vi "ControlProgram5.4.vi"() -> ()   [LabVIEW 2016]
uses:
  <vilib>/Utility/error.llb/DialogType.ctl
  <vilib>/Utility/miscctls.llb/LVPoint32TypeDef.ctl
  <vilib>/DAQmx/write.llb/DAQmx Write (Digital Bool 1Line 1Point).vi
  <vilib>/DAQmx/create/channels.llb/DAQmx Create Channel (DO-Digital Output).vi
  <vilib>/platform/TimedLoop/XDataNode/XDataNode.xnode
  <vilib>/Platform/TimedLoop/XDataNode/nitl_modes.ctl
  <vilib>/Platform/TimedLoop/XDataNode/XDNodeRunTimeDep.lvlib
  <vilib>/Platform/TimedLoop/XDataNode/wakeup.ctl
  <vilib>/Platform/TimedLoop/XDataNode/timing_clust.ctl
  <vilib>/DAQmx/create/channels.llb/DAQmx Create Channel (AI-Voltage-Basic).vi
  <vilib>/DAQmx/create/channels.llb/DAQmx Create Channel (AO-Voltage-Basic).vi
  <vilib>/DAQmx/write.llb/DAQmx Write (Analog 1D DBL NChan 1Samp).vi
  <resource>/objmgr/daqmx.rc
  <vilib>/Analysis/NI_AALBase.lvlib
  <vilib>/Analysis/baseanly.llb/Mean (DBL).vi
  <vilib>/Instr/_visa.llb/VISA Configure Serial Port (Instr).vi
  <vilib>/DAQmx/read.llb/DAQmx Read (Analog 2D DBL NChan NSamp).vi
  <vilib>/Utility/inputDevices.llb/closeMouse.vi
  <vilib>/Utility/inputDevices.llb/mouseAcquire.vi
  <vilib>/DAQmx/configure/timing.llb/DAQmx Timing (Sample Clock).vi
panel:
  out "Flush Sample Start Time":u32=46318105
  out "Sample flush time (s)":dbl=60.0
  in  "Inject Sample":bool
  out "Chart Freq (Hz)":dbl=500.0
  out "Cal values":T1={"AX alpha"=672.9952101249002, "BX alpha"=822.8320399167465, "AX kappa"=0.3432739170419873, "BX kappa"=0.22087046979741862, "AX offset"=-0.002065833400375715, "BX offset"=0.010483360643544744, "AY alpha"=702.0654168010462, "BY alpha"=773.6701766674906, "AY kappa"=0.33643150106915, "BY kappa"=0.2444549177225145, "AY offset"=-0.1177594339643395, "BY offset"=0.06470506082263472}
  in  "Inject Pump 1":bool
  in  "Inject Pump 2":bool
  in  "Tab Control 2":T2(tab)
  in  "Force FB script":bool
  in  "Got ADig bead":bool
  in  "Move Cap. 2 (ADig Top)":bool
  in  "Dump beads":bool
  in  "Got DNA bead":bool
  in  "Flow on\ncap 2?":bool=TRUE
  in  "Flow on\ncap 1?":bool=TRUE
  in  "Flow on\ndump?":bool=TRUE
  in  "Delta after tether":dbl=3.2
  in  "TA Cancel Save?":bool
  in  "Min fish\ndelta (V)":dbl=2.8 min=0.0 max=10.0 step=0.1
  in  "Max fish\ndelta (V)":dbl=3.8 min=0.0 max=10.0 step=0.1
  in  "Fish Speed (ms)":i32=3000
  in  "Wait (ms)":i32=1500
  in  "# attempts":dbl=15.0
  in  "Cutoff force (pN)":dbl=5.0
  in  "Raster after\n tether?":bool=TRUE
  out "Tether":bool
  out "Attempt #":i32
  in  "Flow on\nwhile fish?":bool=TRUE
  in  "Flow on\nafter raster?":bool=TRUE
  in  "Offset @ Delta (V)":dbl=4.0
  in  "Cal @ Delta (V)":dbl=5.0
  in  "Cal stage position":i32=3
  in  "Conv Y (nm/V)":dbl=505.7
  in  "Conv X (nm/V)":dbl=891.5
  out "Cal Final Sampling Rate":dbl=125000.0
  in  "Cal Averaging":i32=1
  in  "Wait before dip (s)":dbl=3.0
  in  "Start dipping after?":bool
  in  "Start trap delta (V)":dbl=3.85
  in  "Cancel dwell":bool
  in  "Pause dwell":bool
  in  "Return position":dbl=3.0
  in  "Dip duration":dbl=15.0
  in  "Dip position":dbl=4.0
  in  "Dip":bool
  out "Dip time":i32
  in  "Stop":bool=TRUE
  in  "?":T3(tab)
  in  "Save N sets":bool
  in  "N sets":i32=200
  in  "Cal sets to save":i32=500
  in  "Reset data stream":bool
  out "Buffer Overflow":bool
  out "Stage moving":bool
  in  "Comment":string
  in  "Raster scan":bool
  out "Saving":bool
  in  "Save cal":bool
  in  "Save Data":bool
  in  "Stop saving":bool
  out "Calibrating":bool
  out "Progress":dbl(slide) scale=0.0..100.0
  in  "Read Cal":bool
  in  "Fish":bool
  in  "Averaging Number":i32=1250
  out "Final Sampling Rate":dbl=100.0
  in  "Trap position":cluster{"X":dbl, "Y":dbl}={"X"=6.4, "Y"=1.35}
  in  "Trap delta":dbl=5.0 min=0.0 max=10.0 step=0.1
  in  "Fixed X":dbl=1.4
  in  "Fixed Y":dbl=1.35
  in  "Shutter 1 (B)":bool=TRUE
  in  "Shutter 2 (A)":bool=TRUE
  in  "Pulling direction":bool
  out "Raster scanning...":bool
  out "Current file name":path=path "D:/data/151111/151111_000.dat"
  in  "AX alpha":dbl=672.9952101249002 format="%#_3p"
  in  "BX alpha":dbl=822.8320399167465 format="%#_3g"
  in  "AX kappa":dbl=0.3432739170419873 format="%#_3g"
  in  "BX kappa":dbl=0.22087046979741862 format="%#_3g"
  in  "AX offset":dbl=-0.002065833400375715 format="%#_3g"
  in  "BX offset":dbl=0.010483360643544744 format="%#_3g"
  in  "AY alpha":dbl=702.0654168010462 format="%#_3g"
  in  "BY alpha":dbl=773.6701766674906 format="%#_3g"
  in  "AY kappa":dbl=0.33643150106915 format="%#_3g"
  in  "BY kappa":dbl=0.2444549177225145 format="%#_3g"
  in  "AY offset":dbl=-0.1177594339643395 format="%#_3g"
  in  "BY offset":dbl=0.06470506082263472 format="%#_3g"
  out "Buffer status":u8(slide) scale=0.0..100.0
  in  "dump spot":string="Dump beads spot"
  in  "up flow spot":string="Upper flow spot"
  in  "low flow spot":string="Lower flow spot"
  in  "up cap":string="Upper capillary (ADig beads)"
  in  "bottom cap":string="Lower capillary (DNA beads)"
  in  "Move to Position 5":bool
  in  "Set Position 5":bool
  in  "Saved stage positions":dbl[][](array[numeric])=[[1.0, 0.0, 0.0, 0.0], [2.0, -0.10561, -3.22524, -0.0041], [3.0, 0.5, -0.73974, 0.0], [4.0, 0.5, -2.1978, 0.0], [5.0, 0.5, -2.63158, -0.02256]]
  in  "Set Position 2":bool
  in  "Move to Position 2":bool
  in  "Set Position 1":bool
  in  "Move to Position 1":bool
  in  "Set Position 4":bool
  in  "Move to Position 4":bool
  in  "Set Position 3":bool
  in  "Move to Position 3":bool
  out "Stage error":errorcluster
  in  "Clear Volume":bool
  out "Sample Flush Meter":u8(slide) scale=0.0..100.0
  out "Flushing Sample":bool
  in  "Flush Sample":bool
  in  "Normal \nRate (ul/hr)  3":dbl=100.0
  in  "Normal \nVolume (ul) 3":dbl=400.0
  in  "Normal \nVolume (ul) 2":dbl
  in  "Normal \nRate (ul/hr)":dbl
  in  "Normal \nVolume (ul)":dbl
  in  "Flush\nRate (ul/min)":dbl
  in  "Flush\nVolume (ul)":dbl
  in  "Flush \nRate (ul/min)  2":dbl
  in  "Flush Pump 2":bool
  in  "Flush\nVolume (ul)  2":dbl
  in  "Flush Pump 1":bool
  in  "Normal \nRate (ul/hr)  2":dbl
  in  "Write Wait":i32=1000
  in  "Flush \nRate (ul/min)  3":dbl=100.0
  in  "Flush\nVolume (ul)  3":dbl=100.0
  out "error out":errorcluster
  in  "Use Mouse to Move Trap?":bool
  in  "Pause Mouse/Mirror Connection":bool
  out "Reference Voltage":cluster{dbl, dbl}={0.0, -0.0}
  out "Saved voltage":cluster{dbl, dbl}={5.766666666666665, 1.45}
  out "Real Coordinates":cluster{"Horizontal":i32, "Vertical":i32}={"Horizontal"=897, "Vertical"=-1271}
  out "CoordinatesMousePressed":T4
  out "Sum error":dbl(knob) scale=-1.0..1.0
  out "Trap sep":waveform(dbl)[](graph)=[{"t0"=timestamp(11.689999999999795 s since 1904-01-01), "dt"=0.002, "Y"=[4456.58918693872, 4456.558162103858, 4456.805211715709, 4456.946547075299, 4456.750056453253], "attributes"=variant("NI_ChannelName"=variant(string "T2 X"))}, {"t0"=timestamp(11.689999999999795 s since 1904-01-01), "dt"=0.002, "Y"=[3.6580154856012372, 3.6801758901442225, 3.6782205603924463, 3.7068987310363912, 3.7544784232311184], "attributes"=variant("NI_ChannelName"=variant(string "T2 Y"))}]
  in  "Set reading to\nsetpoint":bool
  in  "Offset Y (nm)":dbl format="%0.2f"
  in  "Offset X (nm)":dbl format="%0.2f"
  in  "Remove offsets":bool
  in  "Force Feedback":bool
  out "Feedback Output Voltage 2":cluster{dbl, dbl} {"?" format="%#_4g"; "?" format="%#_4g"}
  in  "Max value X":dbl=10.0 format="%.1f"
  in  "Min value X":dbl format="%0.1f"
  in  "Max value Y":dbl=10.0 format="%.1f"
  in  "Min value Y":dbl format="%.1g"
  in  "Offset":cluster{"Off Y":dbl, "Off X":dbl}={"Off Y"=1.5, "Off X"=0.17}
  in  "Setpoint voltage":cluster{"SP Y":dbl, "SP X":dbl}={"SP Y"=0.6, "SP X"=0.0}
  in  "Feedback const":T5={"Ki_B_Y"=0.5, "Ki_B_X"=0.0, "Kp Y"=1.0, "Kp X"=0.0}
  out "Mean Trap Pos X 2 (nm)":dbl=4456.729832857368 format="%0.2f"
  out "Mean Trp Pos Y 2 (nm)":dbl=3.6955578180810833 format="%0.2f"
  out "T2 X RMS (A)":dbl=1.4304414731965482 format="%0.2f"
  out "T2 Y RMS (A)":dbl=0.33307251334057864 format="%0.2f"
  in  "Scan range (nm)":dbl=500.0
  in  "Scan speed (nm/s)":dbl=100.0 min=0.0 max=100.0
  in  "Step size (nm)":dbl=1.0
  in  "Save scans":bool=TRUE
  in  "# scans":i32=1
  in  "Load param":bool
  in  "Scan Parameters":T6(array[cluster])=[{"Label"="Offset", "Max delta 2"=3.8, "Start delta 2"=2.4, "Speed (ms) 2"=10000, "# scans 2"=1}]
  in  "Trap delta\nafter":dbl=3.6
  in  "Stop raster":bool
  out "Scan range (V)":dbl=0.5608524957936063
  out "Scan steps (mirror)":u64=500
  out "Scan increment (V)":dbl=0.0011217049915872126
  out "Time per step (ms)":dbl=10.0
  out "Total raster time (s)":dbl=10.0
  out "N sets to be saved":dbl=1000.0
  out "Continue to display?":bool
  out "Video Error":errorcluster
  in  "# Samples/channel (in)":i32=40000 format="%.2f"
  out "Buffer size\n(Samples/channel)":u32=511
  out "DAQ rate\n(Samples/s)":dbl=125000.0 format="%#_6p"
  out "# Samples/channel":i32=1250
  out "# Samples/channel/s":dbl=100.0
  out "AvailSampPerChan":u32=6
  out "Data update period (s/set)":dbl=0.01 format="%#_6p"
  out "AvailSampPerChan 2":u32=81
  in  "PC samp per channel":i32=1000
  in  "Sampling Rate":dbl=125000.0 format="%0.0p"
  in  "DAQ Rate2":dbl=1000000.0 format="%#_6p"
  out "Data period (s)":dbl=8e-06 format="%#_6p"
  in  "Tether break\nforce (pN)":dbl=1.0
  in  "Path":path=path "D:/data"
  in  "Save file index":dbl
  out "Mirror task":refnum<k21>
  in  "HWP1":string="Half waveplate 1: differential trap power"
  in  "HWP0":string="Half waveplate 0: total trap power"
  in  "Move 1":bool
  in  "\"Degrees\" 1":dbl
  in  "Move 0":bool
  in  "\"Degrees\" 0":dbl
  out "Chamber":T7(plugin-control)
  out "Deflection":T4
  in  "Sampling Rate":dbl=125000.0 format="%0.2f"
  in  "Averaging Number":i32=12500
  in  "DAQ Rate":dbl=1000000.0
  out "Final Sampling Rate":dbl
  in  "Tab Control":T8(tab)
  in  "Downsamp\nfact":dbl=250.0
  out "Bead sep":waveform(dbl)[](graph)=[{"t0"=timestamp(11.689999999999795 s since 1904-01-01), "dt"=0.002, "Y"=[63.31490687968469, 63.634813997558965, 62.7925550739979, 64.07278834927408, 63.99586325693618], "attributes"=variant("NI_ChannelName"=variant(string "T2"))}, {"t0"=timestamp(11.689999999999795 s since 1904-01-01), "dt"=0.002, "Y"=[176.64692461381742, 177.9358681148926, 177.1161917603868, 176.2271334264959, 177.42702158777735], "attributes"=variant("NI_ChannelName"=variant(string "T1"))}]
  out "Force (pN)":waveform(dbl)[](graph)=[{"t0"=timestamp(11.689999999999795 s since 1904-01-01), "dt"=0.002, "Y"=[21.359049199870693, 21.47379015932484, 21.184451058658276, 21.619260543462246, 21.59231529352076], "attributes"=variant("NI_ChannelName"=variant(string "T2"))}, {"t0"=timestamp(11.689999999999795 s since 1904-01-01), "dt"=0.002, "Y"=[41.69409117180523, 41.983023709759294, 41.835566815034625, 41.592717375287485, 41.869370537040446], "attributes"=variant("NI_ChannelName"=variant(string "T1"))}]
  out "Mean force (pN)":dbl=31.62036358637639 format="%0.2f"
  out "Force noise (pN)":dbl=0.0949326369135985 format="%0.2f"
  out "Mean Bead Sep\n(nm)":dbl=120.31640670608219 format="%0.2f"
  out "Bead Sep Noise\n(A)":dbl=3.5979970492756337 format="%0.2f"
  out "PSD 2":cluster{dbl[], dbl[]}(graph)
  out "PSD 1":cluster{dbl[], dbl[]}(graph)
  out "PSD 1 Sum":dbl(slide) scale=0.0..10.0
  out "PSD 2 Sum":dbl(slide) scale=0.0..10.0
  in  "Start":bool
  out "All signals":waveform(dbl)[](graph)=[{"t0"=timestamp(11.689999999999795 s since 1904-01-01), "dt"=0.002, "Y"=[-1.299883075629171, -1.2973358725298367, -1.2936816089521828, -1.3024318472699856, -1.301891455018789], "attributes"=variant("NI_ChannelName"=variant(string "A y"))}, {"t0"=timestamp(11.689999999999795 s since 1904-01-01), "dt"=0.002, "Y"=[-0.23397256158648597, -0.24766722604162583, -0.2351063720288359, -0.2449917640631612, -0.24277750809631515], "attributes"=variant("NI_ChannelName"=variant(string "A x"))}, {"t0"=timestamp(11.689999999999795 s since 1904-01-01), "dt"=0.002, "Y"=[-0.7474367183534977, -0.752021809613988, -0.7569647451326695, -0.7437660589687638, -0.7496079628534502], "attributes"=variant("NI_ChannelName"=variant(string "B y"))}, {"t0"=timestamp(11.689999999999795 s since 1904-01-01), "dt"=0.002, "Y"=[-0.7679815477569002, -0.7778056271968022, -0.7612590927024251, -0.7662199857579963, -0.7730989233960032], "attributes"=variant("NI_ChannelName"=variant(string "B x"))}, {"t0"=timestamp(11.689999999999795 s since 1904-01-01), "dt"=0.002, "Y"=[6.442881382091263, 6.440977653300508, 6.439989054505619, 6.439557267869424, 6.436601783511025], "attributes"=variant("NI_ChannelName"=variant(string "A sum"))}, {"t0"=timestamp(11.689999999999795 s since 1904-01-01), "dt"=0.002, "Y"=[6.405386825078533, 6.40147238948137, 6.401793329117672, 6.401977644095232, 6.397063010213611], "attributes"=variant("NI_ChannelName"=variant(string "B sum"))}, {"t0"=timestamp(11.689999999999795 s since 1904-01-01), "dt"=0.002, "Y"=[6.3989783364427595, 6.3989435357306315, 6.399220652513415, 6.399379189091754, 6.399158784580205], "attributes"=variant("NI_ChannelName"=variant(string "Trap x"))}, {"t0"=timestamp(11.689999999999795 s since 1904-01-01), "dt"=0.002, "Y"=[1.3572335682926662, 1.3572773895395378, 1.3572735229590518, 1.357330232808061, 1.3574243196029883], "attributes"=variant("NI_ChannelName"=variant(string "Trap y"))}]
  # "Bead Calibration"
  # "X"
  # "Y"
  # "Pump #1 Controls"
  # "Pump #2 Controls"
  # "Sample Pump Controls"
  # "Retract the pumps manually. Change it back to INFUSE when you're done. Suck it up, don't whine."
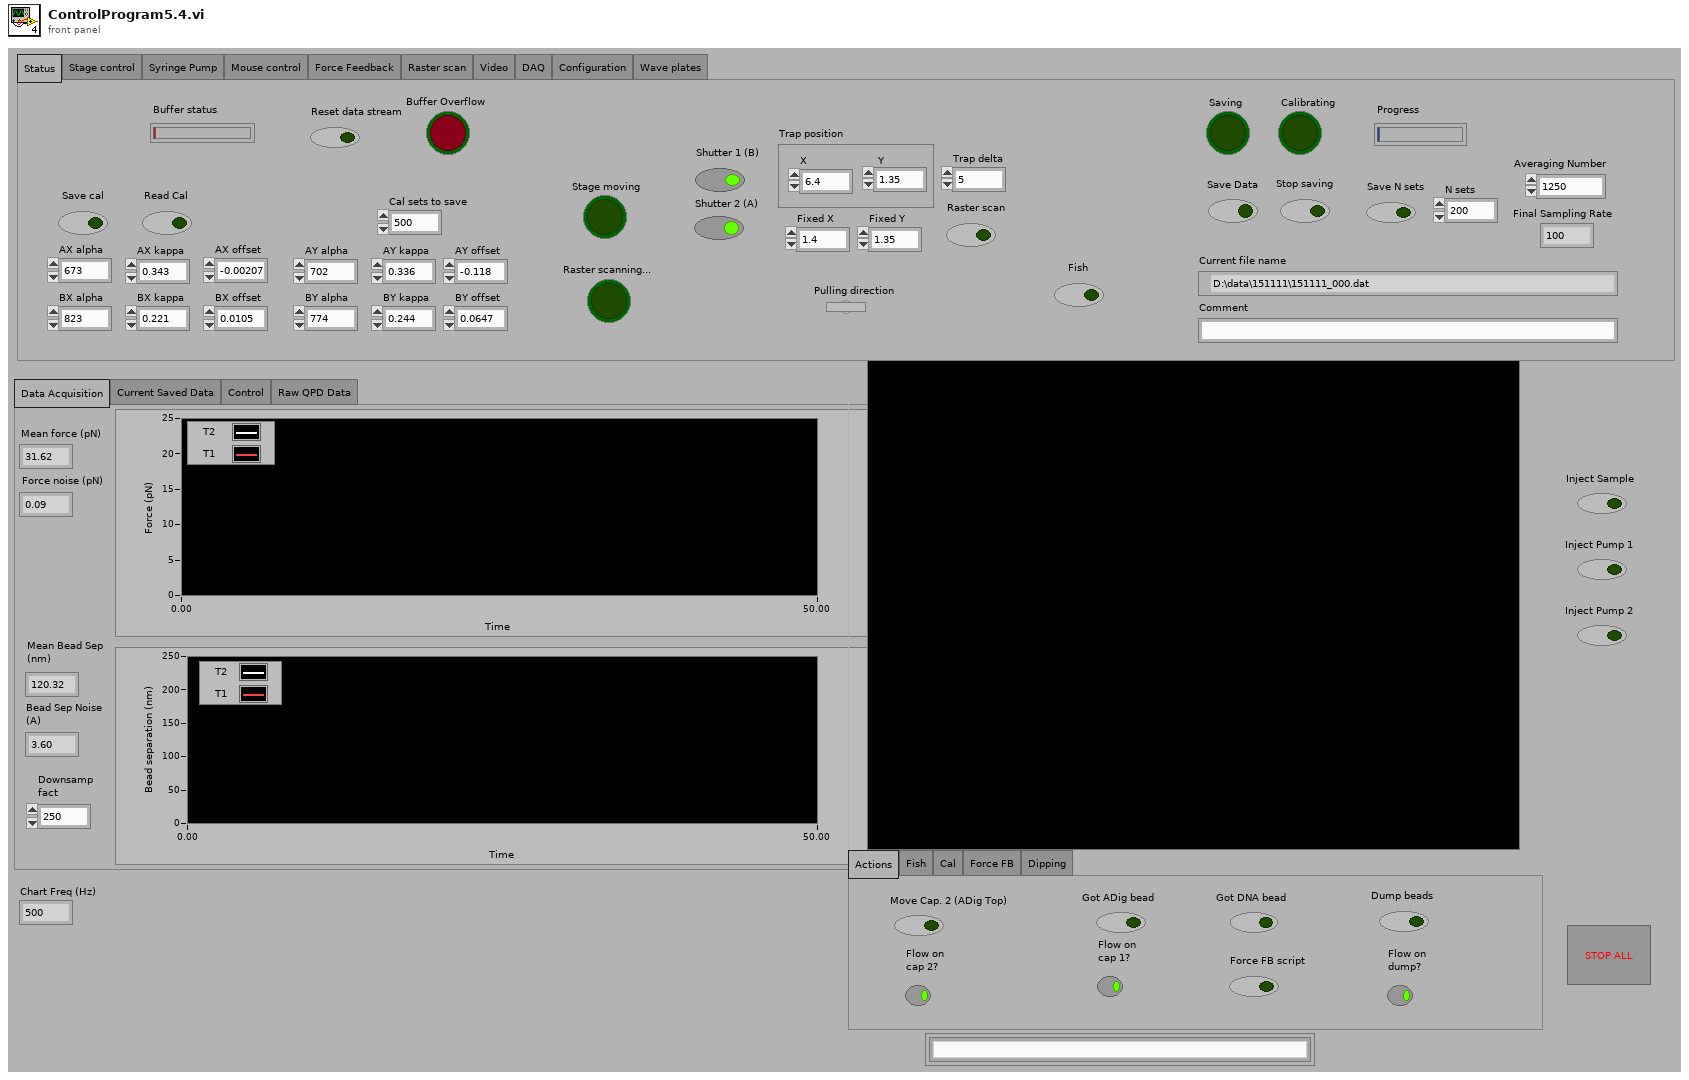
[diagram p1: front panel]
types:
  T1 = cluster{"AX alpha":dbl, "BX alpha":dbl, "AX kappa":dbl, "BX kappa":dbl, "AX offset":dbl, "BX offset":dbl, "AY alpha":dbl, "BY alpha":dbl, "AY kappa":dbl, "BY kappa":dbl, "AY offset":dbl, "BY offset":dbl}
  T2 = enum32{"Actions", "Fish", "Cal", "Force FB", "Dipping"}
  T3 = enum32{"Status", "Stage control", "Syringe Pump", "Mouse control", "Force Feedback", "Raster scan", "Video", "DAQ", "Configuration", "Wave plates"}
  T4 = typedef "LVPoint32TypeDef.ctl" = cluster{"Horizontal":i32, "Vertical":i32}
  T5 = cluster{"Ki_B_Y":dbl, "Ki_B_X":dbl, "Kp Y":dbl, "Kp X":dbl}
  T6 = cluster{"Label":string, "Max delta 2":dbl, "Start delta 2":dbl, "Speed (ms) 2":i32, "# scans 2":i32}[]
  T7 = typedef "IMAQ Image.ctl" = refnum<image>
  T8 = enum32{"Data Acquisition", "Current Saved Data", "Control", "Raw QPD Data"}
  T9 = enum16{"open", "replace", "create", "open or create", "replace or create", "replace or create with confirmation"}
  T10 = enum16{"big-endian, network order", "native, host order", "little-endian"}
  T11 = cluster{string, string, string, string, string, string, string, string}
  T12 = typedef "XDNodeRunTimeDep.lvlib/timing_clust.ctl" = cluster{"Expected End [f-1]":u64, "Actual End [f-1]":u64, "Finished Late? [f-1]":bool, "Expected End [i-1]":u64, "Actual End [i-1]":u64, "Finished Late? [i-1]":bool, "Expected Start [i]":u64, "Actual Start [i]":u64, "Expected Start [f]":u64, "Actual Start [f]":u64, "Source Name":string, "Structure Name":string, "Period":i64, "Deadline":i64, "Offset":i64, "Start":i64, "Priority":i32, "Timeout":i32, "Mode":T13, "Wakeup Reason":T14, "Error":errorcluster, "Source Type":string, "Secondary Source Type":string, "Global End Time":u64, "Global Start Time":u64, "Frame Duration":u64, "Iteration Duration":u64, "Assigned CPU":i32, "I/O Scan Engine Mode":u32}
  T13 = typedef "XDNodeRunTimeDep.lvlib/nitl_modes.ctl" = enum32{"No Change", "Process missed periods, maintain original phase", "Discard missed periods, maintain original phase", "Process missed periods, ignore original phase", "Discard missed periods, ignore original phase"}
  T14 = typedef "XDNodeRunTimeDep.lvlib/wakeup.ctl" = enum32{"Normal", "Aborted", "Asynchronous wakeup", "Timing source error", "Timed loop error", "Timeout"}
  T15 = typedef "DialogType.ctl" = u16
  T16 = cluster{"button 1":bool, "button 2":bool, "button 3":bool, "button 4":bool}
  T17 = cluster{"[0]":dbl, "[1]":dbl, "[2]":dbl, "[3]":dbl, "[4]":dbl, "[5]":dbl, "[6]":dbl, "[7]":dbl, "[8]":dbl, "[9]":dbl, "[10]":dbl, "[11]":dbl}
  T18 = cluster{"Label":string, "Max delta 2":dbl, "Start delta 2":dbl, "Speed (ms) 2":i32, "# scans 2":i32}
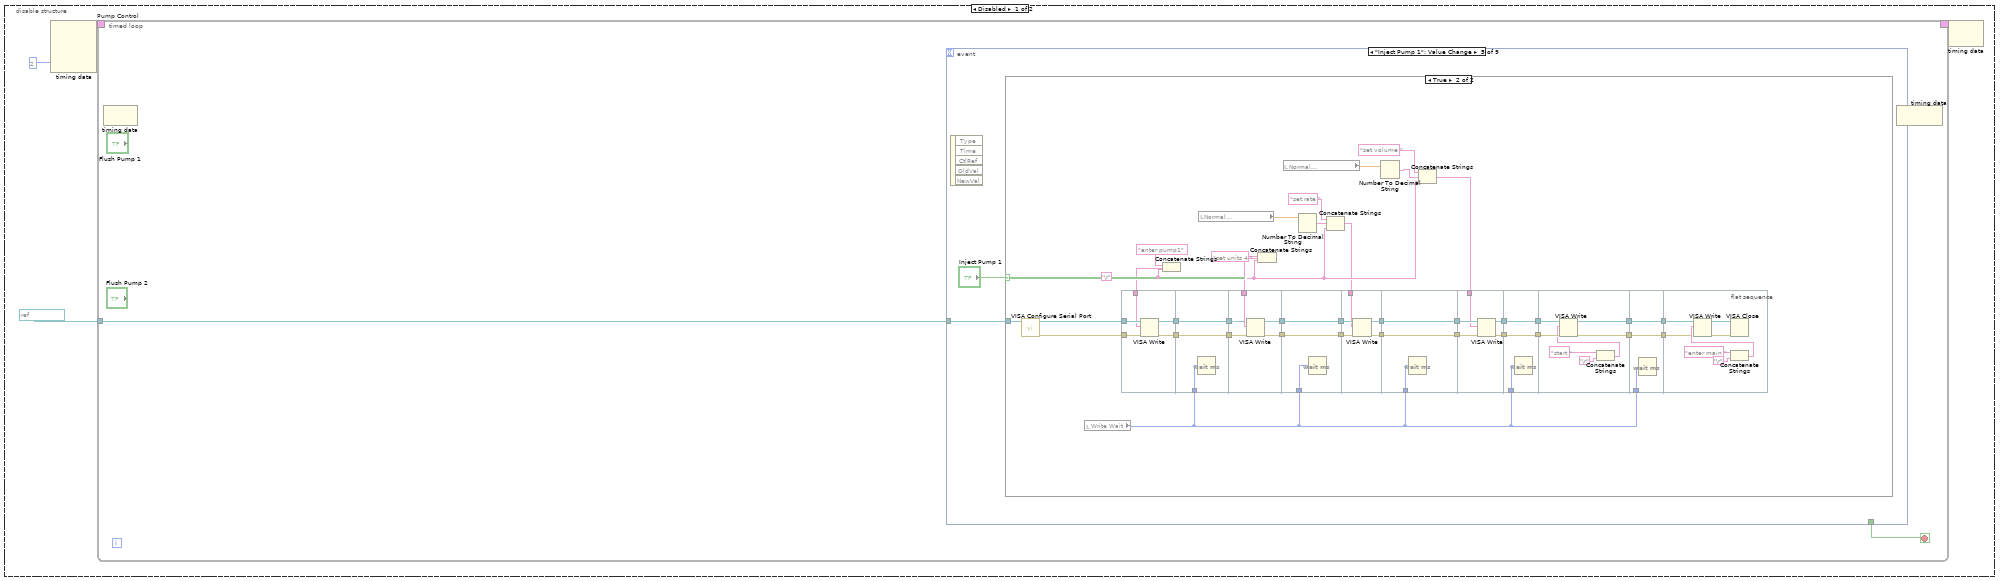
[diagram p2: hidden frame]
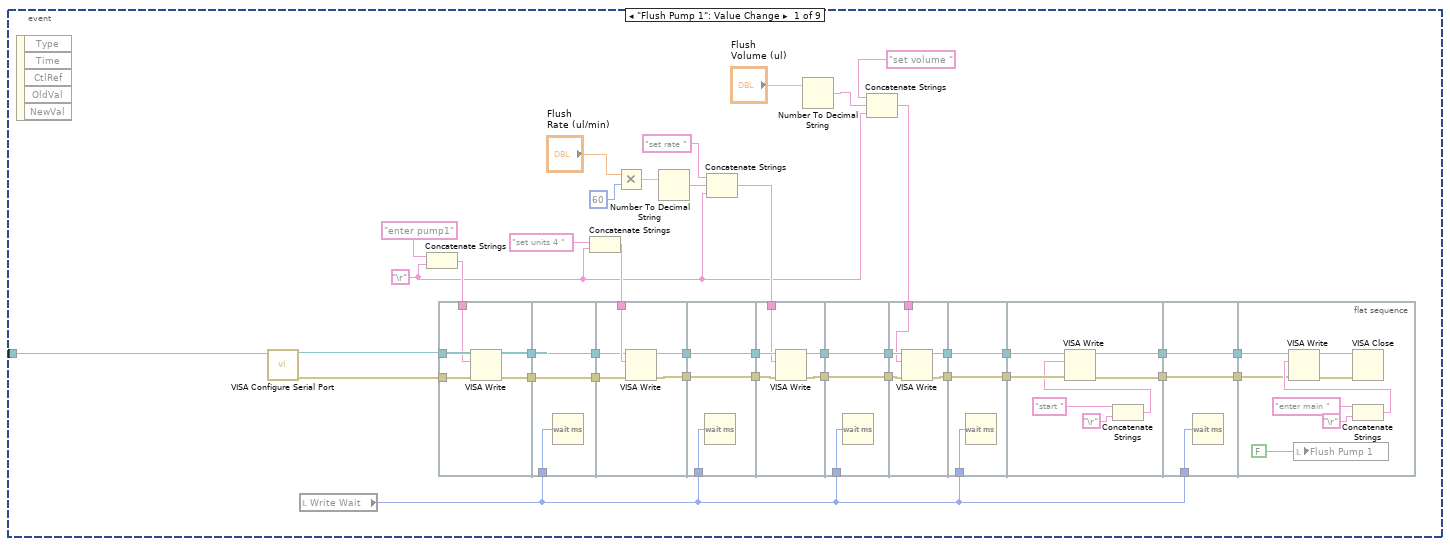
[diagram p3: hidden frame]
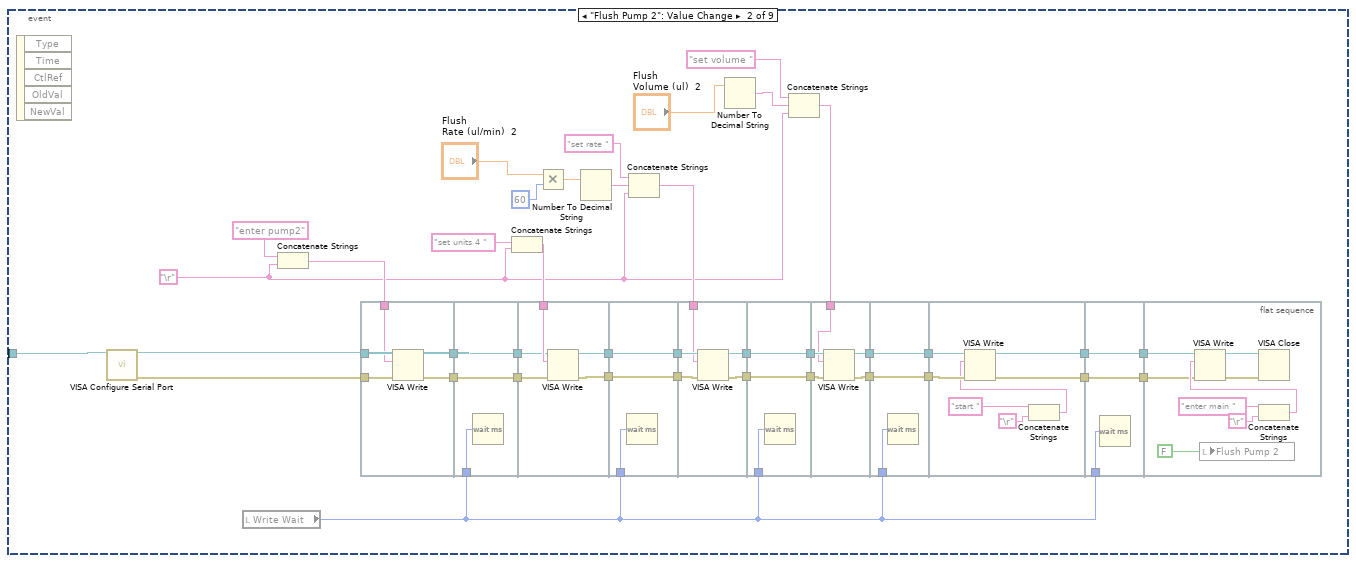
[diagram p4: hidden frame]
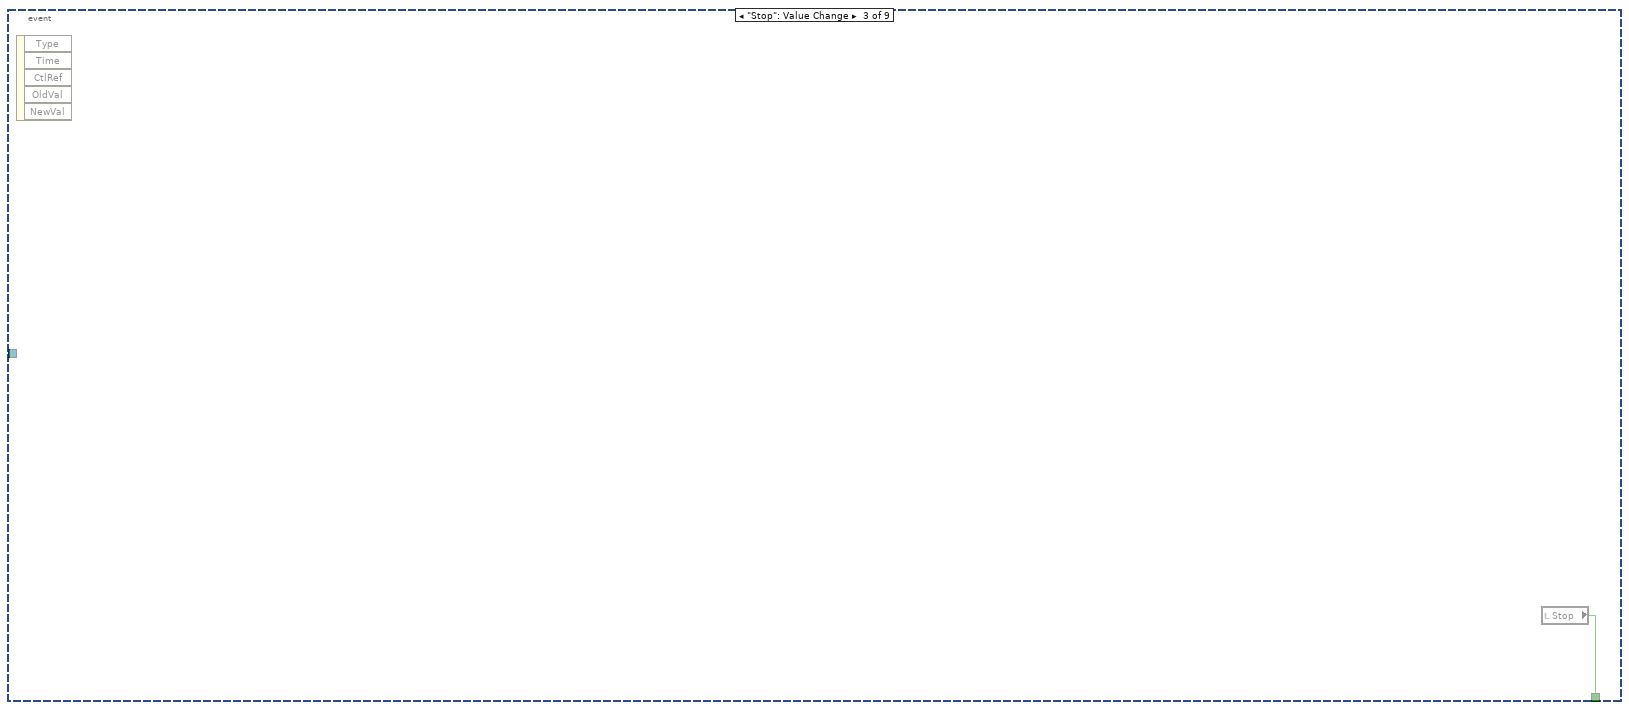
[diagram p5: hidden frame]
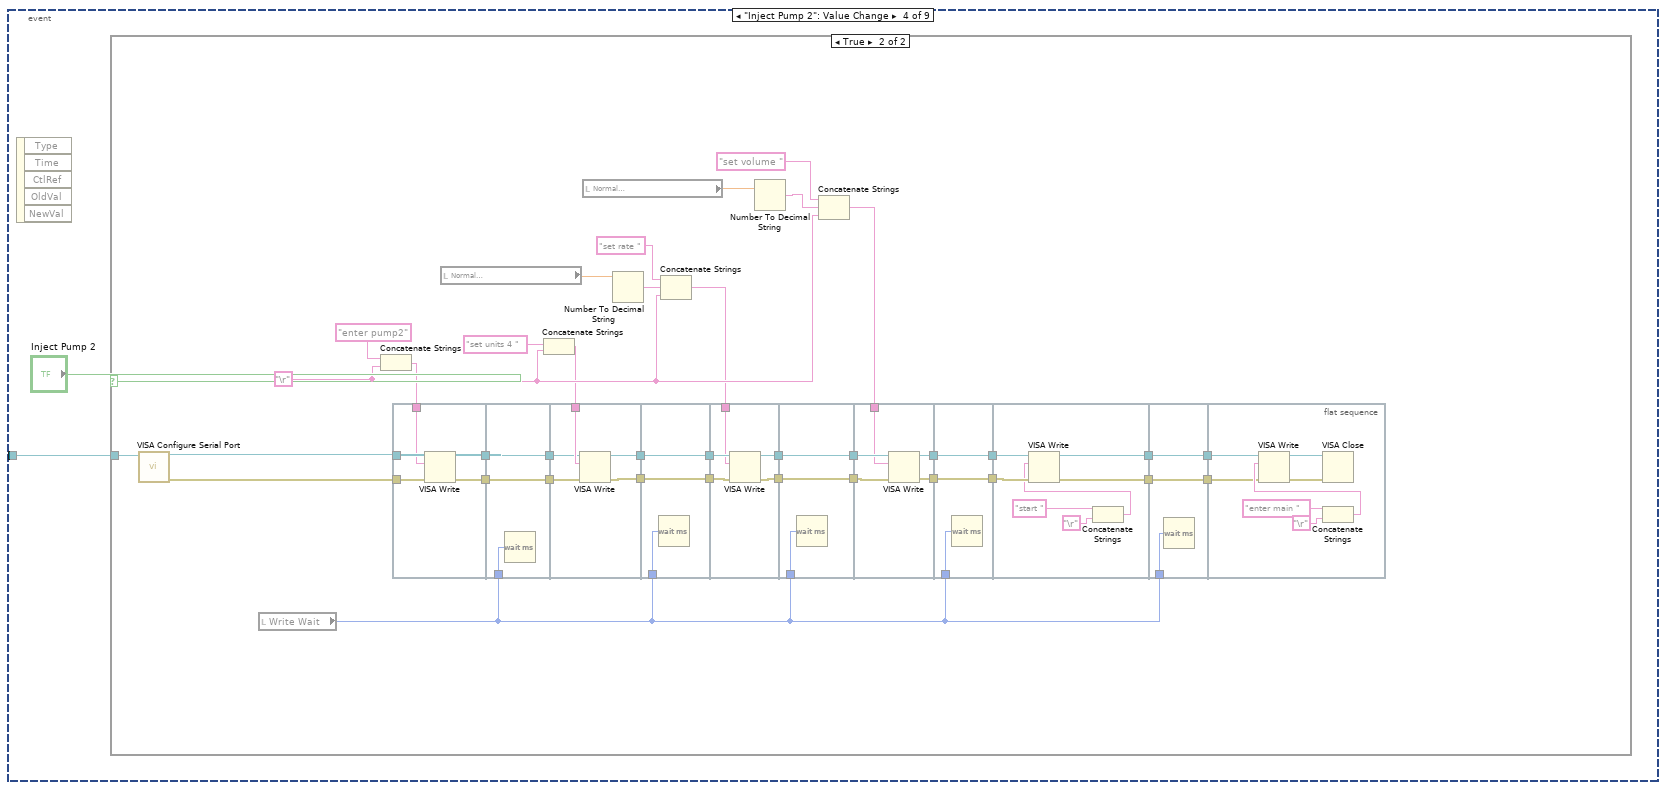
[diagram p6: hidden frame]
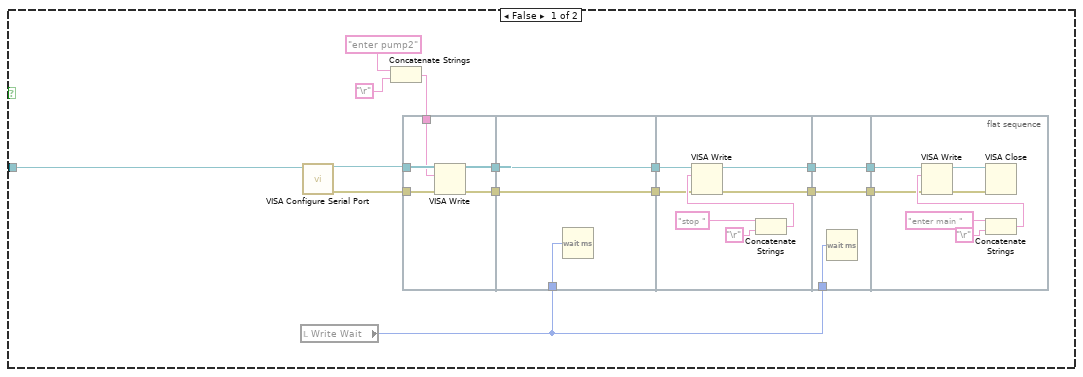
[diagram p7: hidden frame]
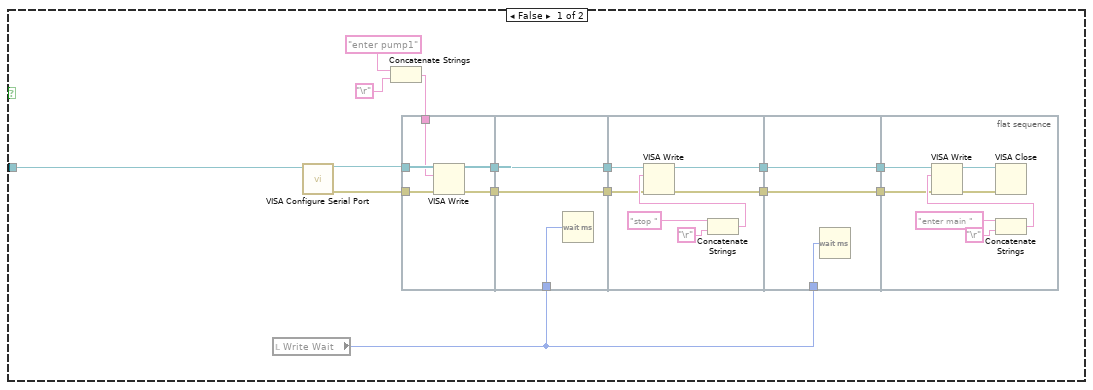
[diagram p8: hidden frame]
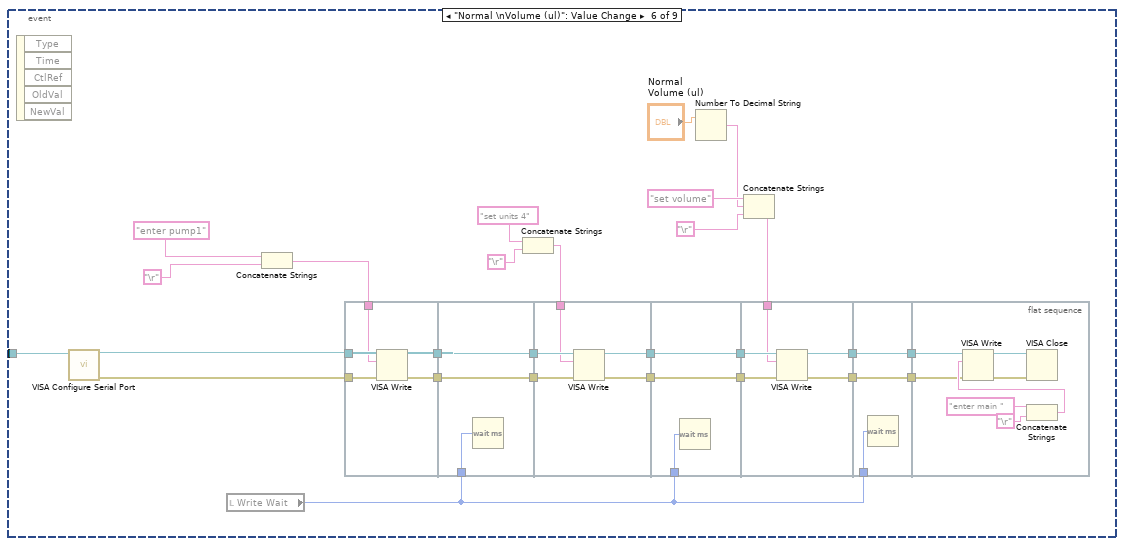
[diagram p9: hidden frame]
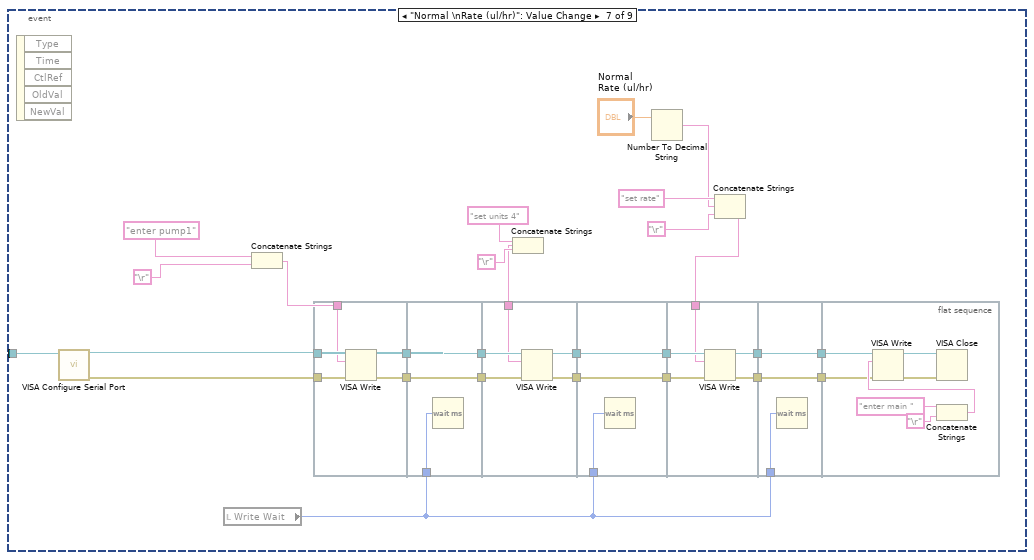
[diagram p10: hidden frame]
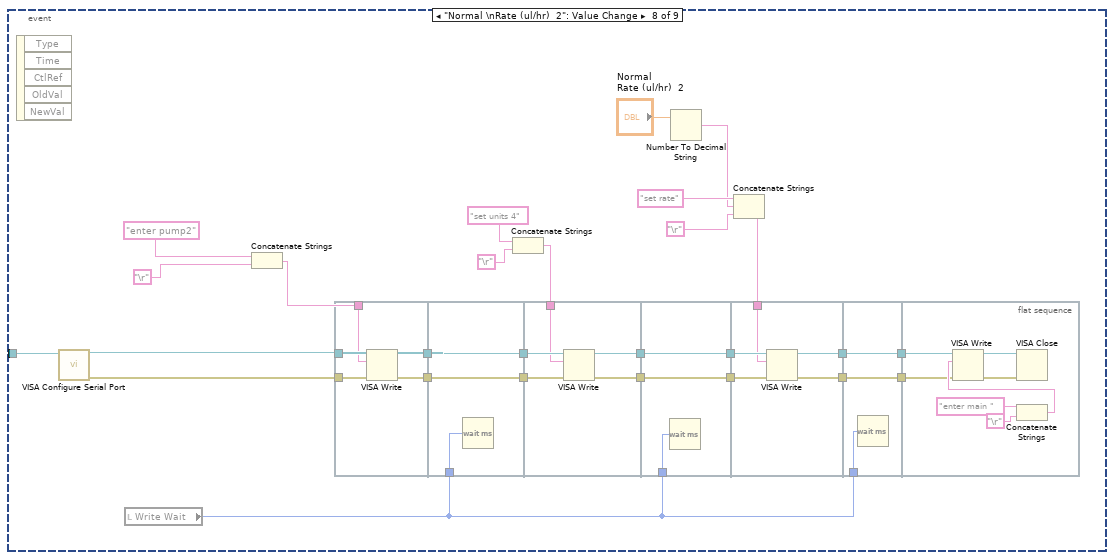
[diagram p11: hidden frame]
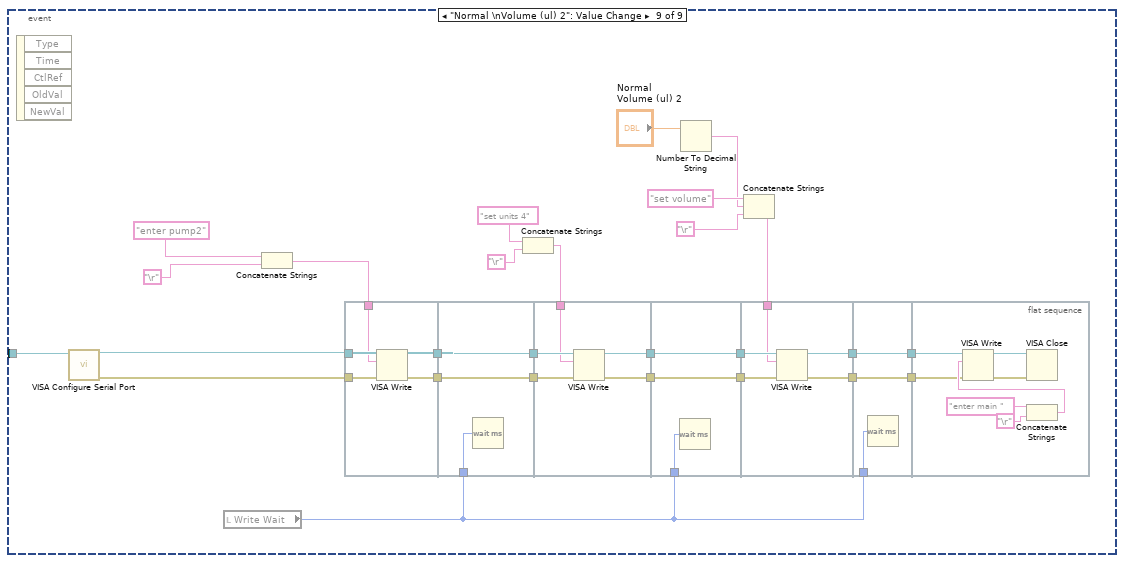
[diagram p12: hidden frame]
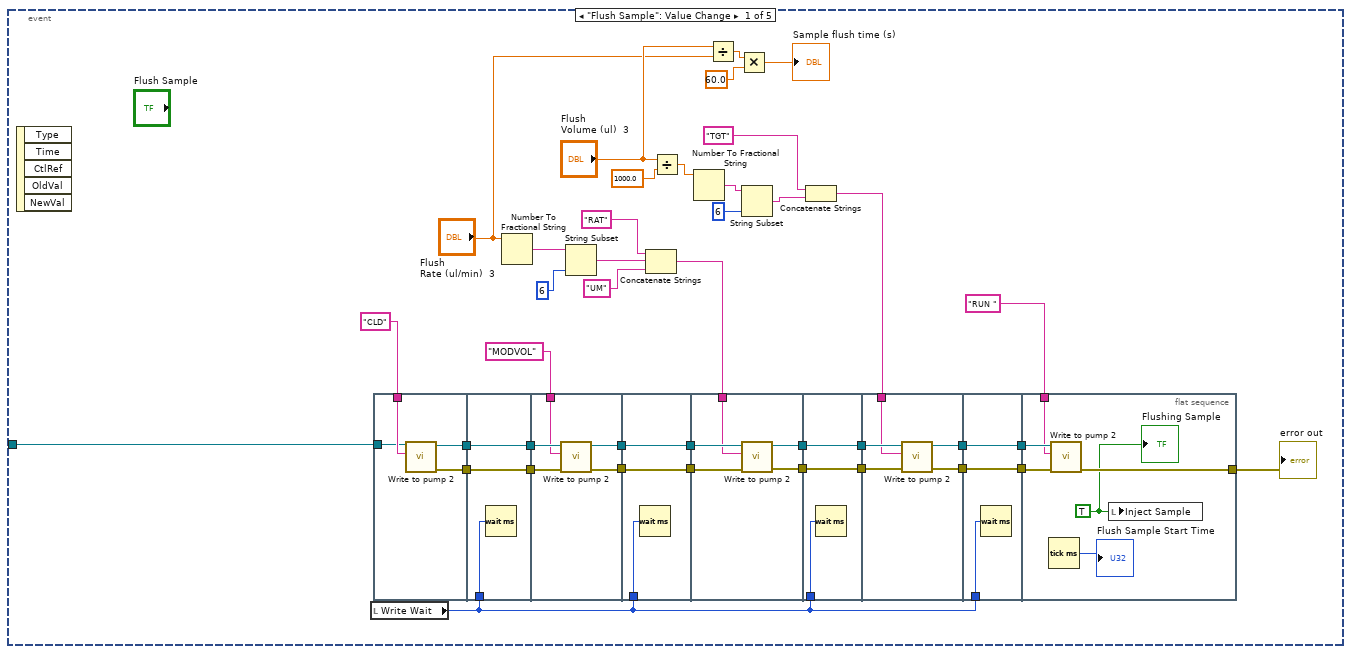
[diagram p13: hidden frame]
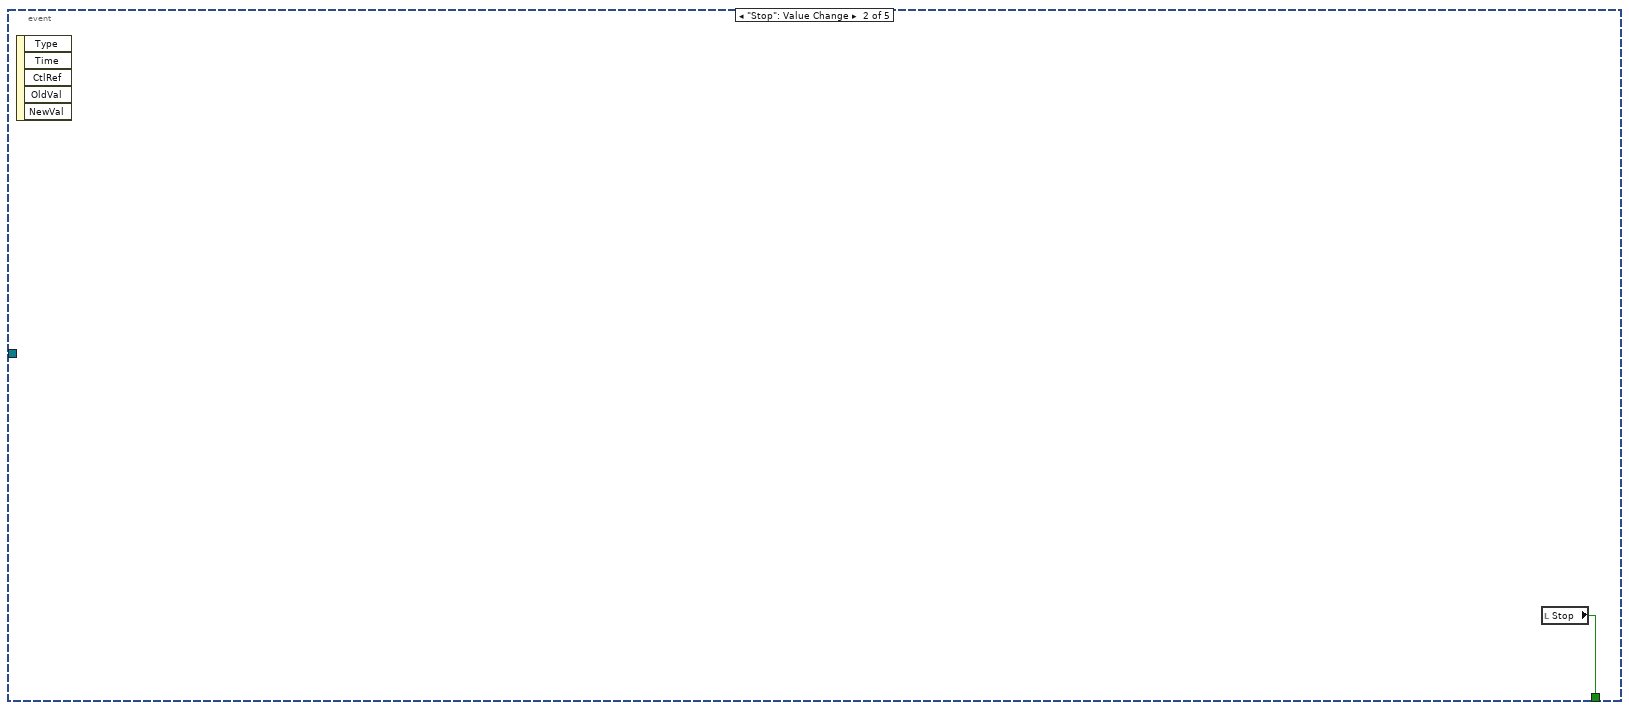
[diagram p14: hidden frame]
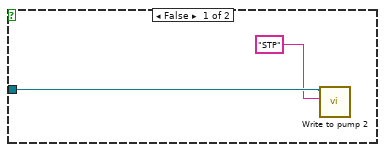
[diagram p15: hidden frame]
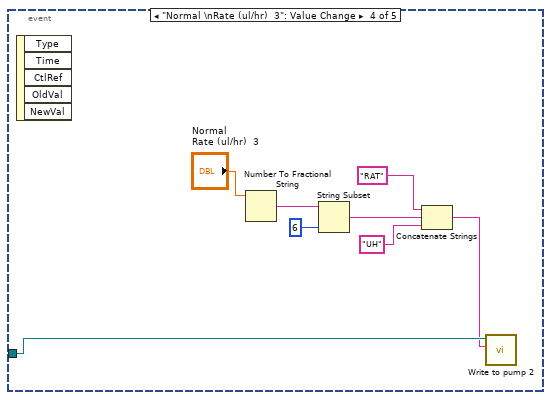
[diagram p16: hidden frame]
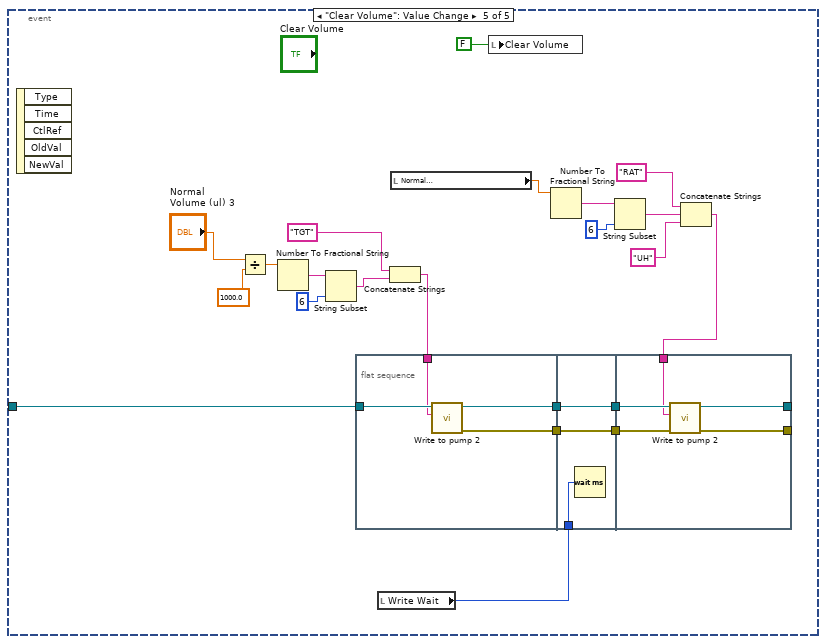
[diagram p17: hidden frame]
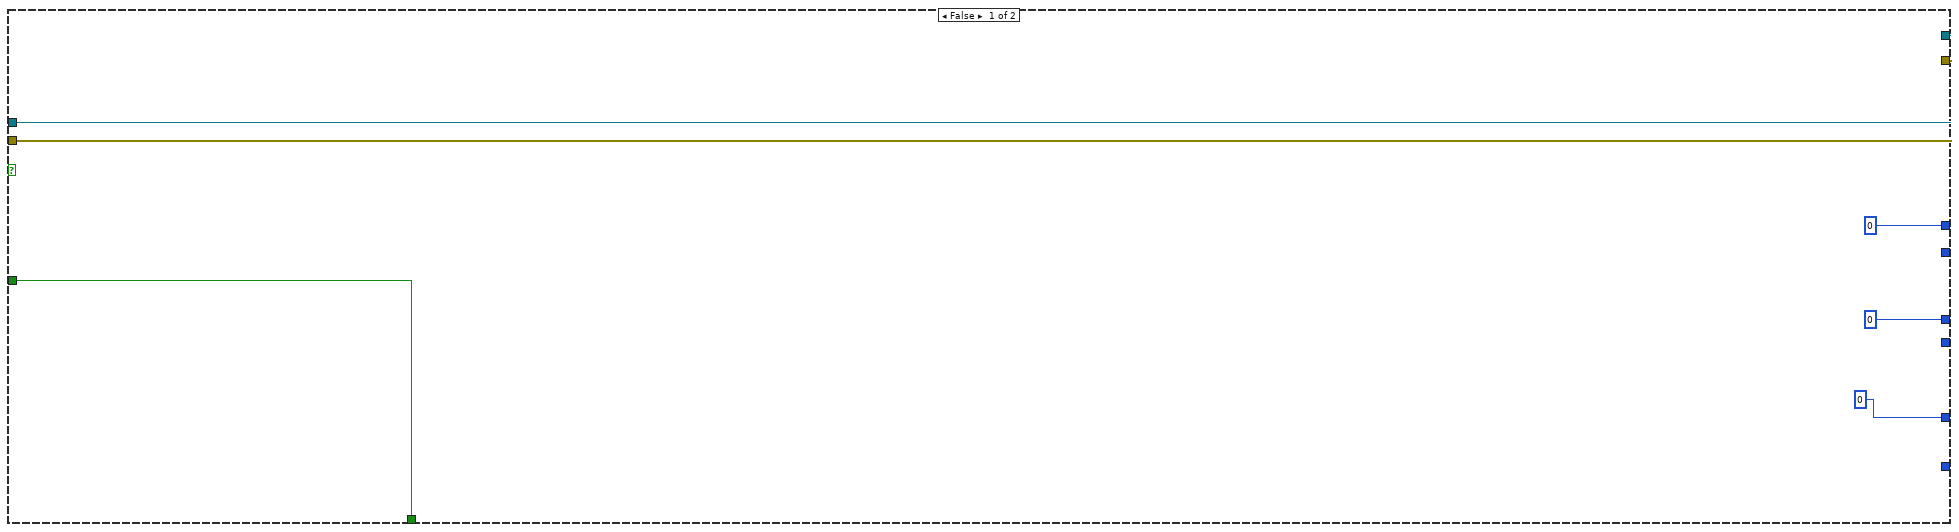
[diagram p18: hidden frame]
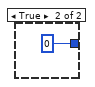
[diagram p19: hidden frame]
diagram:
  w42 = 10.0 ("Minimum Value")
  w43 = -10.0 ("Minimum Value")
  w45 = -2.0 ("Minimum Value")
  w46 = 2.0 ("Maximum Value")
  w71 = 10123 items=["Finite Samples"=10178, "Continuous Samples"=10123] ("sample mode")
  w92 = tag "Dev1/port2/line1"  # Shutter 2
  w95 = tag "Dev1/port1/line4"  # Shutter 1
  # "Create channels for movable mirror"
  # "Create channels for detectors"
  n1 = call-poly <vilib>:"DAQmx Create Virtual Channel.vi"("maximum value"=w46, "minimum value"=w45, "physical channels"=tag "Dev1/ai0" ("Physical Channel")) -> ("task out"=w47:refnum<k21>, "error out"=w70:errorcluster)  [unwired: 11 in]
  n2 = call-poly <vilib>:"DAQmx Create Virtual Channel.vi"("task in"=w47, "maximum value"=w46, "minimum value"=w45, "physical channels"=tag "Dev1/ai1", "error in"=w70) -> ("task out"=w68:refnum<k21>, "error out"=w67:errorcluster)  [unwired: 9 in]
  n3 = call-poly <vilib>:"DAQmx Create Virtual Channel.vi"("task in"=w68, "maximum value"=w46, "minimum value"=w45, "physical channels"=tag "Dev1/ai2", "error in"=w67) -> ("task out"=w59:refnum<k21>, "error out"=w58:errorcluster)  [unwired: 9 in]
  n4 = call-poly <vilib>:"DAQmx Create Virtual Channel.vi"("task in"=w59, "maximum value"=w46, "minimum value"=w45, "physical channels"=tag "Dev1/ai3" ("Physical Channel"), "error in"=w58) -> ("task out"=w44:refnum<k21>, "error out"=w64:errorcluster)  [unwired: 9 in]
  n5 = call-poly <vilib>:"DAQmx Create Virtual Channel.vi"("task in"=w44, "maximum value"=w42, "minimum value"=w43, "physical channels"=tag "Dev1/ai4", "error in"=w64) -> ("task out"=w62:refnum<k21>, "error out"=w61:errorcluster)  [unwired: 9 in]
  n6 = call-poly <vilib>:"DAQmx Create Virtual Channel.vi"("task in"=w62, "maximum value"=w42, "minimum value"=w43, "physical channels"=tag "Dev1/ai5", "error in"=w61) -> ("task out"=w57:refnum<k21>, "error out"=w56:errorcluster)  [unwired: 9 in]
  n7 = call-poly <vilib>:"DAQmx Create Virtual Channel.vi"("task in"=w57, "maximum value"=w42, "minimum value"=w43, "physical channels"=tag "Dev1/ai6", "error in"=w56) -> ("task out"=w51:refnum<k21>, "error out"=w49:errorcluster)  [unwired: 9 in]
  n8 = call-poly <vilib>:"DAQmx Create Virtual Channel.vi"("task in"=w51, "maximum value"=w42, "minimum value"=w43, "physical channels"=tag "Dev1/ai7", "error in"=w49) -> ("task out"=w50:refnum<k21>, "error out"=w48:errorcluster)  [unwired: 9 in]
  n9 = call-poly <vilib>:"DAQmx Timing.vi"("task/channels in"=w50, "sample mode"=w71, "samples per channel"="PC samp per channel", "rate"="Sampling Rate", "error in"=w48) -> ("task out"=w54:refnum<k21>, "error out"=w53:errorcluster)  [unwired: 9 in]
  n10 = call-poly <vilib>:"DAQmx Create Virtual Channel.vi"("maximum value"="Max value Y", "minimum value"="Min value Y", "physical channels"=tag "Dev1/ao1" ("Trap X Axis")) -> ("task out"=w39:refnum<k21>, "error out"=w41:errorcluster)  [unwired: 11 in]
  n11 = property class="DAQmx Timing"(reference=w54, error in=w53, "More:AI Convert:Rate"="DAQ Rate2") -> (reference out=w6:refnum<k21>, error out=w5:errorcluster, "SampClk.Rate"=→"DAQ rate\n(Samples/s)":dbl)
  n12 = call-poly <vilib>:"DAQmx Create Virtual Channel.vi"("task in"=w39, "maximum value"="Max value X", "minimum value"="Min value X", "physical channels"=tag "Dev1/ao0" ("Trap Y Axis"), "error in"=w41) -> ("task out"=w30:refnum<k21>, "error out"=w29:errorcluster)  [unwired: 9 in]
  "Mirror task" <- w30
  n13 = property class="DAQmx Buffer"(reference=w6, error in=w5) -> (reference out=w3:refnum<k21>, error out=w2:errorcluster, "Input.OnbrdBufSize"=→"Buffer size\n(Samples/channel)":u32)
  n14 = call <vilib>:"DAQmx Start Task.vi"("task/channels in"=w3, "error in"=w2) -> ("task out"=w31:refnum<k21>)  [unwired: 12 in, 1 out]
  n15 = while {
    tunnel: [w123] -> w77
    tunnel: [w323] -> w78
    tunnel: [w121] -> w76
    tunnel: [w435] -> w73
    tunnel: w31 -> [w136]
    tunnel: w30 -> [w431]
    tunnel: w29 -> [w436]
    stop <- w435 stop-if-true
    w167 = "NI_ChannelName" ("name")
    w243 = -1
    # "Scan # counter"
    # "DAQ loop iteration\ncounter (for timing)"
    # "Step counter"
    # "Force feedback"
    # "Raster scan"
    # "Rewire everything"
    # "Invert these because changed\nfrom PSD to QPD"
    # "Trap Y"
    # "Trap X"
    # "Convert to\npN"
    # "Convert to\nnm"
    # "Subtract\noffset"
    # "Normalize by\nsum"
    # "B sum"
    # "BX"
    # "BY"
    # "AX"
    # "AY"
    # "A sum"
    # "Close files when done saving"
    n16 = property class="DAQmx Read"(reference=w136) -> (reference out=w135:refnum<k21>, "AvailSampPerChan"=→"AvailSampPerChan 2":u32)  [unwired: 1 in, 1 out]
    n17 = local read "Averaging Number"() -> (w131:i32)
    n18 = local read "Averaging Number"() -> (w137:i32)
    "# Samples/channel" <- w137
    n19 = local read "Sampling Rate"() -> (w434:dbl)
    n20 = call-poly <vilib>:"DAQmx Read.vi"("task/channels in"=w135, "number of samples per channel"=w131, "timeout"=10.0) -> ("task out"=w322:refnum<k21>, "data"=w132:dbl[][], "error out"=w246:errorcluster)  [unwired: 10 in]
    n21 = Unbundle By Name(w246) -> ("status"=w371:bool)
    n22 = Divide(x=w434, y="Cal Averaging") -> (x/y=→"Cal Final Sampling Rate":dbl)
    n23 = Divide(x=w434, y=w137) -> (x/y=→"Final Sampling Rate" →"# Samples/channel/s":dbl)
    n24 = case shown="True" w371 {
      frame False {
      }
      frame True {
        n25 = call <vilib>:"Beep.vi"() -> ()  [unwired: 12 in]
        "Buffer Overflow" <- TRUE
      }
    }
    n26 = local read "Buffer size\n(Samples/channel)"() -> (w318:u32)
    n27 = property class="DAQmx Read"(reference=w322) -> (reference out=w321:refnum<k21>, "AvailSampPerChan"=w319:u32)  [unwired: 1 in, 1 out]
    "AvailSampPerChan" <- w319
    n28 = local read "Cal values"() -> (w363:T1)
    n29 = Index Array(array=w132, index (row)=4) -> (element=w235:dbl[])  [unwired: 1 in]
    n30 = Index Array(array=w132, index (row)=0) -> (element=w245:dbl[])  [unwired: 1 in]
    n31 = Index Array(array=w132, index (row)=2) -> (element=w240:dbl[])  [unwired: 1 in]
    n32 = Index Array(array=w132, index (row)=1) -> (element=w244:dbl[])  [unwired: 1 in]
    n33 = Index Array(array=w132, index (row)=3) -> (element=w238:dbl[])  [unwired: 1 in]
    n34 = Index Array(array=w132, index (row)=6) -> (element=w237:dbl[])  [unwired: 1 in]
    n35 = Index Array(array=w132, index (row)=7) -> (element=w236:dbl[])  [unwired: 1 in]
    n36 = Index Array(array=w132, index (row)=5) -> (element=w234:dbl[])  [unwired: 1 in]
    n37 = Divide(x=w319, y=w318) -> (x/y=→"Buffer status":dbl)
    n38 = Unbundle(w363) -> ("AX alpha"=w351:dbl, "BX alpha"=w347:dbl, "AX kappa"=w343:dbl, "BX kappa"=w339:dbl, "AX offset"=w357:dbl, "BX offset"=w355:dbl, "AY alpha"=w354:dbl, "BY alpha"=w349:dbl, "AY kappa"=w345:dbl, "BY kappa"=w341:dbl, "AY offset"=w361:dbl, "BY offset"=w359:dbl)
    n39 = Multiply(x=w244, y=w243) -> (x*y=w239:dbl[])
    n40 = Multiply(x=w245, y=w243) -> (x*y=w241:dbl[])
    n41 = local write "AX alpha"(w351) -> ()
    n42 = local write "BY offset"(w359) -> ()
    n43 = Build Array(w241, w240, w239, w238, w237, w236, w235, w234) -> (w164:dbl[][])
    n44 = local write "BX alpha"(w347) -> ()
    n45 = case shown="True" "Reset data stream" {
      selector: "Reset data stream" -> [_ w572]
      tunnel: w321 -> [w564 w570]
      tunnel: [w564 w568] -> w323
      tunnel: w246 -> [w563 w567]
      tunnel: [w563 w565] -> _
      frame False {
      }
      frame True {
        n46 = Not(x=w572) -> (.not. x?=w571:bool)
        n47 = call <vilib>:"DAQmx Stop Task.vi"("task/channels in"=w570, "error in"=w567) -> ("task out"=w569:refnum<k21>, "error out"=w566:errorcluster)  [unwired: 12 in]
        n48 = local write "Reset data stream"(w571) -> ()
        n49 = local write "Buffer Overflow"(w571) -> ()
        n50 = call <vilib>:"DAQmx Start Task.vi"("task/channels in"=w569, "error in"=w566) -> ("task out"=w568:refnum<k21>, "error out"=w565:errorcluster)  [unwired: 12 in]
      }
    }
    n51 = call-poly <vilib>:"Mean.vi"("X"=w234) -> ("mean"=w377:dbl)  [unwired: 1 out]
    n52 = local write "AY offset"(w361) -> ()
    n53 = call-poly <vilib>:"Mean.vi"("X"=w235) -> ("mean"=w378:dbl)  [unwired: 1 out]
    n54 = call-poly <vilib>:"Mean.vi"("X"=w240) -> ("mean"=w384:dbl)  [unwired: 1 out]
    n55 = call-poly <vilib>:"Mean.vi"("X"=w238) -> ("mean"=w382:dbl)  [unwired: 1 out]
    n56 = call-poly <vilib>:"Mean.vi"("X"=w237) -> ("mean"=w381:dbl)  [unwired: 1 out]
    n57 = call-poly <vilib>:"Mean.vi"("X"=w236) -> ("mean"=w380:dbl)  [unwired: 1 out]
    n58 = local read "Averaging Number"() -> (w130:i32)
    n59 = local write "BY kappa"(w341) -> ()
    n60 = local write "AX kappa"(w343) -> ()
    n61 = call-poly <vilib>:"Mean.vi"("X"=w239) -> ("mean"=w383:dbl)  [unwired: 1 out]
    n62 = local write "AY kappa"(w345) -> ()
    n63 = call-poly <vilib>:"Mean.vi"("X"=w241) -> ("mean"=w385:dbl)  [unwired: 1 out]
    n64 = local read "DAQ rate\n(Samples/s)"() -> (w142:dbl)
    n65 = Build Array(w378, w377) -> (w376:dbl[])
    n66 = local write "BX kappa"(w339) -> ()
    n67 = local write "BY alpha"(w349) -> ()
    n68 = local write "AX offset"(w357) -> ()
    n69 = local write "BX offset"(w355) -> ()
    n70 = local write "AY alpha"(w354) -> ()
    n71 = Build Array(w385, w384, w383, w382, w381, w380) -> (w374:dbl[])
    n72 = Divide(x=w130, y=w142) -> (x/y=w139:dbl)
    "Data update period (s/set)" <- w139
    n73 = Reciprocal(x=w142) -> (1/x=w143:dbl)
    "Data period (s)" <- w143
    n74 = Divide(x=w385, y=w381) -> (x/y=w415:dbl)
    n75 = Divide(x=w384, y=w381) -> (x/y=w416:dbl)
    n76 = Divide(x=w383, y=w380) -> (x/y=w423:dbl)
    n77 = Divide(x=w382, y=w380) -> (x/y=w424:dbl)
    n78 = Subtract(x=w415, y="AY offset") -> (x-y=w397:dbl)
    n79 = Subtract(x=w416, y="AX offset") -> (x-y=w398:dbl)
    n80 = Subtract(x=w423, y="BY offset") -> (x-y=w396:dbl)
    n81 = Subtract(x=w424, y="BX offset") -> (x-y=w399:dbl)
    n82 = Subtract(x=w423, y=w415) -> (x-y=w413:dbl)
    n83 = Subtract(x=w424, y=w416) -> (x-y=w414:dbl)
    n84 = feedback #1(0.0) -> (w317:dbl)
    n85 = Multiply(x="Downsamp\nfact", y=w143) -> (x*y=w144:dbl)
    n86 = Multiply(x=w397, y="AY alpha") -> (x*y=w331:dbl)
    n87 = Multiply(x=w398, y="AX alpha") -> (x*y=w329:dbl)
    n88 = Multiply(x=w399, y="BX alpha") -> (x*y=w330:dbl)
    n89 = Multiply(x=w396, y="BY alpha") -> (x*y=w332:dbl)
    n90 = Add(x=w139, y=w317) -> (x+y=w315:dbl)
    n91 = feedback-in #1(w315) -> ()
    n92 = Square(x=w331) -> (x^2=w407:dbl)
    n93 = Square(x=w329) -> (x^2=w408:dbl)
    n94 = Square(x=w332) -> (x^2=w409:dbl)
    n95 = Square(x=w330) -> (x^2=w410:dbl)
    n96 = Bundle(w413, w414) -> (w133:cluster{dbl, dbl})  [unwired: 1 in]
    n97 = case shown="True" "Set reading to\nsetpoint" {
      tunnel: w133 -> [_ w561]
      frame False {
      }
      frame True {
        n98 = local write "Set reading to\nsetpoint"(FALSE ("Set reading to\nsetpoint")) -> ()
        n99 = local read "Trap position"() -> (w560:cluster{"X":dbl, "Y":dbl})
        n100 = property on="Setpoint voltage" class="Clust (strict)"("Val(Sgnl)"=w561) -> ()  [unwired: 2 in, 2 out]
        n101 = Unbundle(w560) -> ("X"=w559:dbl, "Y"=w558:dbl)
        n102 = Bundle("Y"=w558, "X"=w559) -> (w557:cluster{"Y":dbl, "X":dbl})  [unwired: 1 in]
        n103 = property on="Offset" class="Clust (strict)"("Val(Sgnl)"=w557) -> ()  [unwired: 2 in, 2 out]
      }
    }
    n104 = Reciprocal(x=w144) -> (1/x=→"Chart Freq (Hz)":dbl)
    n105 = To Time Stamp(1:w315) -> (0:w314:timestamp)
    n106 = Add(x=w407, y=w408) -> (x+y=w411:dbl)
    n107 = Add(x=w409, y=w410) -> (x+y=w422:dbl)
    n108 = Multiply(x=w329, y="AX kappa") -> (x*y=w325:dbl)
    n109 = Bundle("A y", "A x", "B y", "B x", "A sum", "B sum", "Trap x", "Trap y") -> (w305:T11)  [unwired: 1 in]
    n110 = Multiply(x=w330, y="BX kappa") -> (x*y=w326:dbl)
    n111 = Square Root(x=w411) -> (sqrt(x)=w427:dbl)
    n112 = Square Root(x=w422) -> (sqrt(x)=w426:dbl)
    n113 = Multiply(x=w331, y="AY kappa") -> (x*y=w327:dbl)
    n114 = Multiply(x=w332, y="BY kappa") -> (x*y=w328:dbl)
    n115 = Subtract(x=w377, y="Fixed Y") -> (x-y=w412:dbl)
    n116 = Subtract(x=w378, y="Fixed X") -> (x-y=w417:dbl)
    n117 = Cluster To Array(cluster=w305) -> (array=w304:string[])
    n118 = for {
      tunnel: w164 -> [w549] mode=indexing
      tunnel: w144 -> [w548]
      tunnel: "Downsamp\nfact" -> [w554]
      tunnel: [w552] -> w220 mode=indexing
      tunnel: w314 -> [w556]
      tunnel: w304 -> [w551] mode=indexing
      tunnel: "NI_ChannelName" ("name") -> [w550]
      n119 = call "Downsample 1D array.vi"("Ave N"=w554, "Arrray In"=w549) -> ("Array Out"=w555:dbl[])  [unwired: 9 in]
      n120 = Bundle By Name("Y"=w555, "dt"=w548, "t0"=w556) -> (w553:waveform(dbl))  [unwired: 1 in]
      n121 = Set Waveform Attribute(5:w551, 6:w550, 7:w553) -> (3:w552:waveform(dbl))  [unwired: 1 in, 2 out]
    }
    "All signals" <- w220
    n122 = Square(x=w327) -> (x^2=w400:dbl)
    n123 = Square(x=w325) -> (x^2=w401:dbl)
    n124 = Square(x=w328) -> (x^2=w402:dbl)
    n125 = Square(x=w326) -> (x^2=w403:dbl)
    n126 = Add(x=w400, y=w401) -> (x+y=w404:dbl)
    n127 = Add(x=w402, y=w403) -> (x+y=w405:dbl)
    n128 = Multiply(x=w412, y="Conv Y (nm/V)") -> (x*y=w334:dbl)
    n129 = Multiply(x=w417, y="Conv X (nm/V)") -> (x*y=w335:dbl)
    n130 = feedback #2() -> (w372:cluster{"B_Y":dbl, "B_X":dbl})  [unwired: 1 in]
    n131 = case shown="True" "Force Feedback" {
      tunnel: [w840 w856] -> w124
      tunnel: [w839 w855] -> w122
      tunnel: w133 -> [_ w854]
      tunnel: [cluster{"B_Y":dbl, "B_X":dbl} {"B_Y"=0.0, "B_X"=0.0} ("Sum error past") w846] -> w373
      tunnel: w372 -> [_ w853]
      tunnel: w431 -> [w840 w849]
      tunnel: w436 -> [w839 w848]
      frame False {
        # "Force feedback"
      }
      frame True {
        n132 = call "ForceFeedback2.vi"("PSD/Mirror Voltages"=w854, "Sum error"=w853, "task/channels in"=w849, "error in"=w848, "Desired voltage"="Setpoint voltage", "Feedback const"="Feedback const", "offset"="Offset") -> ("task out"=w856:refnum<k21>, "Sum error past"=w846:cluster{"B_Y":dbl, "B_X":dbl}, "Output Voltage"=→"Feedback Output Voltage 2":cluster{dbl, dbl}, "error out"=w855:errorcluster)  [unwired: 8 in, 1 out]
        n133 = local read "Pulling direction"() -> (w845:bool)
        n134 = Unbundle(w846) -> ("B_Y"=w843:dbl, "B_X"=w842:dbl)
        n135 = Select(t=w843, s=w845, f=w842) -> (s? t:f=→"Sum error":dbl)
      }
    }
    n136 = feedback-in #2(w373) -> ()
    n137 = Square Root(x=w404) -> (sqrt(x)=w333:dbl)
    n138 = Square Root(x=w405) -> (sqrt(x)=w428:dbl)
    n139 = Add(x=w333, y=w428) -> (x+y=w406:dbl)
    n140 = Build Array(w415, w416, w423, w424, w381, w380, w333, w428, w427, w426, w335, w334) -> ()  [unwired: 1 out]
    n141 = Divide(x=w406, y=2.0) -> (x/y=w370:dbl)
    n142 = Index Array(array=w220, index=6) -> (element=w169:waveform(dbl))
    n143 = Index Array(array=w220, index=7) -> (element=w171:waveform(dbl))
    n144 = local read "Fixed X"() -> (w224:dbl)
    n145 = local read "Fixed Y"() -> (w226:dbl)
    n146 = Unbundle By Name(w169) -> ("Y"=w228:dbl[])
    n147 = Unbundle By Name(w171) -> ("Y"=w227:dbl[])
    n148 = Index Array(array=w220, index=0) -> (element=w177:waveform(dbl))
    n149 = Index Array(array=w220, index=1) -> (element=w301:waveform(dbl))
    n150 = Index Array(array=w220, index=4) -> (element=w295:waveform(dbl))
    n151 = Subtract(x=w228, y=w224) -> (x-y=w225:dbl[])
    n152 = Subtract(x=w227, y=w226) -> (x-y=w222:dbl[])
    n153 = Unbundle By Name(w177) -> ("Y"=w293:dbl[])
    n154 = Unbundle By Name(w301) -> ("Y"=w292:dbl[])
    n155 = Unbundle By Name(w295) -> ("Y"=w291:dbl[])
    n156 = Index Array(array=w220, index=5) -> (element=w294:waveform(dbl))
    n157 = local read "Conv X (nm/V)"() -> (w223:dbl)
    n158 = local read "Conv Y (nm/V)"() -> (w221:dbl)
    n159 = Index Array(array=w220, index=2) -> (element=w174:waveform(dbl))
    n160 = Index Array(array=w220, index=3) -> (element=w298:waveform(dbl))
    n161 = Set Waveform Attribute(5:"T2 X", 6:w167, 7:w169) -> (3:w168:waveform(dbl))  [unwired: 1 in, 2 out]
    n162 = Set Waveform Attribute(5:"T2 Y", 6:w167, 7:w171) -> (3:w170:waveform(dbl))  [unwired: 1 in, 2 out]
    n163 = Unbundle By Name(w294) -> ("Y"=w288:dbl[])
    n164 = Unbundle By Name(w174) -> ("Y"=w290:dbl[])
    n165 = Unbundle By Name(w298) -> ("Y"=w289:dbl[])
    n166 = local read "Saving"() -> (w336:bool)
    n167 = local read "Tether"() -> (w337:bool)
    n168 = Divide(x=w293, y=w291) -> (x/y=w192:dbl[])
    n169 = Divide(x=w292, y=w291) -> (x/y=w190:dbl[])
    n170 = local read "AY offset"() -> (w279:dbl)
    n171 = local read "AX offset"() -> (w277:dbl)
    n172 = Multiply(x=w225, y=w223) -> (x*y=w161:dbl[])
    n173 = Multiply(x=w222, y=w221) -> (x*y=w163:dbl[])
    n174 = Less?(x=w370, y="Tether break\nforce (pN)") -> (x < y?=w368:bool)
    n175 = Divide(x=w289, y=w288) -> (x/y=w191:dbl[])
    n176 = Subtract(x=w190, y=w277) -> (x-y=w280:dbl[])
    n177 = local read "BY offset"() -> (w284:dbl)
    n178 = local read "BX offset"() -> (w287:dbl)
    n179 = Subtract(x=w192, y=w279) -> (x-y=w281:dbl[])
    n180 = Divide(x=w290, y=w288) -> (x/y=w193:dbl[])
    n181 = local read "AY alpha"() -> (w278:dbl)
    n182 = local read "AX alpha"() -> (w276:dbl)
    n183 = Compound Arithmetic op=AND(w336, w337, w368) -> (w367:bool)
    n184 = call-poly <vilib>:"Mean.vi"("X"=w163) -> ("mean"=w203:dbl)  [unwired: 1 out]
    "Mean Trp Pos Y 2 (nm)" <- w203
    n185 = Subtract(x=w193, y=w192) -> (x-y=w189:dbl[])
    n186 = Subtract(x=w191, y=w190) -> (x-y=w188:dbl[])
    n187 = Subtract(x=w161, y="Offset X (nm)") -> (x-y=w160:dbl[])
    n188 = Subtract(x=w163, y="Offset Y (nm)") -> (x-y=w162:dbl[])
    n189 = Subtract(x=w193, y=w284) -> (x-y=w286:dbl[])
    n190 = Subtract(x=w191, y=w287) -> (x-y=w285:dbl[])
    n191 = Subtract(x=w203, y=w163) -> (x-y=w202:dbl[])
    n192 = call-poly <vilib>:"Mean.vi"("X"=w161) -> ("mean"=w207:dbl)  [unwired: 1 out]
    "Mean Trap Pos X 2 (nm)" <- w207
    n193 = Build Array(w189, w188) -> (w186:dbl[][])
    n194 = Index Array(array=w186, index (row)=0) -> (element=w184:dbl[])  [unwired: 1 in]
    n195 = Index Array(array=w186, index (row)=1) -> (element=w183:dbl[])  [unwired: 1 in]
    n196 = call-poly <vilib>:"Mean.vi"("X"=w184) -> ("mean"=w182:dbl)  [unwired: 1 out]
    n197 = call-poly <vilib>:"Mean.vi"("X"=w183) -> ("mean"=w181:dbl)  [unwired: 1 out]
    n198 = Bundle("mean"=w182, "mean"=w181) -> ()  [unwired: 1 in, 1 out]
    n199 = local read "BY alpha"() -> (w283:dbl)
    n200 = local read "BX alpha"() -> (w282:dbl)
    n201 = Multiply(x=w281, y=w278) -> (x*y=w269:dbl[])
    n202 = Multiply(x=w280, y=w276) -> (x*y=w268:dbl[])
    n203 = Square(x=w202) -> (x^2=w201:dbl[])
    n204 = Subtract(x=w207, y=w161) -> (x-y=w206:dbl[])
    n205 = Bundle By Name(cluster=w170, "Y"=w162) -> (w218:waveform(dbl))
    n206 = Bundle By Name(cluster=w168, "Y"=w160) -> (w219:waveform(dbl))
    n207 = case shown="True" w367 {
      selector: w367 -> [_ w575]
      frame False {
      }
      frame True {
        n208 = call <vilib>:"Beep.vi"() -> ()  [unwired: 12 in]
        n209 = Not(x=w575) -> (.not. x?=w573:bool)
        n210 = local write "Tether"(w573) -> ()
        n211 = local write "Force Feedback"(w573) -> ()
        n212 = property on="Stop saving" class="Bool (strict)"("Val(Sgnl)"="TA Cancel Save?") -> ()  [unwired: 2 in, 2 out]
      }
    }
    n213 = Square(x=w206) -> (x^2=w205:dbl[])
    n214 = call-poly <vilib>:"Mean.vi"("X"=w201) -> ("mean"=w200:dbl)  [unwired: 1 out]
    n215 = Square(x=w269) -> (x^2=w275:dbl[])
    n216 = Multiply(x=w286, y=w283) -> (x*y=w267:dbl[])
    n217 = Square(x=w268) -> (x^2=w274:dbl[])
    n218 = Multiply(x=w285, y=w282) -> (x*y=w266:dbl[])
    n219 = call-poly <vilib>:"Mean.vi"("X"=w205) -> ("mean"=w204:dbl)  [unwired: 1 out]
    n220 = Build Array(w219, w218) -> (w125:waveform(dbl)[])
    "Trap sep" <- w125
    n221 = Square Root(x=w200) -> (sqrt(x)=w199:dbl)
    n222 = Square(x=w267) -> (x^2=w273:dbl[])
    n223 = Square(x=w266) -> (x^2=w272:dbl[])
    n224 = Add(x=w275, y=w274) -> (x+y=w271:dbl[])
    n225 = Square Root(x=w204) -> (sqrt(x)=w197:dbl)
    n226 = Multiply(x=w199, y=10) -> (x*y=→"T2 Y RMS (A)":dbl)
    n227 = Square Root(x=w271) -> (sqrt(x)=w156:dbl[])
    n228 = Add(x=w273, y=w272) -> (x+y=w270:dbl[])
    n229 = Set Waveform Attribute(5:"T2", 6:"NI_ChannelName" ("name"), 7:w177) -> (3:w176:waveform(dbl))  [unwired: 1 in, 2 out]
    n230 = Set Waveform Attribute(5:"T1", 6:"NI_ChannelName" ("name"), 7:w174) -> (3:w173:waveform(dbl))  [unwired: 1 in, 2 out]
    n231 = Square Root(x=w270) -> (sqrt(x)=w155:dbl[])
    n232 = Multiply(x=w197, y=10) -> (x*y=→"T2 X RMS (A)":dbl)
    n233 = Bundle By Name(cluster=w176, "Y"=w156) -> (w180:waveform(dbl))
    n234 = Bundle By Name(cluster=w173, "Y"=w155) -> (w248:waveform(dbl))
    n235 = Add(x=w156, y=w155) -> (x+y=w154:dbl[])
    n236 = case shown="True" "Remove offsets" {
      selector: "Remove offsets" -> [_ w546]
      frame False {
      }
      frame True {
        n237 = local read "Mean Trp Pos Y 2 (nm)"() -> (w544:dbl)
        n238 = Not(x=w546) -> (.not. x?=w547:bool)
        n239 = local read "Mean Trap Pos X 2 (nm)"() -> (w545:dbl)
        n240 = local write "Remove offsets"(w547) -> ()
        n241 = local write "Offset Y (nm)"(w544) -> ()
        n242 = local write "Offset X (nm)"(w545) -> ()
      }
    }
    n243 = Build Array(w180, w248) -> (→"Bead sep":waveform(dbl)[])
    n244 = local read "AY kappa"() -> (w265:dbl)
    n245 = local read "AX kappa"() -> (w264:dbl)
    n246 = Divide(x=w154, y=2) -> (x/y=w152:dbl[])
    n247 = local read "Raster scanning..."() -> (w120:bool)
    n248 = local read "BX kappa"() -> (w262:dbl)
    n249 = local read "BY kappa"() -> (w263:dbl)
    n250 = call-poly <vilib>:"Mean.vi"("X"=w152) -> ("mean"=w151:dbl)  [unwired: 1 out]
    "Mean Bead Sep\n(nm)" <- w151
    n251 = local read "Calibrating"() -> (w429:bool)
    n252 = Multiply(x=w269, y=w265) -> (x*y=w258:dbl[])
    n253 = Multiply(x=w268, y=w264) -> (x*y=w259:dbl[])
    n254 = Square(x=w258) -> (x^2=w257:dbl[])
    n255 = Square(x=w259) -> (x^2=w256:dbl[])
    n256 = Subtract(x=w152, y=w151) -> (x-y=w150:dbl[])
    n257 = Multiply(x=w267, y=w263) -> (x*y=w260:dbl[])
    n258 = Multiply(x=w266, y=w262) -> (x*y=w261:dbl[])
    n259 = Add(x=w257, y=w256) -> (x+y=w253:dbl[])
    n260 = Square(x=w150) -> (x^2=w149:dbl[])
    n261 = Or(x=w120, y="Raster scan") -> (x .or. y?=w119:bool)
    n262 = Square Root(x=w253) -> (sqrt(x)=w217:dbl[])
    n263 = Square(x=w260) -> (x^2=w255:dbl[])
    n264 = Square(x=w261) -> (x^2=w254:dbl[])
    n265 = call-poly <vilib>:"Mean.vi"("X"=w149) -> ("mean"=w148:dbl)  [unwired: 1 out]
    n266 = Add(x=w255, y=w254) -> (x+y=w252:dbl[])
    n267 = Bundle By Name(cluster=w176, "Y"=w217) -> (w251:waveform(dbl))
    n268 = local read "Saving"() -> (w366:bool)
    n269 = Or(x=w429, y=w366) -> ()  [unwired: 1 out]
    n270 = Square Root(x=w148) -> (sqrt(x)=w147:dbl)
    n271 = Square Root(x=w252) -> (sqrt(x)=w216:dbl[])
    n272 = Multiply(x=10, y=w147) -> (x*y=→"Bead Sep Noise\n(A)":dbl)
    n273 = Bundle By Name(cluster=w173, "Y"=w216) -> (w250:waveform(dbl))
    n274 = Add(x=w217, y=w216) -> (x+y=w215:dbl[])
    n275 = Build Array(w251, w250) -> (→"Force (pN)":waveform(dbl)[])
    n276 = Divide(x=w215, y=2) -> (x/y=w212:dbl[])
    n277 = call-poly <vilib>:"Mean.vi"("X"=w212) -> ("mean"=w213:dbl)  [unwired: 1 out]
    "Mean force (pN)" <- w213
    n278 = Subtract(x=w213, y=w212) -> (x-y=w211:dbl[])
    n279 = Square(x=w211) -> (x^2=w210:dbl[])
    n280 = call-poly <vilib>:"Mean.vi"("X"=w210) -> ("mean"=w209:dbl)  [unwired: 1 out]
    n281 = Square Root(x=w209) -> (sqrt(x)=→"Force noise (pN)":dbl)
    n282 = flat-sequence {
      tunnel: w429 -> [w615]
      tunnel: w366 -> [_]
      tunnel: w429 -> [_]
      tunnel: w366 -> [_]
      tunnel: w164 -> [w602]
      tunnel: [w602] -> w387
      tunnel: w246 -> [w601]
      tunnel: [w601] -> w386
      tunnel: w374 -> [w600]
      tunnel: [w600] -> w379
      tunnel: w376 -> [w599]
      tunnel: [w599] -> w375
      tunnel: [w596] -> w365
      tunnel: [w593] -> w364
      tunnel: [w590] -> w233
      tunnel: [w589] -> w232
      tunnel: [w586] -> w231
      tunnel: w127 -> [w583]
      tunnel: ["Save Data"] -> w126
      tunnel: w387 -> [w762]
      tunnel: w386 -> [w761]
      tunnel: w379 -> [_]
      tunnel: w375 -> [_]
      tunnel: w365 -> [w760]
      tunnel: w364 -> [w759]
      tunnel: w233 -> [w758]
      tunnel: w232 -> [w757]
      tunnel: w231 -> [w756]
      tunnel: w126 -> [w754]
      tunnel: w125 -> [w753]
      frame #0 {
        w581 = 0.0
        # "1: old trap\n0: fleezers"
        # "Create files if saving data"
        n283 = local read "Save N sets"() -> (w585:bool)
        n284 = local read "Sampling Rate"() -> (w613:dbl)
        n285 = Or(x=w585, y="Save Data") -> (x .or. y?=w584:bool)
        n286 = Build Array(w584, "Save cal", w583) -> (w604:bool[])
        n287 = Compound Arithmetic op=OR("Save Data", "Save cal", w583) -> (w606:bool)
        n288 = Boolean Array To Number(Boolean array=w604) -> (number=w603:u32)
        n289 = local read "Trap position"() -> (w610:cluster{"X":dbl, "Y":dbl})
        n290 = local read "Fixed X"() -> (w580:dbl)
        n291 = local read "Fixed Y"() -> (w579:dbl)
        n292 = Unbundle(w610) -> ("X"=w578:dbl, "Y"=w577:dbl)
        n293 = Build Array(w578, w577, w580, w579, w581, w581) -> (w609:dbl[])
        n294 = feedback #3(refnum<k0> refnum) -> (w594:refnum<file>)
        n295 = feedback #4() -> (w591:dbl)  [unwired: 1 in]
        n296 = feedback #5(FALSE) -> (w587:bool)
        n297 = feedback #6(0) -> (w607:i32)
        n298 = feedback #7(refnum<k0> refnum) -> (w597:refnum<file>)
        n299 = case shown="True" w606 {
          tunnel: w615 -> [_ _]
          tunnel: 9 -> [_ w657]
          tunnel: w613 -> [_ w656]
          tunnel: 6 -> [_ w655]
          tunnel: 5 -> [_ w654]
          tunnel: w609 -> [_ w653]
          tunnel: [w620 1] -> w590
          tunnel: w607 -> [w621 _]
          tunnel: w603 -> [_ w628]
          tunnel: [w619 w626] -> w596
          tunnel: w597 -> [w619 _]
          tunnel: [w618 w625] -> w593
          tunnel: w594 -> [w618 _]
          tunnel: 1.0 -> [_ w624]
          tunnel: [w617 w623] -> w589
          tunnel: w591 -> [w617 _]
          tunnel: [w616 w622] -> w586
          tunnel: w587 -> [w616 _]
          frame False {
            n300 = Increment(x=w621) -> (x+1=w620:i32)
          }
          frame True {
            w629 = FALSE ("Save Data")
            w635 = FALSE
            w636 = T10."big-endian, network order" ("byte order (0:big-endian, network order)")
            n301 = local write "Save cal"(w629) -> ()
            n302 = local write "Save Data"(w629) -> ()
            n303 = case shown="4" w628 {
              tunnel: w657 -> [w704 w722 w752]
              tunnel: w656 -> [w682 w721 w727]
              tunnel: w655 -> [w703 w719 w748]
              tunnel: w654 -> [w702 w718 w747]
              tunnel: w653 -> [w700 w715 w744]
              tunnel: [w699 w714 w733] -> w650
              tunnel: [w701 w711 w732] -> w622
              tunnel: ["Averaging Number" 200 w730] -> _
              tunnel: w624 -> [w687 w706 w729]
              tunnel: [w683 "Cal sets to save" w723] -> w623
              frame 1, Default {
                w701 = TRUE
                w688 = 0.0
                # "Time trace"
                n304 = local read "Averaging Number"() -> (w698:i32)
                n305 = Boolean To (0,1)(Boolean=w701) -> (0, 1=w693:i16)
                n306 = Increment(x=w693) -> (x+1=w692:i16)
                n307 = Divide(x=w682, y=w698) -> (x/y=w697:dbl)
                n308 = To Double Precision Float(number=w692) -> (double precision float=w691:dbl)
                n309 = Reciprocal(x=w697) -> (1/x=w696:dbl)
                n310 = Reciprocal(x=w682) -> (1/x=w681:dbl)
                n311 = Build Array(w704, w681, w696, w703, w702, 0 ("f")) -> (w695:dbl[])
                n312 = Build Array(w691, w687, w688, w688, w688) -> (w694:dbl[])
                n313 = Build Array (concatenate)(w695, w700, w694) -> (w699:dbl[])
                n314 = Select(t="N sets", s="Save N sets", f=2147483647) -> (s? t:f=w683:i32)
              }
              frame 2 {
                w711 = FALSE
                w709 = 0.0
                # "Calibration file"
                n315 = Reciprocal(x=w721) -> (1/x=w720:dbl)
                n316 = Boolean To (0,1)(Boolean=w711) -> (0, 1=w713:i16)
                n317 = To Double Precision Float(number=w713) -> (double precision float=w712:dbl)
                n318 = Build Array(w722, w720, w720, w719, w718, 1) -> (w716:dbl[])
                n319 = Build Array(w712, w706, w709, w709, w709) -> (w710:dbl[])
                n320 = Build Array (concatenate)(w716, w715, w710) -> (w714:dbl[])
                "Calibrating" <- TRUE ("Calibrating")
              }
              frame 4 {
                w740 = 0.0
                w732 = TRUE
                # "Not using ncycles"
                # "FX curve"
                n321 = local read "Averaging Number"() -> (w751:i32)
                n322 = Boolean To (0,1)(Boolean=w732) -> (0, 1=w743:i16)
                n323 = Increment(x=w743) -> (x+1=w742:i16)
                n324 = local write "Raster scan"(FALSE ("Raster scan")) -> ()
                n325 = To Double Precision Float(number=w742) -> (double precision float=w741:dbl)
                n326 = Divide(x=w727, y=w751) -> (x/y=w750:dbl)
                n327 = Reciprocal(x=w750) -> (1/x=w749:dbl)
                n328 = Build Array(w741, w729, w740, w740, w740) -> (w739:dbl[])
                n329 = Reciprocal(x=w727) -> (1/x=w726:dbl)
                n330 = Build Array(w752, w726, w749, w748, w747, 2) -> (w745:dbl[])
                n331 = local read "Pulling direction"() -> (w737:bool)
                n332 = local read "Scan range (V)"() -> (w724:dbl)
                n333 = local read "N sets to be saved"() -> (w723:dbl)
                n334 = local read "Scan steps (mirror)"() -> (w725:u64)
                n335 = local read "# scans"() -> (w735:i32)
                n336 = Not(x=w737) -> (.not. x?=w736:bool)
                n337 = local read "Averaging Number"() -> (w730:i32)
                n338 = Boolean To (0,1)(Boolean=w736) -> (0, 1=w738:i16)
                n339 = Build Array(w738, w724, w725, 0, w735) -> (w734:dbl[])
                n340 = Build Array (concatenate)(w745, w744, w739, w734) -> (w733:dbl[])
              }
            }
            n341 = call "CreateSaveFile.vi"("Index In"="Save file index", "Ext"=".dat", "Insert"="", "Directory"="Path") -> ("Path Out"=w634:path)  [unwired: 6 in, 1 out]
            "Current file name" <- w634
            n342 = Open/Create/Replace File(file path (use dialog)=w634, operation (0:open)=T9."create", access (0:read/write)=enum16{"read/write", "read-only", "write-only"}."write-only") -> (refnum out=w643:refnum<file>, error out=w644:errorcluster)  [unwired: 3 in, 1 out]
            n343 = Array Size(array=w650) -> (size(s)=w652:i32)
            n344 = case shown="True" w622 {
              tunnel: w634 -> [_ w680]
              tunnel: [refnum<k0> refnum w659] -> w625
              frame False {
              }
              frame True {
                w666 = 0.0
                n345 = Path To String(path=w680) -> (string=w676:string)
                n346 = Build Array(w666, w666, w666, w666, w666, w666, w666, w666) -> (w663:dbl[])
                n347 = String Length(string=w676) -> (length=w679:i32)
                n348 = Array Size(array=w663) -> (size(s)=w665:i32)
                n349 = Subtract(x=w679, y=4) -> (x-y=w677:i32)
                n350 = To Double Precision Float(number=w665) -> (double precision float=w664:dbl)
                n351 = String Subset(string=w676, length (rest)=w677) -> (substring=w675:string)  [unwired: 1 in]
                n352 = Build Array (concatenate)(w664, w663) -> (w662:dbl[])
                n353 = Concatenate Strings(w675, "_pos.dat" ("string")) -> (w673:string)
                n354 = String To Path(string=w673) -> (path=w672:path)
                n355 = Open/Create/Replace File(file path (use dialog)=w672, operation (0:open)=T9."create", access (0:read/write)=enum16{"read/write", "read-only", "write-only"}."write-only") -> (refnum out=w668:refnum<file>, error out=w669:errorcluster)  [unwired: 3 in, 1 out]
                n356 = Deny Access(4:w669, 7:w668) -> (3:w667:refnum<file>)  [unwired: 1 in, 1 out]
                n357 = Write to Binary File(file (use dialog)=w667, data=w662, 5:FALSE ("prepend array or string size? (T)"), 9:T10."big-endian, network order" ("byte order (0:big-endian, network order)")) -> (refnum out=w659:refnum<file>)  [unwired: 2 in, 2 out]
              }
            }
            n358 = Deny Access(4:w644, 7:w643) -> (0:w633:errorcluster, 3:w642:refnum<file>)  [unwired: 1 in]
            n359 = String Length(string="Comment") -> (length=w649:i32)
            n360 = To Double Precision Float(number=w652) -> (double precision float=w651:dbl)
            n361 = To Double Precision Float(number=w649) -> (double precision float=w648:dbl)
            n362 = Build Array (concatenate)(w651, w650, w648) -> (w639:dbl[])
            n363 = Write to Binary File(file (use dialog)=w642, data=w639, error in=w633, 5:w635, 9:w636) -> (refnum out=w638:refnum<file>, error out=w632:errorcluster)  [unwired: 1 in, 1 out]
            n364 = Write to Binary File(file (use dialog)=w638, data="Comment", error in=w632, 5:w635, 9:w636) -> (refnum out=w626:refnum<file>)  [unwired: 1 in, 2 out]
            "Saving" <- TRUE
          }
        }
        n365 = feedback-in #3(w593) -> ()
        n366 = feedback-in #4(w589) -> ()
        n367 = feedback-in #5(w586) -> ()
        n368 = feedback-in #6(w590) -> ()
        n369 = feedback-in #7(w596) -> ()
      }
      frame #1 {
        n370 = local read "Saving"() -> (w755:bool)
        n371 = case shown="True" w755 {
          tunnel: w762 -> [_ w781]
          tunnel: w761 -> [_ w780]
          tunnel: w760 -> [_ w779]
          tunnel: w759 -> [_ w778]
          tunnel: w758 -> [_ w768]
          tunnel: w757 -> [_ w769]
          tunnel: w756 -> [_ w772]
          tunnel: w754 -> [_ w764]
          tunnel: w753 -> [_ w763]
          frame False {
            (unwired) FALSE ("Calibrating")
          }
          frame True {
            n372 = local read "Stop"() -> (w776:bool)
            n373 = Less Or Equal?(x=w768, y=w769) -> (x <= y?=w777:bool)
            n374 = Divide(x=w768, y=w769) -> (x/y=w767:dbl)
            n375 = Or(x=w776, y="Stop saving") -> (x .or. y?=w775:bool)
            n376 = Not(x=w775) -> (.not. x?=w774:bool)
            n377 = Multiply(x=100.0, y=w767) -> (x*y=w766:dbl)
            n378 = And(x=w777, y=w774) -> (x .and. y?=w773:bool)
            n379 = case shown="True" w773 {
              tunnel: w779 -> [w786 w795]
              tunnel: w780 -> [_ w794]
              tunnel: w781 -> [_ w793]
              tunnel: w778 -> [w785 w792]
              tunnel: w772 -> [w783 _]
              tunnel: [0.0 ("Progress") w791] -> w771
              tunnel: w766 -> [_ w791]
              tunnel: w764 -> [_ w788]
              tunnel: w763 -> [_ w789]
              frame False {
                w784 = FALSE
                n380 = Close File(refnum=w786) -> ()  [unwired: 1 in, 2 out]
                n381 = case shown="True" w783 {
                  tunnel: w785 -> [_ w787]
                  frame False {
                  }
                  frame True {
                    n382 = Close File(refnum=w787) -> ()  [unwired: 1 in, 2 out]
                  }
                }
                n383 = call <vilib>:"Beep.vi"() -> ()  [unwired: 12 in]
                n384 = local write "Saving"(w784) -> ()
                n385 = local write "Stop saving"(w784) -> ()
                n386 = local write "Calibrating"(w784) -> ()
              }
              frame True {
                n387 = local read "Calibrating"() -> (w790:bool)
                n388 = case shown="False" w790 {
                  tunnel: w795 -> [w822 w838]
                  tunnel: w794 -> [_ w837]
                  tunnel: w793 -> [w809 w831]
                  tunnel: w792 -> [w808 _]
                  tunnel: w789 -> [w800 _]
                  tunnel: w788 -> [_ _]
                  frame False {
                    n389 = local read "Averaging Number"() -> (w816:i32)
                    n390 = Array Subset(array=w809, index (row)=0 ("index"), length (row)=6 ("length")) -> (w805:dbl[][])  [unwired: 2 in]
                    n391 = Array Subset(array=w809, index (row)=6 ("index"), length (row)=2 ("length")) -> (w804:dbl[][])  [unwired: 2 in]
                    n392 = Array Size(array=w804) -> (size(s)=w815:i32[])
                    n393 = Array Size(array=w805) -> (size(s)=w812:i32[])
                    n394 = Index Array(array=w800, index=0) -> (element=w797:waveform(dbl))
                    n395 = Index Array(array=w800, index=1) -> (element=w796:waveform(dbl))
                    n396 = for {
                      tunnel: w805 -> [w826] mode=indexing
                      tunnel: w816 -> [w828]
                      tunnel: [w827] -> w803 mode=indexing
                      n397 = call "Downsample 1D array.vi"("Ave N"=w828, "Arrray In"=w826) -> ("Array Out"=w827:dbl[])  [unwired: 9 in]
                    }
                    n398 = Unbundle By Name(w797) -> ()  [unwired: 1 out]
                    n399 = Unbundle By Name(w796) -> ()  [unwired: 1 out]
                    n400 = Multiply Array Elements(1:w812) -> (0:w811:i32)
                    n401 = for {
                      tunnel: w804 -> [w825] mode=indexing
                      tunnel: w816 -> [w824]
                      tunnel: [w823] -> w807 mode=indexing
                      n402 = call "Downsample 1D array.vi"("Ave N"=w824, "Arrray In"=w825) -> ("Array Out"=w823:dbl[])  [unwired: 9 in]
                    }
                    n403 = Multiply Array Elements(1:w815) -> (0:w814:i32)
                    n404 = Divide(x=w811, y=w816) -> (x/y=w817:dbl)
                    n405 = Divide(x=w814, y=w816) -> (x/y=w813:dbl)
                    n406 = Transpose 2D Array(2D array=w803) -> (transposed array=w802:dbl[][])
                    n407 = Transpose 2D Array(2D array=w807) -> (transposed array=w801:dbl[][])
                    n408 = Reshape Array(w802, w817) -> (w806:dbl[])
                    n409 = Reshape Array(w801, w813) -> (w810:dbl[])
                    n410 = call <vilib>:"Write File+ [SGL].vi"("1D array"=w810, "refnum"=w808) -> ()  [unwired: 7 in, 3 out]
                    n411 = call <vilib>:"Write File+ [SGL].vi"("1D array"=w806, "refnum"=w822) -> ()  [unwired: 7 in, 3 out]
                  }
                  frame True {
                    n412 = Array Subset(array=w831, index (row)=0 ("index"), length (row)=6 ("length")) -> (w829:dbl[][])  [unwired: 2 in]
                    n413 = Transpose 2D Array(2D array=w829) -> (transposed array=w835:dbl[][])
                    n414 = Array Size(array=w829) -> (size(s)=w830:i32[])
                    n415 = Multiply Array Elements(1:w830) -> (0:w836:i32)
                    n416 = Reshape Array(w835, w836) -> (w834:dbl[])
                    n417 = call <vilib>:"Write File+ [SGL].vi"("1D array"=w834, "error in (no error)"=w837, "refnum"=w838) -> ()  [unwired: 6 in, 3 out]
                  }
                }
              }
            }
            "Progress" <- w771
          }
        }
      }
    }
    n418 = local read "Flushing Sample"() -> (w129:bool)
    n419 = case shown="True" w129 {
      frame False {
      }
      frame True {
        n420 = local read "Flush Sample Start Time"() -> (w540:u32)
        n421 = local read "Sample flush time (s)"() -> (w533:dbl)
        n422 = Tick Count (ms)() -> (millisecond timer value=w541:u32)
        n423 = Subtract(x=w541, y=w540) -> (x-y=w531:u32)
        n424 = Multiply(x=u32 1000, y=w533) -> (x*y=w532:dbl)
        n425 = Divide(x=w531, y=w532) -> (x/y=w536:dbl)
        n426 = Greater?(x=w531, y=w532) -> (0:w539:bool)
        n427 = Not(x=w539) -> (.not. x?=w538:bool)
        n428 = Boolean To (0,1)(Boolean=w538) -> (0, 1=w537:i16)
        n429 = Compound Arithmetic op=MULTIPLY(w537, w536, 100.0 ("value")) -> (→"Sample Flush Meter":dbl)
        n430 = case shown="True" w539 {
          frame False {
          }
          frame True {
            w543 = FALSE ("Inject Sample")
            n431 = property on="Clear Volume" class="Bool (strict)"("Val(Sgnl)"=TRUE ("Value (Signaling)")) -> ()  [unwired: 2 in, 2 out]
            n432 = local write "Inject Sample"(w543) -> ()
            n433 = local write "Flushing Sample"(w543) -> ()
          }
        }
      }
    }
    n434 = feedback #8(0) -> (w112:i32)
    n435 = feedback #9(0) -> (w109:i32)
    n436 = feedback #10(0) -> (w114:i32)
    n437 = case shown="True" w119 {
      tunnel: w124 -> [w443 w491]
      tunnel: [w443 w475] -> w123
      tunnel: w122 -> [w442 w490]
      tunnel: [w442 w474] -> w121
      tunnel: "Raster scan" -> [w441 w464]
      tunnel: [w441 w463] -> w117
      tunnel: [0 w462] -> w115
      tunnel: w114 -> [_ w455]
      tunnel: w112 -> [_ w461]
      tunnel: [0 w446] -> w111
      tunnel: w109 -> [_ w452]
      tunnel: [0 w451] -> w108
      frame False {
      }
      frame True {
        # "Reset step counter"
        # "Current position"
        # "Initial values"
        n438 = local read "Trap position"() -> (w468:cluster{"X":dbl, "Y":dbl})
        n439 = local read "Data update period (s/set)"() -> (w460:dbl)
        n440 = local read "Time per step (ms)"() -> (w457:dbl)
        n441 = local read "Fixed X"() -> (w484:dbl)
        n442 = local read "Fixed Y"() -> (w485:dbl)
        n443 = Unbundle(w468) -> ("X"=w466:dbl, "Y"=w465:dbl)
        n444 = local read "Scan steps (mirror)"() -> (w473:u64)
        n445 = Multiply(x=w460, y=1000.0) -> (x*y=w458:dbl)
        n446 = local read "Stop raster"() -> (w480:bool)
        n447 = local read "Stop saving"() -> (w481:bool)
        n448 = Select(t=w484, s="Pulling direction", f=w485) -> (s? t:f=w492:dbl)
        n449 = Select(t=w465, s="Pulling direction", f=w466) -> (s? t:f=w467:dbl)
        n450 = Divide(x=w457, y=w458) -> (x/y=w456:dbl)
        n451 = Quotient & Remainder(x=w455, y=w456) -> (x-y*floor(x/y)=w454:dbl)  [unwired: 1 out]
        n452 = Not(x=w480) -> (.not. x?=w479:bool)
        n453 = Not(x=w481) -> (.not. x?=w478:bool)
        n454 = Multiply(x=u64 2, y=w473) -> (x*y=w469:u64)
        n455 = Equal To 0?(x=w454) -> (x = 0?=w453:bool)
        n456 = Less?(x=w461, y=w469) -> (x < y?=w470:bool)
        n457 = Compound Arithmetic op=AND(w470, w479, w478, w453) -> (w471:bool)
        n458 = Not(x=w470) -> (.not. x?=w449:bool)
        n459 = feedback #11() -> (w476:dbl)  [unwired: 1 in]
        n460 = case shown="True" w471 {
          tunnel: w492 -> [_ w526]
          tunnel: w467 -> [_ w508]
          tunnel: w491 -> [w503 w525]
          tunnel: w490 -> [w502 w524]
          tunnel: [w503 w523] -> w475
          tunnel: [w502 w522] -> w474
          tunnel: [w499 w511] -> w477
          tunnel: w461 -> [w500 w506]
          tunnel: w476 -> [w499 w505]
          tunnel: w464 -> [w501 w510]
          tunnel: [w501 w510] -> w463
          tunnel: [w500 w509] -> w447
          frame False {
          }
          frame True {
            # "Go forward or backward?"
            n461 = local read "Scan increment (V)"() -> (w504:dbl)
            n462 = local read "Scan steps (mirror)"() -> (w515:u64)
            n463 = Multiply(x=w504, y=w506) -> (x*y=w507:dbl)
            n464 = Less?(x=w506, y=w515) -> (x < y?=w514:bool)
            n465 = Add(x=w508, y=w507) -> (x+y=w517:dbl)
            n466 = Subtract(x=w505, y=w504) -> (x-y=w516:dbl)
            n467 = Select(t=w517, s=w514, f=w516) -> (s? t:f=w511:dbl)
            n468 = local read "Pulling direction"() -> (w513:bool)
            n469 = Build Array(w511, w526) -> (w520:dbl[])
            n470 = Build Array(w526, w511) -> (w519:dbl[])
            n471 = Select(t=w520, s=w513, f=w519) -> (s? t:f=w518:dbl[])
            n472 = call-poly <vilib>:"DAQmx Write.vi"("task/channels in"=w525, "auto start"=TRUE, "data"=w518, "error in"=w524) -> ("task out"=w523:refnum<k21>, "error out"=w522:errorcluster)  [unwired: 9 in, 1 out]
            n473 = Increment(x=w506) -> (x+1=w509:i32)
            "Raster scanning..." <- TRUE ("Raster scanning...")
          }
        }
        n474 = feedback-in #11(w477) -> ()
        n475 = case shown="True" w449 {
          tunnel: w452 -> [w496 w498]
          tunnel: [w496 w497] -> w451
          frame False {
          }
          frame True {
            n476 = Increment(x=w498) -> (x+1=w497:i32)
          }
        }
        n477 = local read "# scans"() -> (w450:i32)
        n478 = local read "Stop saving"() -> (w483:bool)
        n479 = Greater Or Equal?(x=w451, y=w450) -> (x >= y?=w444:bool)
        n480 = Not(x=w444) -> (.not. x?=w445:bool)
        n481 = And(x=w449, y=w445) -> (x .and. y?=w448:bool)
        n482 = Compound Arithmetic op=OR(w444, "Stop raster", w483) -> (w486:bool)
        n483 = case shown="True" w486 {
          frame False {
          }
          frame True {
            n484 = flat-sequence {
              frame #0 {
                n485 = Wait (ms)(milliseconds to wait=u32 300) -> ()  [unwired: 1 out]
              }
              frame #1 {
                n486 = property on="Trap delta" class="DigNum (strict)"("Val(Sgnl)"="Trap delta\nafter") -> ()  [unwired: 2 in, 2 out]
              }
            }
          }
        }
        n487 = And(x="Flow on\nafter raster?", y=w486) -> (x .and. y?=w487:bool)
        n488 = case shown="True" w487 {
          frame False {
          }
          frame True {
            n489 = property on="Inject Sample" class="Bool (strict)"("Val(Sgnl)"=TRUE ("Value (Signaling)")) -> ()  [unwired: 2 in, 2 out]
          }
        }
        n490 = case shown="False" w448 {
          tunnel: w447 -> [w494 _]
          tunnel: [w494 0] -> w446
          frame False {
          }
          frame True {
          }
        }
        n491 = Not(x=w486) -> (.not. x?=w489:bool)
        n492 = local write "Raster scanning..."(w489) -> ()
        n493 = Increment(x=w455) -> (x+1=w462:i32)
      }
    }
    n494 = And(x="Save scans", y=w117) -> (x .and. y?=w127:bool)
    n495 = feedback-in #8(w111) -> ()
    n496 = feedback-in #9(w108) -> ()
    n497 = feedback-in #10(w115) -> ()
    n498 = local read "Stop"() -> (w435:bool)
  }
  n499 = local write "Progress"(u8 0 ("Progress")) -> ()
  n500 = local write "Calibrating"(FALSE ("Calibrating")) -> ()
  n501 = call "InitializeChamberImage.vi"() -> ("error out"=w101:errorcluster, "IMAQ Session Out"=w102:refnum<k11>, "Display Out"=w103:T7, "Acquired Image"=w9:T7)  [unwired: 8 in]
  n502 = node-c288(i64 10 ("Period"), 2 ("Processor")) -> (w15:T12)  [unwired: 2 in]
  n503 = timed-loop {
    tunnel: w103 -> [w866]
    tunnel: w102 -> [w865]
    tunnel: w101 -> [w864]
    tunnel: [w862] -> w100
    tunnel: [w861] -> w99
    timing: w15 -> [_]
    timing-out: [_] -> w14
    i -> [w863]
    stop <- w857 continue-if-true
    n504 = node-c288() -> ()  [unwired: 1 in, 1 out]
    n505 = call <vilib>:"IMAQ Copy Acquired Buffer.vi"("IMAQ Session In"=w865, "Image In"=w866, "Buffer Number"=w863, "error in (no error)"=w864) -> ("IMAQ Session Out"=w862:refnum<k11>, "Image Out"=→"Chamber":T7, "error out"=w861:errorcluster)  [unwired: 7 in, 2 out]
    "Video Error" <- w861
    n506 = local read "Stop"() -> (w859:bool)
    n507 = Unbundle By Name(w861) -> ("status"=w860:bool)
    n508 = Not Or(1:w859, 2:w860) -> (0:w857:bool)
    "Continue to display?" <- w857
    n509 = node-c288() -> ()  [unwired: 1 in, 1 out]
  }
  n510 = node-c288(w14) -> ()  [unwired: 1 out]
  n511 = call <vilib>:"IMAQ Close.vi"("error in (no error)"=w99, "IMAQ Session In"=w100) -> ("error out"=w107:errorcluster)  [unwired: 9 in]
  n512 = call "IMAQ Dispose"("error in (no error)"=w107) -> ("error out"=w106:errorcluster)  [unwired: 5 in]
  n513 = call-poly "VISA Configure Serial Port"("VISA resource name"=refnum<visa-resource-name> "COM3") -> ("VISA resource name out"=w21:refnum<visa-resource-name>, "error out"=w20:errorcluster)  [unwired: 13 in]
  n514 = call "IMAQ Dispose"("Image"=w9, "error in (no error)"=w106) -> ("error out"=w105:errorcluster)  [unwired: 4 in]
  n515 = node-c288(i64 100 ("Period"), 2 ("Processor")) -> (w23:T12)  [unwired: 2 in]
  n516 = call <vilib>:"Simple Error Handler.vi"("error in (no error)"=w105) -> ()  [unwired: 4 in, 5 out]
  n517 = timed-loop {
    timing: w23 -> [_]
    timing-out: [_] -> w22
    tunnel: w21 -> [w869]
    tunnel: w20 -> [w871]
    tunnel: [w869] -> w19
    stop <- w870 stop-if-true
    n518 = node-c288() -> ()  [unwired: 1 in, 1 out]
    n519 = event shown="[0] \"Got DNA bead\": Value Change" {
      selector: _ -> [_ _ _ _ _ _ _ _ _ _ _]
      dyn-events: _ -> [_ _ _ _ _ _ _ _ _ _ _]
      timeout: _ -> [_ _ _ _ _ _ _ _ _ _ _]
      tunnel: w869 -> [w878 w917 w937 w954 w971 w990 w1010 _ _ _ _]
      tunnel: w871 -> [w877 w916 w936 w953 w970 w989 w1009 _ _ _ _]
      tunnel: [_ _ _ _ _ _ _ _ _ _ w1063] -> w870
      event "Got DNA bead": Value Change {
        n520 = event-data() -> ()  [unwired: 1 in, 5 out]
        n521 = flat-sequence {
          tunnel: w878 -> [w882]
          tunnel: w877 -> [w880]
          tunnel: [w897] -> w876
          tunnel: w876 -> [w900]
          tunnel: [w900] -> w875
          tunnel: w875 -> [w902]
          tunnel: [w902] -> w874
          tunnel: w874 -> [w906]
          tunnel: [w906] -> w873
          tunnel: w873 -> [w908]
          tunnel: [w908] -> w872
          tunnel: w872 -> [w910]
          frame #0 {
            n522 = local read "Saved stage positions"() -> (w883:dbl[][])
            n523 = disable-structure shown="Disabled" {
              frame Disabled {
                n524 = property on="Inject Pump 2" class="Bool (strict)"("Val(Sgnl)"=FALSE ("Inject Pump 2")) -> ()  [unwired: 2 in, 2 out]
              }
              frame Enabled {
              }
            }
            n525 = property on="Inject Sample" class="Bool (strict)"("Val(Sgnl)"=TRUE ("Value (Signaling)")) -> ()  [unwired: 2 in, 2 out]
            n526 = local write "Stage moving"(TRUE ("Stage moving")) -> ()
            n527 = property on="Trap delta" class="DigNum (strict)"("Val(Sgnl)"="Cal @ Delta (V)") -> ()  [unwired: 2 in, 2 out]
            n528 = call "move to saved stage position.vi"("error in"=w880, "Stage VISA resource name in"=w882, "Position"="Cal stage position", "Saved Stage Positions"=w883) -> ()  [unwired: 2 out]
          }
          frame #1 {
            n529 = local write "Stage moving"(FALSE ("Stage moving")) -> ()
            n530 = property on="Inject Sample" class="Bool (strict)"("Val(Sgnl)"=FALSE ("Value (Signaling)")) -> ()  [unwired: 2 in, 2 out]
            n531 = call <vilib>:"Beep.vi"() -> ()  [unwired: 12 in]
          }
          frame #2 {
            n532 = Wait (ms)(milliseconds to wait=u32 1000) -> ()  [unwired: 1 out]
          }
          frame #3 {
            n533 = property on="Save cal" class="Bool (strict)"("Val(Sgnl)"=TRUE ("Value (Signaling)")) -> ()  [unwired: 2 in, 2 out]
          }
          frame #4 {
            n534 = Wait (ms)(milliseconds to wait=u32 2000) -> ()  [unwired: 1 out]
          }
          frame #5 {
            n535 = while {
              stop <- w893 stop-if-true
              n536 = local read "Saving"() -> (w894:bool)
              n537 = Not(x=w894) -> (.not. x?=w893:bool)
              n538 = Wait (ms)(milliseconds to wait=u32 100) -> ()  [unwired: 1 out]
            }
          }
          frame #6 {
            n539 = Wait (ms)(milliseconds to wait=u32 2000) -> ()  [unwired: 1 out]
            n540 = property on="Trap delta" class="DigNum (strict)"("Val(Sgnl)"="Offset @ Delta (V)") -> ()  [unwired: 2 in, 2 out]
          }
          frame #7 {
            # "Only continue if there is no buffer\noverflow error"
            n541 = local read "Buffer Overflow"() -> (w898:bool)
            n542 = Not(x=w898) -> (.not. x?=w897:bool)
            n543 = case shown="True" w897 {
              frame False {
              }
              frame True {
                n544 = property on="Raster scan" class="Bool (strict)"("Val(Sgnl)"=TRUE ("Value (Signaling)")) -> ()  [unwired: 2 in, 2 out]
              }
            }
          }
          frame #8 {
            n545 = case shown="True" w900 {
              frame False {
              }
              frame True {
                n546 = Wait (ms)(milliseconds to wait=u32 2000) -> ()  [unwired: 1 out]
              }
            }
          }
          frame #9 {
            n547 = case shown="True" w902 {
              frame False {
              }
              frame True {
                n548 = while {
                  stop <- w904 stop-if-true
                  n549 = local read "Saving"() -> (w905:bool)
                  n550 = Not(x=w905) -> (.not. x?=w904:bool)
                  n551 = Wait (ms)(milliseconds to wait=u32 100) -> ()  [unwired: 1 out]
                }
              }
            }
          }
          frame #10 {
            n552 = case shown="True" w906 {
              frame False {
              }
              frame True {
                n553 = property on="Read Cal" class="Bool (strict)"("Val(Sgnl)"=TRUE ("Value (Signaling)")) -> ()  [unwired: 2 in, 2 out]
              }
            }
          }
          frame #11 {
            n554 = case shown="True" w908 {
              frame False {
              }
              frame True {
                n555 = Wait (ms)(milliseconds to wait=u32 1000) -> ()  [unwired: 1 out]
              }
            }
          }
          frame #12 {
            n556 = case shown="True" w910 {
              frame False {
              }
              frame True {
                n557 = property on="Fish" class="Bool (strict)"("Val(Sgnl)"=TRUE ("Value (Signaling)")) -> ()  [unwired: 2 in, 2 out]
                n558 = case shown="True" "Flow on\nwhile fish?" {
                  frame False {
                  }
                  frame True {
                    n559 = property on="Inject Sample" class="Bool (strict)"("Val(Sgnl)"=TRUE ("Value (Signaling)")) -> ()  [unwired: 2 in, 2 out]
                  }
                }
              }
            }
          }
        }
      }
      event "Dump beads": Value Change {
        n560 = event-data() -> ()  [unwired: 1 in, 5 out]
        n561 = flat-sequence {
          tunnel: w916 -> [w920]
          tunnel: w917 -> [w921]
          tunnel: [w921] -> w915
          tunnel: [w920] -> w914
          tunnel: w915 -> [w924]
          tunnel: w914 -> [w923]
          frame #0 {
            w918 = FALSE ("Fish")
            n562 = local read "Saving"() -> (w919:bool)
            n563 = local write "Pause dwell"(w918) -> ()
            n564 = local write "Force Feedback"(w918) -> ()
            n565 = local write "Dump beads"(w918) -> ()
            n566 = property on="Stop saving" class="Bool (strict)"("Val(Sgnl)"=w919) -> ()  [unwired: 2 in, 2 out]
            n567 = local write "Fish"(w918) -> ()
          }
          frame #1 {
            n568 = local read "Saved stage positions"() -> (w926:dbl[][])
            n569 = case shown="True" "Flow on\ndump?" {
              frame False {
              }
              frame True {
                n570 = property on="Inject Sample" class="Bool (strict)"("Val(Sgnl)"=TRUE ("Value (Signaling)")) -> ()  [unwired: 2 in, 2 out]
              }
            }
            n571 = local write "Stage moving"(TRUE ("Stage moving")) -> ()
            n572 = call "move to saved stage position.vi"("error in"=w923, "Stage VISA resource name in"=w924, "Position"=5, "Saved Stage Positions"=w926) -> ()  [unwired: 2 out]
          }
          frame #2 {
            n573 = local read "Shutter 1 (B)"() -> (w931:bool)
            n574 = local read "Shutter 2 (A)"() -> (w930:bool)
            n575 = call <vilib>:"Beep.vi"() -> ()  [unwired: 12 in]
            n576 = case shown="True" w931 {
              frame False {
              }
              frame True {
                n577 = property on="Shutter 1 (B)" class="Bool (strict)"("Val(Sgnl)"=FALSE ("Value (Signaling)")) -> ()  [unwired: 2 in, 2 out]
              }
            }
            n578 = case shown="True" w930 {
              frame False {
              }
              frame True {
                n579 = property on="Shutter 2 (A)" class="Bool (strict)"("Val(Sgnl)"=FALSE) -> ()  [unwired: 2 in, 2 out]
              }
            }
            n580 = local write "Stage moving"(FALSE ("Stage moving")) -> ()
            n581 = local write "Tether"(FALSE ("Tether")) -> ()
          }
          frame #3 {
            n582 = property on="Move Cap. 2 (ADig Top)" class="Bool (strict)"("Val(Sgnl)"=TRUE ("Value (Signaling)")) -> ()  [unwired: 2 in, 2 out]
          }
        }
      }
      event "Move Cap. 2 (ADig Top)": Value Change {
        n583 = event-data() -> ()  [unwired: 1 in, 5 out]
        n584 = flat-sequence {
          tunnel: w937 -> [w941]
          tunnel: w936 -> [w940]
          frame #0 {
            n585 = local read "Saved stage positions"() -> (w939:dbl[][])
            n586 = case shown="True" "Flow on\ncap 2?" {
              frame False {
              }
              frame True {
                n587 = property on="Inject Sample" class="Bool (strict)"("Val(Sgnl)"=TRUE ("Value (Signaling)")) -> ()  [unwired: 2 in, 2 out]
              }
            }
            n588 = local write "Move Cap. 2 (ADig Top)"(FALSE ("Move Cap. 2 (ADig Top)")) -> ()
            n589 = local write "Stage moving"(TRUE ("Stage moving")) -> ()
            n590 = call "move to saved stage position.vi"("error in"=w940, "Stage VISA resource name in"=w941, "Position"=2, "Saved Stage Positions"=w939) -> ()  [unwired: 2 out]
          }
          frame #1 {
            # "Make sure you don't reverse\nwhich is ON and OFF"
            n591 = local read "Cal @ Delta (V)"() -> (w948:dbl)
            n592 = local write "Stage moving"(FALSE ("Stage moving")) -> ()
            n593 = call <vilib>:"Beep.vi"() -> ()  [unwired: 12 in]
            n594 = property on="Trap delta" class="DigNum (strict)"("Val(Sgnl)"=w948) -> ()  [unwired: 2 in, 2 out]
            n595 = disable-structure shown="Disabled" {
              frame Disabled {
                n596 = property on="Inject Pump 1" class="Bool (strict)"("Val(Sgnl)"=TRUE ("Inject Pump 2")) -> ()  [unwired: 2 in, 2 out]
              }
              frame Enabled {
              }
            }
            n597 = local read "Shutter 2 (A)"() -> (w947:bool)
            n598 = case shown="False" w947 {
              frame False {
                n599 = property on="Shutter 2 (A)" class="Bool (strict)"("Val(Sgnl)"=TRUE ("Value (Signaling)")) -> ()  [unwired: 2 in, 2 out]
              }
              frame True {
              }
            }
            n600 = property on="Inject Sample" class="Bool (strict)"("Val(Sgnl)"=FALSE ("Value (Signaling)")) -> ()  [unwired: 2 in, 2 out]
          }
        }
      }
      event "Got ADig bead": Value Change {
        n601 = event-data() -> ()  [unwired: 1 in, 5 out]
        n602 = flat-sequence {
          tunnel: w954 -> [w958]
          tunnel: w953 -> [w957]
          frame #0 {
            n603 = local read "Saved stage positions"() -> (w960:dbl[][])
            n604 = property on="Inject Pump 1" class="Bool (strict)"("Val(Sgnl)"=FALSE ("Inject Pump 2")) -> ()  [unwired: 2 in, 2 out]
            n605 = case shown="True" "Flow on\ncap 1?" {
              frame False {
              }
              frame True {
                n606 = property on="Inject Sample" class="Bool (strict)"("Val(Sgnl)"=TRUE ("Value (Signaling)")) -> ()  [unwired: 2 in, 2 out]
              }
            }
            n607 = local write "Stage moving"(TRUE ("Stage moving")) -> ()
            n608 = call "move to saved stage position.vi"("error in"=w957, "Stage VISA resource name in"=w958, "Position"=1, "Saved Stage Positions"=w960) -> ()  [unwired: 2 out]
          }
          frame #1 {
            n609 = local read "Shutter 1 (B)"() -> (w964:bool)
            n610 = disable-structure shown="Disabled" {
              frame Disabled {
                n611 = property on="Inject Pump 2" class="Bool (strict)"("Val(Sgnl)"=TRUE ("Inject Pump 2")) -> ()  [unwired: 2 in, 2 out]
              }
              frame Enabled {
              }
            }
            n612 = local write "Stage moving"(FALSE ("Stage moving")) -> ()
            n613 = case shown="False" w964 {
              frame False {
                n614 = property on="Shutter 1 (B)" class="Bool (strict)"("Val(Sgnl)"=TRUE ("Value (Signaling)")) -> ()  [unwired: 2 in, 2 out]
              }
              frame True {
              }
            }
            n615 = property on="Inject Sample" class="Bool (strict)"("Val(Sgnl)"=FALSE ("Value (Signaling)")) -> ()  [unwired: 2 in, 2 out]
            n616 = call <vilib>:"Beep.vi"() -> ()  [unwired: 12 in]
          }
        }
        n617 = local write "Got ADig bead"(FALSE ("Got ADig bead")) -> ()
      }
      event "Set Position 1", "Set Position 2", "Set Position 3", "Set Position 4", "Set Position 5": Value Change {
        n618 = event-data() -> ()  [unwired: 1 in, 5 out]
        n619 = Build Array("Set Position 1", "Set Position 2", "Set Position 3", "Set Position 4", "Set Position 5") -> (w983:bool[])
        n620 = Boolean Array To Number(Boolean array=w983) -> (number=w982:u32)
        n621 = call "Read Stage Position.vi"("error in"=w970, "VISA resource name in"=w971) -> ("Current Position"=w968:cluster{dbl, dbl, dbl}, "error out"=→"Stage error":errorcluster)  [unwired: 1 in, 1 out]
        n622 = Logarithm Base 2(1:w982) -> (0:w976:dbl)
        n623 = Cluster To Array(cluster=w968) -> (array=w978:dbl[])
        n624 = Increment(x=w976) -> (x+1=w979:dbl)
        n625 = Build Array (concatenate)(w979, w978) -> (w977:dbl[])
        n626 = Replace Array Subset(array="Saved stage positions", new element=w977, index (row)=w976) -> (w980:dbl[][])  [unwired: 1 in]
        n627 = local write "Saved stage positions"(w980) -> ()
      }
      event "Move to Position 2", "Move to Position 4", "Move to Position 3", "Move to Position 5", "Move to Position 1": Value Change {
        n628 = event-data() -> ()  [unwired: 1 in, 5 out]
        n629 = Build Array("Move to Position 1", "Move to Position 2", "Move to Position 3", "Move to Position 4", "Move to Position 5") -> (w993:bool[])
        n630 = Boolean Array To Number(Boolean array=w993) -> (number=w992:u32)
        n631 = Logarithm Base 2(1:w992) -> (0:w991:dbl)
        n632 = flat-sequence {
          tunnel: w991 -> [w998]
          tunnel: w990 -> [w997]
          tunnel: w989 -> [w996]
          frame #0 {
            n633 = local read "Saved stage positions"() -> (w999:dbl[][])
            n634 = Increment(x=w998) -> (x+1=w995:dbl)
            n635 = call "move to saved stage position.vi"("error in"=w996, "Stage VISA resource name in"=w997, "Position"=w995, "Saved Stage Positions"=w999) -> ()  [unwired: 2 out]
            "Stage moving" <- TRUE ("Stage moving")
          }
          frame #1 {
            n636 = call <vilib>:"Beep.vi"() -> ()  [unwired: 12 in]
            n637 = local write "Stage moving"(FALSE ("Stage moving")) -> ()
          }
        }
      }
      event "Dip": Value Change {
        n638 = event-data() -> ()  [unwired: 1 in, 5 out]
        n639 = local write "Dip"(FALSE ("Dip")) -> ()
        n640 = flat-sequence {
          tunnel: w1010 -> [w1012]
          tunnel: w1009 -> [w1011]
          tunnel: [w1013] -> w1007
          tunnel: [w1012] -> w1005
          tunnel: [w1011] -> w1003
          tunnel: [w1021] -> w1008
          tunnel: w1007 -> [w1021]
          tunnel: [w1020] -> w1006
          tunnel: w1005 -> [w1020]
          tunnel: [w1019] -> w1004
          tunnel: w1003 -> [w1019]
          tunnel: w1008 -> [w1040]
          tunnel: w1006 -> [w1039]
          tunnel: w1004 -> [w1038]
          frame #0 {
            n641 = local read "Saved stage positions"() -> (w1013:dbl[][])
            n642 = local write "Stage moving"(TRUE) -> ()
            n643 = call "move to saved stage position.vi"("error in"=w1011, "Stage VISA resource name in"=w1012, "Position"="Dip position", "Saved Stage Positions"=w1013) -> ()  [unwired: 2 out]
          }
          frame #1 {
            n644 = node-c288() -> (w1018:T12)  [unwired: 4 in]
            n645 = timed-loop {
              timing: w1018 -> [_]
              timing-out: [_] -> w1017
              i -> [w1031]
              stop <- w1022 stop-if-true
              n646 = node-c288() -> ()  [unwired: 1 in, 1 out]
              n647 = Greater Or Equal?(x=w1031, y="Dip duration") -> (x >= y?=w1027:bool)
              n648 = local read "Dump beads"() -> (w1024:bool)
              n649 = Or(x=w1027, y="Cancel dwell") -> (x .or. y?=w1025:bool)
              n650 = Not(x="Pause dwell") -> (.not. x?=w1028:bool)
              n651 = node-c288() -> ()  [unwired: 1 in, 1 out]
              n652 = And(x=w1028, y=w1025) -> (x .and. y?=w1023:bool)
              n653 = Or(x=w1023, y=w1024) -> (x .or. y?=w1022:bool)
              "Dip time" <- w1031
            }
            n654 = local write "Stage moving"(FALSE ("Stage moving")) -> ()
            n655 = node-c288(w1017) -> ()  [unwired: 1 out]
          }
          frame #2 {
            n656 = local write "Cancel dwell"(FALSE ("Cancel dwell")) -> ()
            n657 = call "move to saved stage position.vi"("error in"=w1038, "Stage VISA resource name in"=w1039, "Position"="Return position", "Saved Stage Positions"=w1040) -> ()  [unwired: 2 out]
          }
          frame #3 {
            n658 = local write "Stage moving"(FALSE ("Stage moving")) -> ()
          }
        }
      }
      event "Force FB script": Value Change {
        n659 = event-data() -> ()  [unwired: 1 in, 5 out]
        n660 = flat-sequence {
          frame #0 {
            n661 = disable-structure shown="Disabled" {
              frame Disabled {
                n662 = local read "# Samples/channel"() -> (w1044:i32)
                n663 = local write "# Samples/channel (in)"(w1044) -> ()
              }
              frame Enabled {
              }
            }
            n664 = local write "Force FB script"(FALSE ("Force FB script")) -> ()
            n665 = property on="Trap delta" class="DigNum (strict)"("Val(Sgnl)"="Start trap delta (V)") -> ()  [unwired: 2 in, 2 out]
          }
          frame #1 {
            n666 = Wait (ms)(milliseconds to wait=u32 500) -> ()  [unwired: 1 out]
          }
          frame #2 {
            n667 = property on="Set reading to\nsetpoint" class="Bool (strict)"("Val(Sgnl)"=TRUE ("Value (Signaling)")) -> ()  [unwired: 2 in, 2 out]
          }
          frame #3 {
            n668 = Wait (ms)(milliseconds to wait=u32 300) -> ()  [unwired: 1 out]
          }
          frame #4 {
            n669 = local write "Force Feedback"(TRUE ("Force Feedback")) -> ()
            n670 = property on="Tabs" class="TabCtl (strict)"("Val(Sgnl)"=T3."Force Feedback" ("Value (Signaling)")) -> ()  [unwired: 2 in, 2 out]
          }
          frame #5 {
            n671 = property on="Save Data" class="Bool (strict)"("Val(Sgnl)"=TRUE ("Value (Signaling)")) -> ()  [unwired: 2 in, 2 out]
          }
          frame #6 {
            n672 = Multiply(x="Wait before dip (s)", y=1000) -> (x*y=w1051:dbl)
            n673 = Wait (ms)(milliseconds to wait=w1051) -> ()  [unwired: 1 out]
          }
          frame #7 {
            n674 = case shown="True" "Start dipping after?" {
              selector: "Start dipping after?" -> [_ w1056]
              frame False {
              }
              frame True {
                n675 = property on="Dip" class="Bool (strict)"("Val(Sgnl)"=w1056) -> ()  [unwired: 2 in, 2 out]
              }
            }
            n676 = property on="Remove offsets" class="Bool (strict)"("Val(Sgnl)"=TRUE ("Value (Signaling)")) -> ()  [unwired: 2 in, 2 out]
          }
        }
      }
      event "Move 0": Value Change {
        n677 = event-data() -> ()  [unwired: 1 in, 5 out]
        n678 = local write "Move 0"(FALSE) -> ()
        n679 = call "HalfWavePlate.vi"("Degrees"="\"Degrees\" 0", "Motor"=0) -> ()  [unwired: 1 in]
      }
      event "Move 1": Value Change {
        n680 = event-data() -> ()  [unwired: 1 in, 5 out]
        n681 = local write "Move 1"(FALSE) -> ()
        n682 = call "HalfWavePlate.vi"("Degrees"="\"Degrees\" 1", "Motor"=1) -> ()  [unwired: 1 in]
      }
      event "Stop": Value Change {
        n683 = event-data() -> ()  [unwired: 1 in, 5 out]
        n684 = local read "Stop"() -> (w1063:bool)
      }
    }
    n685 = node-c288() -> ()  [unwired: 1 in, 1 out]
  }
  n686 = node-c288(2 ("Processor")) -> (w75:T12)  [unwired: 3 in]
  n687 = node-c288(2 ("Processor")) -> (w27:T12)  [unwired: 3 in]
  n688 = timed-loop {
    timing: w75 -> [_]
    timing-out: [_] -> w74
    stop <- w1066 stop-if-true
    n689 = node-c288() -> ()  [unwired: 1 in, 1 out]
    n690 = case shown="\"Current Saved Data\"" "Tab Control" {
      frame "Control" {
        n691 = case shown="True" "Start" {
          frame False {
          }
          frame True {
            w1079 = T15 3 items=["no dialog", "OK message", "continue or stop message", "OK message + warnings", "continue/stop + warnings"] ("type of dialog (OK msg:1)")
            n692 = call "InitializeAcquireFF.vi"("DAQ Rate"="DAQ Rate", "Averaging Number"="Averaging Number", "Sampling Rate"="Sampling Rate") -> ("error out"=w1073:errorcluster, "task out"=w1072:refnum<k21>, "Final Sampling Rate"=→"Final Sampling Rate":dbl)  [unwired: 4 in, 2 out]
            n693 = while {
              tunnel: [w1091] -> w1078
              tunnel: [w1090] -> w1071
              tunnel: "Averaging Number" -> [w1089]
              tunnel: w1073 -> [w1088]
              tunnel: w1072 -> [w1086]
              stop <- w1087 continue-if-true
              n694 = call "Acquire2_QPD.vi"("task/channels in"=w1086, "Save Data?"=FALSE ("Take Data?"), "Averaging Number"=w1089, "error in"=w1088) -> ("PSD 1"=→"PSD 1":cluster{dbl[], dbl[]}, "PSD 1 Sum"=→"PSD 1 Sum":dbl, "PSD 2"=→"PSD 2":cluster{dbl[], dbl[]}, "PSD 2 Sum"=→"PSD 2 Sum":dbl, "task out"=w1091:refnum<k21>, "error out"=w1090:errorcluster)  [unwired: 14 in, 4 out]
              n695 = local read "Start"() -> (w1087:bool)
            }
            n696 = call <vilib>:"DAQmx Clear Task.vi"("task in"=w1078, "error in"=w1071) -> ("error out"=w1080:errorcluster)  [unwired: 13 in]
            n697 = call <vilib>:"Simple Error Handler.vi"("type of dialog (OK msg:1)"=w1079, "error in (no error)"=w1080) -> ()  [unwired: 3 in, 5 out]
          }
        }
      }
      frame "Current Saved Data" {
      }
      frame "Data Acquisition" {
      }
      frame "Raw QPD Data" {
      }
    }
    n698 = local read "Stop"() -> (w1066:bool)
    n699 = node-c288() -> ()  [unwired: 1 in, 1 out]
  }
  n700 = call-poly <vilib>:"DAQmx Create Virtual Channel.vi"("lines"=w92) -> ("task out"=w91:refnum<k21>)  [unwired: 13 in, 1 out]
  n701 = call-poly <vilib>:"DAQmx Create Virtual Channel.vi"("lines"=w95) -> ("task out"=w94:refnum<k21>)  [unwired: 13 in, 1 out]
  n702 = timed-loop {
    timing: w27 -> [_]
    timing-out: [_] -> w26
    stop <- w1092 stop-if-true
    n703 = node-c288() -> ()  [unwired: 1 in, 1 out]
    n704 = event shown="[0] \"Pause Mouse/Mirror Connection\": Value Change" {
      selector: _ -> [_ _]
      dyn-events: _ -> [_ _]
      timeout: _ -> [_ _]
      tunnel: [w1185 _] -> w1093
      tunnel: [_ w1186] -> w1092
      event "Pause Mouse/Mirror Connection": Value Change {
        n705 = event-data() -> ("NewVal"=w1185:bool)  [unwired: 1 in]
      }
      event "Stop": Value Change {
        n706 = event-data() -> ("NewVal"=w1186:bool)  [unwired: 1 in]
      }
    }
    n707 = case shown="True" w1093 {
      frame False {
      }
      frame True {
        n708 = call "InitializeMouseControl.vi"() -> ("error out 2"=w1102:errorcluster, "task out"=w1103:refnum<k21>, "error out"=w1105:errorcluster, "device ID"=w1104:refnum<k1>)  [unwired: 8 in]
        n709 = while {
          tunnel: w1105 -> [w1117]
          tunnel: w1104 -> [w1116]
          tunnel: w1103 -> [w1115]
          tunnel: w1102 -> [w1114]
          tunnel: [w1113] -> w1100
          tunnel: [w1112] -> w1099
          tunnel: [w1111] -> w1096
          tunnel: [w1110] -> w1097
          stop <- w1109 stop-if-true
          n710 = case shown="True" "Use Mouse to Move Trap?" {
            tunnel: w1116 -> [w1124 w1147]
            tunnel: w1117 -> [w1123 w1146]
            tunnel: w1115 -> [w1122 w1145]
            tunnel: w1114 -> [w1121 w1144]
            tunnel: [w1124 w1143] -> w1111
            tunnel: [w1123 w1142] -> w1110
            tunnel: [w1122 w1141] -> w1113
            tunnel: [w1121 w1140] -> w1112
            frame False {
              (unwired) FALSE ("button 1")
            }
            frame True {
              w1135 = 0.0 ("y")
              w1137 = 10
              n711 = local read "Deflection"() -> (w1148:T4)
              n712 = call-poly <vilib>:"Acquire Input Data.vi"("device ID"=w1147, "error in (no error)"=w1146) -> ("device ID"=w1143:refnum<k1>, "button info"=w1161:T16, "error out"=w1142:errorcluster)  [unwired: 14 in, 1 out]
              n713 = Unbundle By Name(w1148) -> ("Horizontal"=w1150:i32, "Vertical"=w1149:i32)
              n714 = local read "Saved voltage"() -> (w1126:cluster{dbl, dbl})
              n715 = Divide(x=w1150, y=30) -> (x/y=w1153:dbl)
              n716 = Divide(x=w1149, y=-20) -> (x/y=w1154:dbl)
              n717 = Unbundle By Name(w1161) -> ("button 1"=w1139:bool, "button 2"=w1155:bool)
              n718 = Bundle(w1153, w1154) -> (w1131:cluster{dbl, dbl})  [unwired: 1 in]
              n719 = local write "Reference Voltage"(w1131) -> ()
              n720 = Add(x=w1131, y=w1126) -> (x+y=w1159:cluster{dbl, dbl})
              n721 = case shown="True" w1139 {
                frame False {
                  n722 = stacked-sequence {
                    frame #0 {
                      n723 = local write "CoordinatesMousePressed"(T4 {"Horizontal"=0, "Vertical"=0} ("Coords when pressed")) -> ()
                      n724 = local write "Deflection"(T4 {"Horizontal"=0, "Vertical"=0} ("deflaction")) -> ()
                    }
                  }
                }
                frame True {
                  n725 = local read "CoordinatesMousePressed"() -> (w1184:T4)
                  n726 = local read "Real Coordinates"() -> (w1183:cluster{"Horizontal":i32, "Vertical":i32})
                  n727 = Subtract(x=w1183, y=w1184) -> (x-y=w1182:T4)
                  n728 = local write "Deflection"(w1182) -> ()
                }
              }
              n729 = Unbundle(w1159) -> (w1136:dbl, w1127:dbl)
              n730 = case shown="True" w1155 {
                frame False {
                }
                frame True {
                  n731 = local read "Reference Voltage"() -> (w1165:cluster{dbl, dbl})
                  n732 = local read "Saved voltage"() -> (w1163:cluster{dbl, dbl})
                  n733 = Add(x=w1165, y=w1163) -> (x+y=→"Saved voltage":cluster{dbl, dbl})
                  n734 = local read "Real Coordinates"() -> (w1164:cluster{"Horizontal":i32, "Vertical":i32})
                  n735 = local write "CoordinatesMousePressed"(w1164) -> ()
                }
              }
              n736 = Less?(x=w1136, y=w1137) -> (x < y?=w1134:bool)
              n737 = Greater?(x=w1136, y=w1135) -> (0:w1133:bool)
              n738 = Greater?(x=w1127, y=w1135) -> (0:w1129:bool)
              n739 = Less?(x=w1127, y=w1137) -> (x < y?=w1130:bool)
              n740 = And(x=w1129, y=w1130) -> (x .and. y?=w1128:bool)
              n741 = And(x=w1134, y=w1133) -> (x .and. y?=w1132:bool)
              n742 = case shown="False" w1128 {
                tunnel: [w1175 w1179] -> w1138
                tunnel: w1127 -> [w1173 w1179]
                frame False {
                  n743 = Greater?(x=w1173, y=10.0) -> (0:w1176:bool)
                  n744 = case shown="True" w1176 {
                    tunnel: [0.0 10.0] -> w1175
                    frame False {
                    }
                    frame True {
                    }
                  }
                }
                frame True {
                }
              }
              n745 = case shown="False" w1132 {
                tunnel: w1136 -> [w1167 w1172]
                tunnel: [w1168 w1172] -> w1160
                frame False {
                  n746 = Greater?(x=w1167, y=10.0) -> (0:w1169:bool)
                  n747 = case shown="True" w1169 {
                    tunnel: [0.0 10.0] -> w1168
                    frame False {
                    }
                    frame True {
                    }
                  }
                }
                frame True {
                }
              }
              n748 = Bundle(w1160, w1138) -> (w1125:cluster{dbl, dbl})  [unwired: 1 in]
              n749 = Cluster To Array(cluster=w1125) -> (array=w1156:dbl[])
              n750 = call-poly <vilib>:"DAQmx Write.vi"("task/channels in"=w1145, "data"=w1156, "error in"=w1144) -> ("task out"=w1158:refnum<k21>, "error out"=w1157:errorcluster)  [unwired: 10 in, 1 out]
              n751 = call <vilib>:"DAQmx Is Task Done.vi"("task/channels in"=w1158, "error in"=w1157) -> ("task out"=w1141:refnum<k21>, "error out"=w1140:errorcluster)  [unwired: 11 in, 1 out]
            }
          }
          n752 = event shown="[0] \"Pane\": Mouse Move" {
            selector: _ -> [_ _ _]
            dyn-events: _ -> [_ _ _]
            timeout: _ -> [_ _ _]
            event Mouse Move {
              n753 = event-data() -> ("Coords"=w1119:T4)  [unwired: 1 in]
              n754 = local write "Real Coordinates"(w1119) -> ()
            }
            event Mouse Down {
              n755 = event-data() -> ("Coords"=w1120:T4)  [unwired: 1 in]
              n756 = local write "CoordinatesMousePressed"(w1120) -> ()
            }
            event "Pause Mouse/Mirror Connection": Value Change {
              n757 = event-data() -> ()  [unwired: 1 in, 3 out]
            }
          }
          n758 = local read "Stop"() -> (w1106:bool)
          n759 = Not(x="Pause Mouse/Mirror Connection") -> (.not. x?=w1107:bool)
          n760 = Or(x=w1107, y=w1106) -> (x .or. y?=w1109:bool)
        }
        n761 = call <vilib>:"DAQmx Clear Task.vi"("task in"=w1100, "error in"=w1099) -> ("error out"=w1101:errorcluster)  [unwired: 13 in]
        n762 = call <vilib>:"Simple Error Handler.vi"("error in (no error)"=w1101) -> ()  [unwired: 4 in, 5 out]
        n763 = call-poly <vilib>:"Close Input Device.vi"("error in (no error)"=w1097, "device ID"=w1096) -> ("error out"=w1098:errorcluster)  [unwired: 8 in]
        n764 = call <vilib>:"Simple Error Handler.vi"("error in (no error)"=w1098) -> ()  [unwired: 4 in, 5 out]
      }
    }
    n765 = node-c288() -> ()  [unwired: 1 in, 1 out]
  }
  n766 = node-c288(i64 100 ("Period")) -> (w89:T12)  [unwired: 3 in]
  n767 = timed-loop {
    tunnel: w91 -> [w1189]
    tunnel: [w1188] -> w90
    tunnel: w94 -> [w1191]
    tunnel: [w1190] -> w93
    timing: w89 -> [_]
    timing-out: [_] -> w88
    stop <- w1187 stop-if-true
    n768 = node-c288() -> ()  [unwired: 1 in, 1 out]
    n769 = event shown="[1] \"Shutter 2 (A)\": Value Change" {
      selector: _ -> [_ _ _]
      dyn-events: _ -> [_ _ _]
      timeout: _ -> [_ _ _]
      tunnel: w1191 -> [w1195 _ _]
      tunnel: [w1194 _ _] -> w1190
      tunnel: w1189 -> [_ w1215 _]
      tunnel: [_ w1213 _] -> w1188
      tunnel: [_ _ w1232] -> w1187
      event "Shutter 1 (B)": Value Change {
        n770 = event-data() -> ()  [unwired: 1 in, 1 out]
        n771 = flat-sequence {
          tunnel: [w1201] -> w1198
          tunnel: w1195 -> [w1200]
          tunnel: [w1205] -> w1197
          tunnel: [w1208] -> w1196
          tunnel: w1198 -> [w1203]
          tunnel: w1197 -> [w1212]
          tunnel: w1196 -> [w1210]
          tunnel: [w1209] -> w1194
          frame #0 {
            n772 = call-poly <vilib>:"DAQmx Write.vi"("task/channels in"=w1200, "data"=FALSE) -> ("task out"=w1201:refnum<k21>)  [unwired: 11 in, 2 out]
            n773 = Wait (ms)(milliseconds to wait=100) -> ()  [unwired: 1 out]
          }
          frame #1 {
            n774 = Or(x="Shutter 1 (B)", y=TRUE) -> (x .or. y?=w1205:bool)
            n775 = call-poly <vilib>:"DAQmx Write.vi"("task/channels in"=w1203, "data"=w1205) -> ("task out"=w1208:refnum<k21>)  [unwired: 11 in, 2 out]
            n776 = Wait (ms)(milliseconds to wait=100) -> ()  [unwired: 1 out]
          }
          frame #2 {
            n777 = Not(x=w1212) -> (.not. x?=w1211:bool)
            n778 = call-poly <vilib>:"DAQmx Write.vi"("task/channels in"=w1210, "data"=w1211) -> ("task out"=w1209:refnum<k21>)  [unwired: 11 in, 2 out]
          }
        }
      }
      event "Shutter 2 (A)": Value Change {
        n779 = event-data() -> ()  [unwired: 1 in, 1 out]
        n780 = flat-sequence {
          tunnel: w1215 -> [w1220]
          tunnel: [w1219] -> w1214
          tunnel: [w1224] -> w1217
          tunnel: [w1227] -> w1216
          tunnel: w1214 -> [w1222]
          tunnel: w1217 -> [w1231]
          tunnel: w1216 -> [w1229]
          tunnel: [w1228] -> w1213
          frame #0 {
            n781 = call-poly <vilib>:"DAQmx Write.vi"("task/channels in"=w1220, "data"=FALSE) -> ("task out"=w1219:refnum<k21>)  [unwired: 11 in, 2 out]
            n782 = Wait (ms)(milliseconds to wait=100) -> ()  [unwired: 1 out]
          }
          frame #1 {
            n783 = Or(x="Shutter 2 (A)", y=TRUE) -> (x .or. y?=w1224:bool)
            n784 = call-poly <vilib>:"DAQmx Write.vi"("task/channels in"=w1222, "data"=w1224) -> ("task out"=w1227:refnum<k21>)  [unwired: 11 in, 2 out]
            n785 = Wait (ms)(milliseconds to wait=100) -> ()  [unwired: 1 out]
          }
          frame #2 {
            n786 = Not(x=w1231) -> (.not. x?=w1230:bool)
            n787 = call-poly <vilib>:"DAQmx Write.vi"("task/channels in"=w1229, "data"=w1230) -> ("task out"=w1228:refnum<k21>)  [unwired: 11 in, 2 out]
          }
        }
      }
      event "Stop": Value Change {
        n788 = event-data() -> ("NewVal"=w1232:bool)  [unwired: 1 in, 5 out]
      }
    }
    n789 = node-c288() -> ()  [unwired: 1 in, 1 out]
  }
  n790 = node-c288(w88) -> ()  [unwired: 1 out]
  n791 = node-c288(w74) -> ()  [unwired: 1 out]
  n792 = call <vilib>:"DAQmx Clear Task.vi"("task in"=w90) -> ()  [unwired: 14 in, 1 out]
  n793 = call <vilib>:"DAQmx Clear Task.vi"("task in"=w93) -> ()  [unwired: 14 in, 1 out]
  n794 = node-c288(w26) -> ()  [unwired: 1 out]
  n795 = node-c288(w22) -> ()  [unwired: 1 out]
  n796 = local write "Tether"(FALSE ("Tether")) -> ()
  n797 = local read "Path"() -> (w81:path)
  n798 = node-c288(i64 1 ("Period"), 2 ("Processor")) -> (w87:T12)  [unwired: 2 in]
  n799 = VISA Close(VISA resource name=w19) -> (error out=w104:errorcluster)  [unwired: 1 in]
  n800 = timed-loop {
    timing: w87 -> [_]
    timing-out: [_] -> w86
    tunnel: w81 -> [w1234]
    stop <- w1233 stop-if-true
    n801 = node-c288() -> ()  [unwired: 1 in, 1 out]
    n802 = event shown="[5] \"Fish\": Value Change" {
      selector: _ -> [_ _ _ _ _ _ _ _ _]
      dyn-events: _ -> [_ _ _ _ _ _ _ _ _]
      timeout: _ -> [_ _ _ _ _ _ _ _ _]
      tunnel: w1234 -> [_ w1238 _ _ _ _ _ _ _]
      tunnel: [_ _ w1258 _ _ _ _ _ _] -> w1233
      event Timeout {
        n803 = event-data() -> ()  [unwired: 1 in, 2 out]
      }
      event "Read Cal": Value Change {
        n804 = event-data() -> ()  [unwired: 1 in, 6 out]
        n805 = Path To String(path=w1238) -> (string=w1237:string)
        n806 = Format Date/Time String(time format string (%c)="%y%m%d") -> (date/time string=w1239:string)  [unwired: 2 in]
        n807 = Concatenate Strings(w1237, "\\" ("string"), w1239, "\\" ("string"), "current.cal") -> (w1257:string)
        n808 = String To Path(string=w1257) -> (path=w1256:path)
        n809 = Open/Create/Replace File(file path (use dialog)=w1256, operation (0:open)=T9."open", access (0:read/write)=enum16{"read/write", "read-only", "write-only"}."read-only") -> (refnum out=w1252:refnum<file>, error out=w1253:errorcluster)  [unwired: 3 in, 1 out]
        n810 = Deny Access(4:w1253, 7:w1252) -> (0:w1251:errorcluster, 3:w1250:refnum<file>)  [unwired: 1 in]
        n811 = Read from Binary File(5:0.0, 8:w1251, 9:T10."big-endian, network order" ("byte order (0:big-endian, network order)"), 10:12 ("count"), 11:w1250) -> (0:w1246:errorcluster, 2:w1244:dbl[], 3:w1247:refnum<file>)  [unwired: 1 in, 1 out]
        n812 = Array To Cluster(array=w1244) -> (cluster=→"Cal values":T17)
        n813 = Close File(refnum=w1247, error in=w1246) -> ()  [unwired: 2 out]
        n814 = local write "Read Cal"(FALSE ("Read Cal")) -> ()
      }
      event "Stop": Value Change {
        n815 = event-data() -> ("NewVal"=w1258:bool)  [unwired: 1 in, 5 out]
      }
      event "Trap position": Value Change {
        # "Need to rotate so X and Y don't get mixed up."
        n816 = event-data() -> ()  [unwired: 1 in, 6 out]
        n817 = local read "Mirror task"() -> (w1259:refnum<k21>)
        n818 = Cluster To Array(cluster="Trap position") -> (array=w1262:dbl[])
        n819 = Rotate 1D Array(1:w1262, 2:1 ("n")) -> (0:w1260:dbl[])
        n820 = call-poly <vilib>:"DAQmx Write.vi"("task/channels in"=w1259, "data"=w1260) -> ("task out"=w1265:refnum<k21>, "error out"=w1264:errorcluster)  [unwired: 11 in, 1 out]
        n821 = call <vilib>:"DAQmx Stop Task.vi"("task/channels in"=w1265, "error in"=w1264) -> ("error out"=w1263:errorcluster)  [unwired: 12 in, 1 out]
        n822 = call <vilib>:"Simple Error Handler.vi"("error in (no error)"=w1263) -> ()  [unwired: 4 in, 5 out]
      }
      event "Trap delta": Value Change {
        n823 = event-data() -> ()  [unwired: 1 in, 6 out]
        n824 = local read "Pulling direction"() -> (w1268:bool)
        n825 = local read "Fixed Y"() -> (w1272:dbl)
        n826 = local read "Fixed X"() -> (w1271:dbl)
        n827 = Select(t=w1272, s=w1268, f=w1271) -> (s? t:f=w1270:dbl)
        n828 = Add(x="Trap delta", y=w1270) -> (x+y=w1267:dbl)
        n829 = case shown="True" w1268 {
          tunnel: w1267 -> [w1273 w1274]
          frame False {
            n830 = property on="X" class="DigNum (strict)"("Val(Sgnl)"=w1273) -> ()  [unwired: 2 in, 2 out]
          }
          frame True {
            n831 = property on="Y" class="DigNum (strict)"("Val(Sgnl)"=w1274) -> ()  [unwired: 2 in, 2 out]
          }
        }
      }
      event "Fish": Value Change {
        n832 = event-data() -> ()  [unwired: 1 in, 6 out]
        n833 = local read "Fish"() -> (w1275:bool)
        n834 = case shown="True" w1275 {
          frame False {
          }
          frame True {
            w1284 = 0.0 ("minimum value")
            w1285 = 10.0 ("maximum value")
            # "Grab offset in pulling\ndirection and add to \ndelta values"
            n835 = call-poly <vilib>:"DAQmx Create Virtual Channel.vi"("maximum value"=w1285, "minimum value"=w1284, "physical channels"=tag "Dev1/ao0") -> ("task out"=w1289:refnum<k21>, "error out"=w1288:errorcluster)  [unwired: 11 in]
            n836 = call-poly <vilib>:"DAQmx Create Virtual Channel.vi"("task in"=w1289, "maximum value"=w1285, "minimum value"=w1284, "physical channels"=tag "Dev1/ao1", "error in"=w1288) -> ("task out"=w1283:refnum<k21>, "error out"=w1282:errorcluster)  [unwired: 9 in]
            n837 = node-c288(i64 1 ("Period")) -> (w1291:T12)  [unwired: 3 in]
            n838 = timed-loop {
              timing: w1291 -> [_]
              timing-out: [_] -> w1290
              tunnel: w1283 -> [w1342]
              tunnel: w1282 -> [w1341]
              tunnel: [w1340] -> w1278
              tunnel: [w1339] -> w1277
              tunnel: [w1307] -> w1280
              tunnel: [w1321] -> w1276
              i -> [w1325]
              stop <- w1321 stop-if-true
              # "Send offset in direction\nof not-pulling to DAQ"
              n839 = node-c288() -> ()  [unwired: 1 in, 1 out]
              n840 = local read "Pulling direction"() -> (w1309:bool)
              n841 = local read "Fixed Y"() -> (w1311:dbl)
              n842 = local read "Fixed X"() -> (w1312:dbl)
              n843 = Select(t=w1311, s=w1309, f=w1312) -> (s? t:f=w1313:dbl)
              n844 = Add(x=w1313, y="Max fish\ndelta (V)") -> (x+y=w1315:dbl)
              n845 = Subtract(x="Max fish\ndelta (V)", y="Min fish\ndelta (V)") -> (x-y=w1317:dbl)
              n846 = Select(t=w1312, s=w1309, f=w1311) -> (s? t:f=w1310:dbl)
              n847 = Divide(x=w1317, y="Fish Speed (ms)") -> (x/y=w1318:dbl)
              n848 = flat-sequence {
                tunnel: w1309 -> [w1361]
                tunnel: w1310 -> [w1360]
                tunnel: w1342 -> [w1359]
                tunnel: w1341 -> [w1358]
                tunnel: w1318 -> [w1357]
                tunnel: w1315 -> [w1356]
                tunnel: "Fish Speed (ms)" -> [w1351]
                tunnel: [w1355] -> w1338
                tunnel: [w1354] -> w1337
                tunnel: [w1353] -> w1336
                tunnel: [w1352] -> w1335
                tunnel: [w1345] -> w1324
                tunnel: [w1344] -> w1308
                tunnel: [w1343] -> w1305
                tunnel: [w1408] -> w1334
                tunnel: w1338 -> [w1408]
                tunnel: [w1407] -> w1333
                tunnel: w1337 -> [w1407]
                tunnel: [w1406] -> w1332
                tunnel: w1336 -> [w1406]
                tunnel: [w1405] -> w1331
                tunnel: w1335 -> [w1405]
                tunnel: w1324 -> [w1404]
                tunnel: [w1404] -> w1323
                tunnel: w1308 -> [w1403]
                tunnel: [w1402] -> w1306
                tunnel: w1305 -> [w1402]
                tunnel: w1334 -> [w1419]
                tunnel: w1333 -> [w1418]
                tunnel: w1332 -> [w1417]
                tunnel: w1331 -> [w1416]
                tunnel: w1320 -> [w1415]
                tunnel: [w1414] -> w1340
                tunnel: [w1413] -> w1339
                tunnel: w1323 -> [w1412]
                tunnel: [w1411] -> w1307
                tunnel: w1306 -> [w1410]
                frame #0 {
                  n849 = local read "Mean force (pN)"() -> (w1350:dbl)
                  n850 = local read "Cutoff force (pN)"() -> (w1349:dbl)
                  n851 = Less Or Equal?(x=w1350, y=w1349) -> (x <= y?=w1347:bool)
                  n852 = And(x="Fish", y=w1347) -> (x .and. y?=w1348:bool)
                  n853 = case shown="True" w1348 {
                    selector: w1348 -> [w1363 _]
                    tunnel: w1361 -> [w1366 w1382]
                    tunnel: w1360 -> [_ w1381]
                    tunnel: w1359 -> [w1368 w1380]
                    tunnel: w1358 -> [w1367 w1379]
                    tunnel: w1357 -> [w1365 w1378]
                    tunnel: w1356 -> [w1364 w1377]
                    tunnel: [w1368 w1376] -> w1355
                    tunnel: [w1367 w1375] -> w1354
                    tunnel: [w1366 w1374] -> w1353
                    tunnel: [w1364 w1373] -> w1343
                    tunnel: [w1365 w1372] -> w1352
                    tunnel: w1351 -> [_ w1371]
                    tunnel: [w1363 w1370] -> w1345
                    tunnel: [FALSE w1369] -> w1344
                    frame False {
                    }
                    frame True {
                      n854 = while {
                        tunnel: w1382 -> [w1391]
                        tunnel: w1381 -> [w1390]
                        tunnel: w1380 -> [w1398]
                        tunnel: w1379 -> [w1397]
                        tunnel: w1378 -> [w1389]
                        tunnel: w1377 -> [w1395]
                        tunnel: [w1393] -> w1376
                        tunnel: [w1392] -> w1375
                        tunnel: [w1391] -> w1374
                        tunnel: [w1390] -> w1373
                        tunnel: [w1389] -> w1372
                        tunnel: w1371 -> [w1388]
                        tunnel: [w1383] -> w1370
                        tunnel: [w1383] -> w1369
                        i -> [w1387]
                        stop <- w1384 stop-if-true
                        n855 = Multiply(x=w1389, y=w1387) -> (x*y=w1396:dbl)
                        n856 = Subtract(x=w1395, y=w1396) -> (x-y=w1394:dbl)
                        n857 = Build Array(w1390, w1394) -> (w1401:dbl[])
                        n858 = Build Array(w1394, w1390) -> (w1400:dbl[])
                        n859 = Greater Or Equal?(x=w1387, y=w1388) -> (x >= y?=w1383:bool)
                        n860 = Select(t=w1401, s=w1391, f=w1400) -> (s? t:f=w1399:dbl[])
                        n861 = local read "Fish"() -> (w1385:bool)
                        n862 = Not(x=w1385) -> (.not. x?=w1386:bool)
                        n863 = call-poly <vilib>:"DAQmx Write.vi"("task/channels in"=w1398, "data"=w1399, "error in"=w1397) -> ("task out"=w1393:refnum<k21>, "error out"=w1392:errorcluster)  [unwired: 10 in, 1 out]
                        n864 = Compound Arithmetic op=OR(w1383, w1386) -> (w1384:bool)
                      }
                    }
                  }
                }
                frame #1 {
                  n865 = case shown="True" w1403 {
                    frame False {
                    }
                    frame True {
                      n866 = Wait (ms)(milliseconds to wait="Wait (ms)") -> ()  [unwired: 1 out]
                    }
                  }
                }
                frame #2 {
                  n867 = case shown="True" w1412 {
                    tunnel: w1419 -> [w1422 w1431]
                    tunnel: w1418 -> [w1421 w1430]
                    tunnel: w1417 -> [_ w1429]
                    tunnel: w1416 -> [_ w1428]
                    tunnel: w1415 -> [_ w1427]
                    tunnel: [w1422 w1426] -> w1414
                    tunnel: [w1421 w1425] -> w1413
                    tunnel: [FALSE w1424] -> w1411
                    tunnel: w1410 -> [_ w1423]
                    frame False {
                    }
                    frame True {
                      n868 = while {
                        tunnel: w1431 -> [w1459]
                        tunnel: w1430 -> [w1458]
                        tunnel: w1429 -> [w1443]
                        tunnel: w1428 -> [w1456]
                        tunnel: w1427 -> [w1455]
                        tunnel: [w1453] -> w1426
                        tunnel: [w1452] -> w1425
                        tunnel: [w1436] -> w1424
                        tunnel: w1423 -> [w1433]
                        i -> [w1444]
                        stop <- w1449 stop-if-true
                        # "If tether formed,\nimmediately change\nto new delta."
                        n869 = local read "Fixed Y"() -> (w1437:dbl)
                        n870 = local read "Fixed X"() -> (w1442:dbl)
                        n871 = local read "Cutoff force (pN)"() -> (w1445:dbl)
                        n872 = Multiply(x=w1456, y=w1444) -> (x*y=w1457:dbl)
                        n873 = local read "Mean force (pN)"() -> (w1446:dbl)
                        n874 = Add(x=w1455, y=w1457) -> (x+y=w1439:dbl)
                        n875 = Select(t=w1437, s=w1443, f=w1442) -> (s? t:f=w1441:dbl)
                        n876 = Greater?(x=w1446, y=w1445) -> (0:w1436:bool)
                        n877 = Add(x=w1441, y="Delta after tether") -> (x+y=w1440:dbl)
                        n878 = Select(t=w1440, s=w1436, f=w1439) -> (s? t:f=w1438:dbl)
                        n879 = local read "Fish Speed (ms)"() -> (w1451:i32)
                        n880 = Build Array(w1433, w1438) -> (w1454:dbl[])
                        n881 = Build Array(w1438, w1433) -> (w1434:dbl[])
                        n882 = Select(t=w1454, s=w1443, f=w1434) -> (s? t:f=w1432:dbl[])
                        n883 = case shown="True" w1436 {
                          tunnel: "Delta after tether" -> [_ _]
                          tunnel: w1432 -> [_ w1461]
                          frame False {
                          }
                          frame True {
                            n884 = Array To Cluster(array=w1461) -> (cluster=w1460:cluster{"[0]":dbl, "[1]":dbl})
                            n885 = local write "Trap position"(w1460) -> ()
                          }
                        }
                        n886 = local read "Fish"() -> (w1448:bool)
                        n887 = Greater Or Equal?(x=w1444, y=w1451) -> (x >= y?=w1450:bool)
                        n888 = Not(x=w1448) -> (.not. x?=w1447:bool)
                        n889 = call-poly <vilib>:"DAQmx Write.vi"("task/channels in"=w1459, "data"=w1432, "error in"=w1458) -> ("task out"=w1453:refnum<k21>, "error out"=w1452:errorcluster)  [unwired: 10 in, 1 out]
                        n890 = Compound Arithmetic op=OR(w1450, w1447, w1436) -> (w1449:bool)
                      }
                    }
                  }
                }
              }
              n891 = Add(x=w1313, y="Min fish\ndelta (V)") -> (x+y=w1320:dbl)
              n892 = Decrement(x="# attempts") -> (x-1=w1329:dbl)
              n893 = Greater Or Equal?(x=w1325, y=w1329) -> (x >= y?=w1328:bool)
              n894 = local read "Mean force (pN)"() -> (w1327:dbl)
              n895 = Greater?(x=w1327, y="Cutoff force (pN)") -> (0:w1322:bool)
              n896 = Compound Arithmetic op=OR(w1307, w1322, w1328) -> (w1321:bool)
              n897 = case shown="True" w1307 {
                frame False {
                }
                frame True {
                  n898 = call <vilib>:"Beep.vi"() -> ()  [unwired: 12 in]
                }
              }
              n899 = node-c288() -> ()  [unwired: 1 in, 1 out]
              "Tether" <- w1307
              "Attempt #" <- w1325
            }
            n900 = node-c288(w1290) -> ()  [unwired: 1 out]
            n901 = flat-sequence {
              tunnel: w1280 -> [w1299]
              tunnel: [w1299] -> w1279
              tunnel: w1278 -> [w1296]
              tunnel: w1277 -> [w1295]
              tunnel: w1276 -> [w1294]
              tunnel: w1279 -> [w1301]
              frame #0 {
                w1298 = T15 1 items=["no dialog", "OK message", "continue or stop message", "OK message + warnings", "continue/stop + warnings"] ("type of dialog (OK msg:1)")
                n902 = call <vilib>:"DAQmx Clear Task.vi"("task in"=w1296, "error in"=w1295) -> ("error out"=w1297:errorcluster)  [unwired: 13 in]
                n903 = Not(x=w1294) -> (.not. x?=w1293:bool)
                n904 = local write "Fish"(w1293) -> ()
                n905 = Wait (ms)(milliseconds to wait=u32 300) -> ()  [unwired: 1 out]
                n906 = call <vilib>:"Simple Error Handler.vi"("type of dialog (OK msg:1)"=w1298, "error in (no error)"=w1297) -> ()  [unwired: 3 in, 5 out]
              }
              frame #1 {
                n907 = And(x=w1301, y="Raster after\n tether?") -> (x .and. y?=w1302:bool)
                n908 = case shown="True" w1302 {
                  selector: w1302 -> [_ w1304]
                  frame False {
                  }
                  frame True {
                    n909 = property on="Raster scan" class="Bool (strict)"("Val(Sgnl)"=w1304) -> ()  [unwired: 2 in, 2 out]
                    n910 = property on="Inject Sample" class="Bool (strict)"("Val(Sgnl)"=FALSE ("Value (Signaling)")) -> ()  [unwired: 2 in, 2 out]
                  }
                }
              }
            }
          }
        }
      }
      event "Load param": Value Change {
        n911 = event-data() -> ()  [unwired: 1 in, 6 out]
        n912 = property on="Scan Parameters" class="Arr (strict)"() -> ("Index Values"=w1474:u32[])  [unwired: 2 in, 2 out]
        n913 = Index Array(array=w1474, index=0) -> (element=w1471:u32)
        n914 = Index Array(array="Scan Parameters", index=w1471) -> (element=w1470:T18)
        n915 = Unbundle(w1470) -> ("# scans 2"=w1469:i32)  [unwired: 4 out]
        n916 = local write "Load param"(FALSE ("Load param")) -> ()
        n917 = property on="# scans" class="DigNum (strict)"("Val(Sgnl)"=w1469) -> ()  [unwired: 2 in, 2 out]
      }
      event "Step size (nm)", "Scan speed (nm/s)", "# scans", "Pulling direction", "Scan range (nm)": Value Change {
        n918 = event-data() -> ()  [unwired: 1 in, 6 out]
        n919 = local read "Pulling direction"() -> (w1505:bool)
        n920 = Reciprocal(x="Scan speed (nm/s)") -> (1/x=w1497:dbl)
        n921 = local read "Conv Y (nm/V)"() -> (w1503:dbl)
        n922 = local read "Conv X (nm/V)"() -> (w1504:dbl)
        n923 = Multiply(x="Step size (nm)", y=w1497) -> (x*y=w1495:dbl)
        n924 = Divide(x="Scan range (nm)", y="Step size (nm)") -> (x/y=w1502:dbl)
        n925 = Absolute Value(x=w1502) -> (abs(x)=w1501:dbl)
        n926 = Multiply(x=w1495, y=1000.0) -> (x*y=w1482:dbl)
        n927 = Select(t=w1503, s=w1505, f=w1504) -> (s? t:f=w1493:dbl)
        n928 = Multiply(x="# scans", y=2) -> (x*y=w1481:i32)
        n929 = To Unsigned Quad Integer(1:w1501) -> (0:w1491:u64)
        "Scan steps (mirror)" <- w1491
        n930 = Divide(x="Scan range (nm)", y=w1493) -> (x/y=→"Scan range (V)":dbl)
        n931 = Multiply(x=w1491, y=w1482) -> (x*y=w1490:dbl)
        n932 = Divide(x="Step size (nm)", y=w1493) -> (x/y=→"Scan increment (V)":dbl)
        n933 = Round Toward +Infinity(x=w1482) -> (ceil(x): smallest int >= x=w1479:dbl)
        "Time per step (ms)" <- w1479
        n934 = local read "Data update period (s/set)"() -> (w1485:dbl)
        n935 = Multiply(x=w1481, y=w1490) -> (x*y=w1488:dbl)
        n936 = Divide(x=w1488, y=1000.0) -> (x/y=w1486:dbl)
        "Total raster time (s)" <- w1486
        n937 = local read "Data update period (s/set)"() -> (w1477:dbl)
        n938 = Divide(x=w1486, y=w1485) -> (x/y=w1484:dbl)
        n939 = Round Toward -Infinity(1:w1484) -> (0:→"N sets to be saved":dbl)
        n940 = Multiply(x=w1477, y=1000.0) -> (x*y=w1475:dbl)
        n941 = Less?(x=w1479, y=w1475) -> (x < y?=w1478:bool)
        n942 = case shown="True" w1478 {
          selector: w1478 -> [_ w1506]
          frame False {
          }
          frame True {
            n943 = call "Display Message to User"("Enable"=w1506) -> ()  [unwired: 9 in, 2 out]
          }
        }
      }
      event "Averaging Number": Value Change {
        n944 = event-data() -> ()  [unwired: 1 in, 6 out]
        n945 = local read "# Samples/channel (in)"() -> (w1510:i32)
        n946 = local read "Averaging Number"() -> (w1508:i32)
        n947 = Quotient & Remainder(x=w1510, y=w1508) -> (floor(x/y)=w1509:i32)  [unwired: 1 out]
        n948 = Multiply(x=w1509, y=w1508) -> (x*y=w1507:i32)
        n949 = local write "# Samples/channel (in)"(w1507) -> ()
      }
    }
    n950 = node-c288() -> ()  [unwired: 1 in, 1 out]
  }
  n951 = call <vilib>:"Simple Error Handler.vi"("error in (no error)"=w104) -> ()  [unwired: 4 in, 5 out]
  n952 = disable-structure shown="Enabled" {
    frame Disabled {
      n953 = node-c288(2 ("Processor")) -> (w1516:T12)  [unwired: 3 in]
      n954 = timed-loop "Pump Control" {
        timing: w1516 -> [_]
        timing-out: [_] -> w1515
        tunnel: refnum<visa-resource-name> "COM6" ("VISA resource name") -> [w1518]
        stop <- w1517 stop-if-true
        n955 = node-c288() -> ()  [unwired: 1 in, 1 out]
        n956 = event shown="[4] \"Inject Pump 1\": Value Change" {
          selector: _ -> [_ _ _ _ _ _ _ _ _]
          dyn-events: _ -> [_ _ _ _ _ _ _ _ _]
          timeout: _ -> [_ _ _ _ _ _ _ _ _]
          tunnel: w1518 -> [w1526 w1622 _ w1698 w1826 w1969 w2014 w2072 w2131]
          tunnel: [_ _ w1697 _ _ _ _ _ _] -> w1517
          event "Flush Pump 1": Value Change {
            w1527 = "\r"
            n957 = event-data() -> ()  [unwired: 1 in, 5 out]
            n958 = call-poly "VISA Configure Serial Port"("VISA resource name"=w1526) -> ("VISA resource name out"=w1540:refnum<visa-resource-name>, "error out"=w1541:errorcluster)  [unwired: 13 in]
            n959 = local read "Write Wait"() -> (w1519:i32)
            n960 = Concatenate Strings("enter pump1", w1527) -> (w1528:string)
            n961 = flat-sequence {
              tunnel: w1541 -> [w1560]
              tunnel: w1540 -> [w1562]
              tunnel: [w1561] -> w1557
              tunnel: [w1559] -> w1556
              tunnel: w1528 -> [w1558]
              tunnel: w1557 -> [w1565]
              tunnel: [w1565] -> w1555
              tunnel: w1556 -> [w1564]
              tunnel: [w1564] -> w1554
              tunnel: w1519 -> [w1563]
              tunnel: [w1570] -> w1553
              tunnel: w1533 -> [w1569]
              tunnel: [w1566] -> w1552
              tunnel: w1555 -> [w1568]
              tunnel: w1554 -> [w1567]
              tunnel: w1553 -> [w1573]
              tunnel: [w1573] -> w1551
              tunnel: [w1572] -> w1550
              tunnel: w1552 -> [w1572]
              tunnel: w1519 -> [w1571]
              tunnel: w1551 -> [w1578]
              tunnel: [w1577] -> w1549
              tunnel: w1536 -> [w1576]
              tunnel: w1550 -> [w1575]
              tunnel: [w1574] -> w1548
              tunnel: w1549 -> [w1581]
              tunnel: [w1581] -> w1547
              tunnel: [w1580] -> w1546
              tunnel: w1548 -> [w1580]
              tunnel: w1519 -> [w1579]
              tunnel: w1547 -> [w1586]
              tunnel: [w1585] -> w1545
              tunnel: w1539 -> [w1584]
              tunnel: w1546 -> [w1583]
              tunnel: [w1582] -> w1544
              tunnel: [w1589] -> w1543
              tunnel: w1545 -> [w1589]
              tunnel: [w1588] -> w1542
              tunnel: w1544 -> [w1588]
              tunnel: w1519 -> [w1587]
              tunnel: w1543 -> [w1594]
              tunnel: w1542 -> [w1591]
              tunnel: [w1593] -> w1522
              tunnel: [w1592] -> w1520
              tunnel: [w1599] -> w1523
              tunnel: w1522 -> [w1599]
              tunnel: [w1598] -> w1521
              tunnel: w1520 -> [w1598]
              tunnel: w1519 -> [w1597]
              tunnel: w1523 -> [w1601]
              tunnel: w1521 -> [w1600]
              frame #0 {
                n962 = VISA Write(VISA resource name=w1562, write buffer=w1558, error in (no error)=w1560) -> (VISA resource name out=w1561:refnum<visa-resource-name>, error out=w1559:errorcluster)  [unwired: 1 out]
              }
              frame #1 {
                n963 = Wait (ms)(milliseconds to wait=w1563) -> ()  [unwired: 1 out]
              }
              frame #2 {
                n964 = VISA Write(VISA resource name=w1568, write buffer=w1569, error in (no error)=w1567) -> (VISA resource name out=w1570:refnum<visa-resource-name>, error out=w1566:errorcluster)  [unwired: 1 out]
              }
              frame #3 {
                n965 = Wait (ms)(milliseconds to wait=w1571) -> ()  [unwired: 1 out]
              }
              frame #4 {
                n966 = VISA Write(VISA resource name=w1578, write buffer=w1576, error in (no error)=w1575) -> (VISA resource name out=w1577:refnum<visa-resource-name>, error out=w1574:errorcluster)  [unwired: 1 out]
              }
              frame #5 {
                n967 = Wait (ms)(milliseconds to wait=w1579) -> ()  [unwired: 1 out]
              }
              frame #6 {
                n968 = VISA Write(VISA resource name=w1586, write buffer=w1584, error in (no error)=w1583) -> (VISA resource name out=w1585:refnum<visa-resource-name>, error out=w1582:errorcluster)  [unwired: 1 out]
              }
              frame #7 {
                n969 = Wait (ms)(milliseconds to wait=w1587) -> ()  [unwired: 1 out]
              }
              frame #8 {
                n970 = Concatenate Strings("start ", "\r") -> (w1590:string)
                n971 = VISA Write(VISA resource name=w1594, write buffer=w1590, error in (no error)=w1591) -> (VISA resource name out=w1593:refnum<visa-resource-name>, error out=w1592:errorcluster)  [unwired: 1 out]
              }
              frame #9 {
                n972 = Wait (ms)(milliseconds to wait=w1597) -> ()  [unwired: 1 out]
              }
              frame #10 {
                n973 = local write "Flush Pump 1"(FALSE ("Flush Pump 1")) -> ()
                n974 = Concatenate Strings("enter main ", "\r") -> (w1605:string)
                n975 = VISA Write(VISA resource name=w1601, write buffer=w1605, error in (no error)=w1600) -> (VISA resource name out=w1604:refnum<visa-resource-name>, error out=w1603:errorcluster)  [unwired: 1 out]
                n976 = VISA Close(VISA resource name=w1604, error in (no error)=w1603) -> ()  [unwired: 1 out]
              }
            }
            n977 = Concatenate Strings("set units 4 ", w1527) -> (w1533:string)
            n978 = Multiply(x="Flush\nRate (ul/min)", y=60) -> (x*y=w1531:dbl)
            n979 = Number To Decimal String(number=w1531) -> (decimal integer string=w1534:string)  [unwired: 1 in]
            n980 = Concatenate Strings("set rate ", w1534, w1527) -> (w1536:string)
            n981 = Number To Decimal String(number="Flush\nVolume (ul)") -> (decimal integer string=w1538:string)  [unwired: 1 in]
            n982 = Concatenate Strings("set volume ", w1538, w1527) -> (w1539:string)
          }
          event "Flush Pump 2": Value Change {
            w1613 = "\r"
            n983 = event-data() -> ()  [unwired: 1 in, 5 out]
            n984 = call-poly "VISA Configure Serial Port"("VISA resource name"=w1622) -> ("VISA resource name out"=w1633:refnum<visa-resource-name>, "error out"=w1634:errorcluster)  [unwired: 13 in]
            n985 = local read "Write Wait"() -> (w1608:i32)
            n986 = Concatenate Strings("enter pump2", w1613) -> (w1614:string)
            n987 = flat-sequence {
              tunnel: w1634 -> [w1649]
              tunnel: w1633 -> [w1651]
              tunnel: [w1650] -> w1619
              tunnel: [w1648] -> w1617
              tunnel: w1614 -> [w1647]
              tunnel: w1619 -> [w1654]
              tunnel: [w1654] -> w1618
              tunnel: w1617 -> [w1653]
              tunnel: [w1653] -> w1616
              tunnel: w1608 -> [w1652]
              tunnel: [w1659] -> w1646
              tunnel: w1626 -> [w1658]
              tunnel: [w1655] -> w1645
              tunnel: w1618 -> [w1657]
              tunnel: w1616 -> [w1656]
              tunnel: w1646 -> [w1662]
              tunnel: [w1662] -> w1644
              tunnel: [w1661] -> w1643
              tunnel: w1645 -> [w1661]
              tunnel: w1608 -> [w1660]
              tunnel: w1644 -> [w1667]
              tunnel: [w1666] -> w1642
              tunnel: w1629 -> [w1665]
              tunnel: w1643 -> [w1664]
              tunnel: [w1663] -> w1641
              tunnel: w1642 -> [w1670]
              tunnel: [w1670] -> w1640
              tunnel: [w1669] -> w1639
              tunnel: w1641 -> [w1669]
              tunnel: w1608 -> [w1668]
              tunnel: w1640 -> [w1675]
              tunnel: [w1674] -> w1638
              tunnel: w1632 -> [w1673]
              tunnel: w1639 -> [w1672]
              tunnel: [w1671] -> w1637
              tunnel: [w1678] -> w1636
              tunnel: w1638 -> [w1678]
              tunnel: [w1677] -> w1635
              tunnel: w1637 -> [w1677]
              tunnel: w1608 -> [w1676]
              tunnel: w1636 -> [w1685]
              tunnel: w1635 -> [w1684]
              tunnel: [w1680] -> w1612
              tunnel: [w1679] -> w1610
              tunnel: w1612 -> [w1688]
              tunnel: [w1688] -> w1611
              tunnel: w1610 -> [w1687]
              tunnel: [w1687] -> w1609
              tunnel: w1608 -> [w1686]
              tunnel: w1611 -> [w1692]
              tunnel: w1609 -> [w1691]
              frame #0 {
                n988 = VISA Write(VISA resource name=w1651, write buffer=w1647, error in (no error)=w1649) -> (VISA resource name out=w1650:refnum<visa-resource-name>, error out=w1648:errorcluster)  [unwired: 1 out]
              }
              frame #1 {
                n989 = Wait (ms)(milliseconds to wait=w1652) -> ()  [unwired: 1 out]
              }
              frame #2 {
                n990 = VISA Write(VISA resource name=w1657, write buffer=w1658, error in (no error)=w1656) -> (VISA resource name out=w1659:refnum<visa-resource-name>, error out=w1655:errorcluster)  [unwired: 1 out]
              }
              frame #3 {
                n991 = Wait (ms)(milliseconds to wait=w1660) -> ()  [unwired: 1 out]
              }
              frame #4 {
                n992 = VISA Write(VISA resource name=w1667, write buffer=w1665, error in (no error)=w1664) -> (VISA resource name out=w1666:refnum<visa-resource-name>, error out=w1663:errorcluster)  [unwired: 1 out]
              }
              frame #5 {
                n993 = Wait (ms)(milliseconds to wait=w1668) -> ()  [unwired: 1 out]
              }
              frame #6 {
                n994 = VISA Write(VISA resource name=w1675, write buffer=w1673, error in (no error)=w1672) -> (VISA resource name out=w1674:refnum<visa-resource-name>, error out=w1671:errorcluster)  [unwired: 1 out]
              }
              frame #7 {
                n995 = Wait (ms)(milliseconds to wait=w1676) -> ()  [unwired: 1 out]
              }
              frame #8 {
                n996 = Concatenate Strings("start ", "\r") -> (w1683:string)
                n997 = VISA Write(VISA resource name=w1685, write buffer=w1683, error in (no error)=w1684) -> (VISA resource name out=w1680:refnum<visa-resource-name>, error out=w1679:errorcluster)  [unwired: 1 out]
              }
              frame #9 {
                n998 = Wait (ms)(milliseconds to wait=w1686) -> ()  [unwired: 1 out]
              }
              frame #10 {
                n999 = local write "Flush Pump 2"(FALSE ("Flush Pump 1")) -> ()
                n1000 = Concatenate Strings("enter main ", "\r") -> (w1693:string)
                n1001 = VISA Write(VISA resource name=w1692, write buffer=w1693, error in (no error)=w1691) -> (VISA resource name out=w1690:refnum<visa-resource-name>, error out=w1689:errorcluster)  [unwired: 1 out]
                n1002 = VISA Close(VISA resource name=w1690, error in (no error)=w1689) -> ()  [unwired: 1 out]
              }
            }
            n1003 = Concatenate Strings("set units 4 ", w1613) -> (w1626:string)
            n1004 = Multiply(x="Flush \nRate (ul/min)  2", y=60) -> (x*y=w1624:dbl)
            n1005 = Number To Decimal String(number=w1624) -> (decimal integer string=w1627:string)  [unwired: 1 in]
            n1006 = Concatenate Strings("set rate ", w1627, w1613) -> (w1629:string)
            n1007 = Number To Decimal String(number="Flush\nVolume (ul)  2") -> (decimal integer string=w1631:string)  [unwired: 1 in]
            n1008 = Concatenate Strings("set volume ", w1631, w1613) -> (w1632:string)
          }
          event "Stop": Value Change {
            n1009 = event-data() -> ()  [unwired: 1 in, 5 out]
            n1010 = local read "Stop"() -> (w1697:bool)
          }
          event "Inject Pump 2": Value Change {
            n1011 = event-data() -> ()  [unwired: 1 in, 5 out]
            n1012 = case shown="True" "Inject Pump 2" {
              tunnel: w1698 -> [w1701 w1743]
              frame False {
                n1013 = local read "Write Wait"() -> (w1700:i32)
                n1014 = call-poly "VISA Configure Serial Port"("VISA resource name"=w1701) -> ("VISA resource name out"=w1705:refnum<visa-resource-name>, "error out"=w1706:errorcluster)  [unwired: 13 in]
                n1015 = Concatenate Strings("enter pump2", "\r") -> (w1703:string)
                n1016 = flat-sequence {
                  tunnel: w1706 -> [w1717]
                  tunnel: w1705 -> [w1719]
                  tunnel: [w1718] -> w1714
                  tunnel: [w1716] -> w1713
                  tunnel: w1703 -> [w1715]
                  tunnel: w1714 -> [w1722]
                  tunnel: w1713 -> [w1721]
                  tunnel: [w1722] -> w1712
                  tunnel: [w1721] -> w1711
                  tunnel: w1700 -> [w1720]
                  tunnel: [w1726] -> w1710
                  tunnel: [w1725] -> w1709
                  tunnel: w1712 -> [w1724]
                  tunnel: w1711 -> [w1723]
                  tunnel: w1710 -> [w1732]
                  tunnel: [w1732] -> w1708
                  tunnel: w1709 -> [w1731]
                  tunnel: [w1731] -> w1707
                  tunnel: w1700 -> [w1730]
                  tunnel: w1708 -> [w1736]
                  tunnel: w1707 -> [w1735]
                  frame #0 {
                    n1017 = VISA Write(VISA resource name=w1719, write buffer=w1715, error in (no error)=w1717) -> (VISA resource name out=w1718:refnum<visa-resource-name>, error out=w1716:errorcluster)  [unwired: 1 out]
                  }
                  frame #1 {
                    n1018 = Wait (ms)(milliseconds to wait=w1720) -> ()  [unwired: 1 out]
                  }
                  frame #2 {
                    n1019 = Concatenate Strings("stop ", "\r") -> (w1729:string)
                    n1020 = VISA Write(VISA resource name=w1724, write buffer=w1729, error in (no error)=w1723) -> (VISA resource name out=w1726:refnum<visa-resource-name>, error out=w1725:errorcluster)  [unwired: 1 out]
                  }
                  frame #3 {
                    n1021 = Wait (ms)(milliseconds to wait=w1730) -> ()  [unwired: 1 out]
                  }
                  frame #4 {
                    n1022 = Concatenate Strings("enter main ", "\r") -> (w1737:string)
                    n1023 = VISA Write(VISA resource name=w1736, write buffer=w1737, error in (no error)=w1735) -> (VISA resource name out=w1734:refnum<visa-resource-name>, error out=w1733:errorcluster)  [unwired: 1 out]
                    n1024 = VISA Close(VISA resource name=w1734, error in (no error)=w1733) -> ()  [unwired: 1 out]
                  }
                }
              }
              frame True {
                w1756 = "\r"
                n1025 = call-poly "VISA Configure Serial Port"("VISA resource name"=w1743) -> ("VISA resource name out"=w1745:refnum<visa-resource-name>, "error out"=w1744:errorcluster)  [unwired: 13 in]
                n1026 = local read "Write Wait"() -> (w1740:i32)
                n1027 = Concatenate Strings("enter pump2", w1756) -> (w1755:string)
                n1028 = flat-sequence {
                  tunnel: w1744 -> [w1779]
                  tunnel: w1745 -> [w1781]
                  tunnel: [w1780] -> w1776
                  tunnel: [w1778] -> w1775
                  tunnel: w1755 -> [w1777]
                  tunnel: w1776 -> [w1784]
                  tunnel: [w1784] -> w1774
                  tunnel: w1775 -> [w1783]
                  tunnel: [w1783] -> w1773
                  tunnel: w1740 -> [w1782]
                  tunnel: [w1789] -> w1772
                  tunnel: w1752 -> [w1788]
                  tunnel: [w1785] -> w1771
                  tunnel: w1774 -> [w1787]
                  tunnel: w1773 -> [w1786]
                  tunnel: w1772 -> [w1792]
                  tunnel: [w1792] -> w1770
                  tunnel: [w1791] -> w1769
                  tunnel: w1771 -> [w1791]
                  tunnel: w1740 -> [w1790]
                  tunnel: w1770 -> [w1797]
                  tunnel: [w1796] -> w1768
                  tunnel: w1749 -> [w1795]
                  tunnel: w1769 -> [w1794]
                  tunnel: [w1793] -> w1767
                  tunnel: w1768 -> [w1800]
                  tunnel: [w1800] -> w1766
                  tunnel: [w1799] -> w1765
                  tunnel: w1767 -> [w1799]
                  tunnel: w1740 -> [w1798]
                  tunnel: w1766 -> [w1805]
                  tunnel: [w1804] -> w1764
                  tunnel: w1746 -> [w1803]
                  tunnel: w1765 -> [w1802]
                  tunnel: [w1801] -> w1763
                  tunnel: [w1808] -> w1762
                  tunnel: w1764 -> [w1808]
                  tunnel: [w1807] -> w1761
                  tunnel: w1763 -> [w1807]
                  tunnel: w1740 -> [w1806]
                  tunnel: w1762 -> [w1815]
                  tunnel: w1761 -> [w1814]
                  tunnel: [w1810] -> w1760
                  tunnel: [w1809] -> w1759
                  tunnel: w1760 -> [w1818]
                  tunnel: [w1818] -> w1758
                  tunnel: w1759 -> [w1817]
                  tunnel: [w1817] -> w1757
                  tunnel: w1740 -> [w1816]
                  tunnel: w1758 -> [w1822]
                  tunnel: w1757 -> [w1821]
                  frame #0 {
                    n1029 = VISA Write(VISA resource name=w1781, write buffer=w1777, error in (no error)=w1779) -> (VISA resource name out=w1780:refnum<visa-resource-name>, error out=w1778:errorcluster)  [unwired: 1 out]
                  }
                  frame #1 {
                    n1030 = Wait (ms)(milliseconds to wait=w1782) -> ()  [unwired: 1 out]
                  }
                  frame #2 {
                    n1031 = VISA Write(VISA resource name=w1787, write buffer=w1788, error in (no error)=w1786) -> (VISA resource name out=w1789:refnum<visa-resource-name>, error out=w1785:errorcluster)  [unwired: 1 out]
                  }
                  frame #3 {
                    n1032 = Wait (ms)(milliseconds to wait=w1790) -> ()  [unwired: 1 out]
                  }
                  frame #4 {
                    n1033 = VISA Write(VISA resource name=w1797, write buffer=w1795, error in (no error)=w1794) -> (VISA resource name out=w1796:refnum<visa-resource-name>, error out=w1793:errorcluster)  [unwired: 1 out]
                  }
                  frame #5 {
                    n1034 = Wait (ms)(milliseconds to wait=w1798) -> ()  [unwired: 1 out]
                  }
                  frame #6 {
                    n1035 = VISA Write(VISA resource name=w1805, write buffer=w1803, error in (no error)=w1802) -> (VISA resource name out=w1804:refnum<visa-resource-name>, error out=w1801:errorcluster)  [unwired: 1 out]
                  }
                  frame #7 {
                    n1036 = Wait (ms)(milliseconds to wait=w1806) -> ()  [unwired: 1 out]
                  }
                  frame #8 {
                    n1037 = Concatenate Strings("start ", "\r") -> (w1813:string)
                    n1038 = VISA Write(VISA resource name=w1815, write buffer=w1813, error in (no error)=w1814) -> (VISA resource name out=w1810:refnum<visa-resource-name>, error out=w1809:errorcluster)  [unwired: 1 out]
                  }
                  frame #9 {
                    n1039 = Wait (ms)(milliseconds to wait=w1816) -> ()  [unwired: 1 out]
                  }
                  frame #10 {
                    n1040 = Concatenate Strings("enter main ", "\r") -> (w1823:string)
                    n1041 = VISA Write(VISA resource name=w1822, write buffer=w1823, error in (no error)=w1821) -> (VISA resource name out=w1820:refnum<visa-resource-name>, error out=w1819:errorcluster)  [unwired: 1 out]
                    n1042 = VISA Close(VISA resource name=w1820, error in (no error)=w1819) -> ()  [unwired: 1 out]
                  }
                }
                n1043 = local read "Normal \nRate (ul/hr)  2"() -> (w1741:dbl)
                n1044 = Concatenate Strings("set units 4 ", w1756) -> (w1752:string)
                n1045 = local read "Normal \nVolume (ul) 2"() -> (w1742:dbl)
                n1046 = Number To Decimal String(number=w1741) -> (decimal integer string=w1751:string)  [unwired: 1 in]
                n1047 = Concatenate Strings("set rate ", w1751, w1756) -> (w1749:string)
                n1048 = Number To Decimal String(number=w1742) -> (decimal integer string=w1747:string)  [unwired: 1 in]
                n1049 = Concatenate Strings("set volume ", w1747, w1756) -> (w1746:string)
              }
            }
          }
          event "Inject Pump 1": Value Change {
            n1050 = event-data() -> ()  [unwired: 1 in, 5 out]
            n1051 = case shown="True" "Inject Pump 1" {
              tunnel: w1826 -> [w1829 w1871]
              frame False {
                n1052 = local read "Write Wait"() -> (w1828:i32)
                n1053 = call-poly "VISA Configure Serial Port"("VISA resource name"=w1829) -> ("VISA resource name out"=w1833:refnum<visa-resource-name>, "error out"=w1834:errorcluster)  [unwired: 13 in]
                n1054 = Concatenate Strings("enter pump1", "\r") -> (w1831:string)
                n1055 = flat-sequence {
                  tunnel: w1834 -> [w1845]
                  tunnel: w1833 -> [w1847]
                  tunnel: [w1846] -> w1842
                  tunnel: [w1844] -> w1841
                  tunnel: w1831 -> [w1843]
                  tunnel: w1842 -> [w1850]
                  tunnel: w1841 -> [w1849]
                  tunnel: [w1850] -> w1840
                  tunnel: [w1849] -> w1839
                  tunnel: w1828 -> [w1848]
                  tunnel: [w1854] -> w1838
                  tunnel: [w1853] -> w1837
                  tunnel: w1840 -> [w1852]
                  tunnel: w1839 -> [w1851]
                  tunnel: w1838 -> [w1860]
                  tunnel: [w1860] -> w1836
                  tunnel: w1837 -> [w1859]
                  tunnel: [w1859] -> w1835
                  tunnel: w1828 -> [w1858]
                  tunnel: w1836 -> [w1864]
                  tunnel: w1835 -> [w1863]
                  frame #0 {
                    n1056 = VISA Write(VISA resource name=w1847, write buffer=w1843, error in (no error)=w1845) -> (VISA resource name out=w1846:refnum<visa-resource-name>, error out=w1844:errorcluster)  [unwired: 1 out]
                  }
                  frame #1 {
                    n1057 = Wait (ms)(milliseconds to wait=w1848) -> ()  [unwired: 1 out]
                  }
                  frame #2 {
                    n1058 = Concatenate Strings("stop ", "\r") -> (w1857:string)
                    n1059 = VISA Write(VISA resource name=w1852, write buffer=w1857, error in (no error)=w1851) -> (VISA resource name out=w1854:refnum<visa-resource-name>, error out=w1853:errorcluster)  [unwired: 1 out]
                  }
                  frame #3 {
                    n1060 = Wait (ms)(milliseconds to wait=w1858) -> ()  [unwired: 1 out]
                  }
                  frame #4 {
                    n1061 = Concatenate Strings("enter main ", "\r") -> (w1865:string)
                    n1062 = VISA Write(VISA resource name=w1864, write buffer=w1865, error in (no error)=w1863) -> (VISA resource name out=w1862:refnum<visa-resource-name>, error out=w1861:errorcluster)  [unwired: 1 out]
                    n1063 = VISA Close(VISA resource name=w1862, error in (no error)=w1861) -> ()  [unwired: 1 out]
                  }
                }
              }
              frame True {
                w1884 = "\r"
                n1064 = call-poly "VISA Configure Serial Port"("VISA resource name"=w1871) -> ("VISA resource name out"=w1873:refnum<visa-resource-name>, "error out"=w1872:errorcluster)  [unwired: 13 in]
                n1065 = local read "Write Wait"() -> (w1868:i32)
                n1066 = flat-sequence {
                  tunnel: w1872 -> [w1907]
                  tunnel: w1873 -> [w1909]
                  tunnel: [w1908] -> w1904
                  tunnel: [w1906] -> w1903
                  tunnel: w1883 -> [w1905]
                  tunnel: w1904 -> [w1912]
                  tunnel: [w1912] -> w1902
                  tunnel: w1903 -> [w1911]
                  tunnel: [w1911] -> w1901
                  tunnel: w1868 -> [w1910]
                  tunnel: [w1917] -> w1900
                  tunnel: w1880 -> [w1916]
                  tunnel: [w1913] -> w1899
                  tunnel: w1902 -> [w1915]
                  tunnel: w1901 -> [w1914]
                  tunnel: w1900 -> [w1920]
                  tunnel: [w1920] -> w1898
                  tunnel: [w1919] -> w1897
                  tunnel: w1899 -> [w1919]
                  tunnel: w1868 -> [w1918]
                  tunnel: w1898 -> [w1925]
                  tunnel: [w1924] -> w1896
                  tunnel: w1877 -> [w1923]
                  tunnel: w1897 -> [w1922]
                  tunnel: [w1921] -> w1895
                  tunnel: w1896 -> [w1928]
                  tunnel: [w1928] -> w1894
                  tunnel: [w1927] -> w1893
                  tunnel: w1895 -> [w1927]
                  tunnel: w1868 -> [w1926]
                  tunnel: w1894 -> [w1933]
                  tunnel: [w1932] -> w1892
                  tunnel: w1874 -> [w1931]
                  tunnel: w1893 -> [w1930]
                  tunnel: [w1929] -> w1891
                  tunnel: [w1936] -> w1890
                  tunnel: w1892 -> [w1936]
                  tunnel: [w1935] -> w1889
                  tunnel: w1891 -> [w1935]
                  tunnel: w1868 -> [w1934]
                  tunnel: w1890 -> [w1943]
                  tunnel: w1889 -> [w1942]
                  tunnel: [w1938] -> w1888
                  tunnel: [w1937] -> w1887
                  tunnel: w1888 -> [w1946]
                  tunnel: [w1946] -> w1886
                  tunnel: w1887 -> [w1945]
                  tunnel: [w1945] -> w1885
                  tunnel: w1868 -> [w1944]
                  tunnel: w1886 -> [w1950]
                  tunnel: w1885 -> [w1949]
                  frame #0 {
                    n1067 = VISA Write(VISA resource name=w1909, write buffer=w1905, error in (no error)=w1907) -> (VISA resource name out=w1908:refnum<visa-resource-name>, error out=w1906:errorcluster)  [unwired: 1 out]
                  }
                  frame #1 {
                    n1068 = Wait (ms)(milliseconds to wait=w1910) -> ()  [unwired: 1 out]
                  }
                  frame #2 {
                    n1069 = VISA Write(VISA resource name=w1915, write buffer=w1916, error in (no error)=w1914) -> (VISA resource name out=w1917:refnum<visa-resource-name>, error out=w1913:errorcluster)  [unwired: 1 out]
                  }
                  frame #3 {
                    n1070 = Wait (ms)(milliseconds to wait=w1918) -> ()  [unwired: 1 out]
                  }
                  frame #4 {
                    n1071 = VISA Write(VISA resource name=w1925, write buffer=w1923, error in (no error)=w1922) -> (VISA resource name out=w1924:refnum<visa-resource-name>, error out=w1921:errorcluster)  [unwired: 1 out]
                  }
                  frame #5 {
                    n1072 = Wait (ms)(milliseconds to wait=w1926) -> ()  [unwired: 1 out]
                  }
                  frame #6 {
                    n1073 = VISA Write(VISA resource name=w1933, write buffer=w1931, error in (no error)=w1930) -> (VISA resource name out=w1932:refnum<visa-resource-name>, error out=w1929:errorcluster)  [unwired: 1 out]
                  }
                  frame #7 {
                    n1074 = Wait (ms)(milliseconds to wait=w1934) -> ()  [unwired: 1 out]
                  }
                  frame #8 {
                    n1075 = Concatenate Strings("start ", "\r") -> (w1941:string)
                    n1076 = VISA Write(VISA resource name=w1943, write buffer=w1941, error in (no error)=w1942) -> (VISA resource name out=w1938:refnum<visa-resource-name>, error out=w1937:errorcluster)  [unwired: 1 out]
                  }
                  frame #9 {
                    n1077 = Wait (ms)(milliseconds to wait=w1944) -> ()  [unwired: 1 out]
                  }
                  frame #10 {
                    n1078 = Concatenate Strings("enter main ", "\r") -> (w1951:string)
                    n1079 = VISA Write(VISA resource name=w1950, write buffer=w1951, error in (no error)=w1949) -> (VISA resource name out=w1948:refnum<visa-resource-name>, error out=w1947:errorcluster)  [unwired: 1 out]
                    n1080 = VISA Close(VISA resource name=w1948, error in (no error)=w1947) -> ()  [unwired: 1 out]
                  }
                }
                n1081 = Concatenate Strings("enter pump1", w1884) -> (w1883:string)
                n1082 = local read "Normal \nRate (ul/hr)"() -> (w1869:dbl)
                n1083 = Concatenate Strings("set units 4 ", w1884) -> (w1880:string)
                n1084 = local read "Normal \nVolume (ul)"() -> (w1870:dbl)
                n1085 = Number To Decimal String(number=w1869) -> (decimal integer string=w1879:string)  [unwired: 1 in]
                n1086 = Concatenate Strings("set rate ", w1879, w1884) -> (w1877:string)
                n1087 = Number To Decimal String(number=w1870) -> (decimal integer string=w1875:string)  [unwired: 1 in]
                n1088 = Concatenate Strings("set volume ", w1875, w1884) -> (w1874:string)
              }
            }
          }
          event "Normal \nVolume (ul)": Value Change {
            n1089 = event-data() -> ()  [unwired: 1 in, 5 out]
            n1090 = call-poly "VISA Configure Serial Port"("VISA resource name"=w1969) -> ("VISA resource name out"=w1971:refnum<visa-resource-name>, "error out"=w1970:errorcluster)  [unwired: 13 in]
            n1091 = local read "Write Wait"() -> (w1954:i32)
            n1092 = Concatenate Strings("enter pump1", "\r") -> (w1973:string)
            n1093 = flat-sequence {
              tunnel: w1970 -> [w1983]
              tunnel: w1971 -> [w1985]
              tunnel: [w1984] -> w1963
              tunnel: [w1982] -> w1962
              tunnel: w1973 -> [w1981]
              tunnel: w1963 -> [w1988]
              tunnel: [w1988] -> w1961
              tunnel: w1962 -> [w1987]
              tunnel: [w1987] -> w1959
              tunnel: w1954 -> [w1986]
              tunnel: w1961 -> [w1992]
              tunnel: [w1993] -> w1960
              tunnel: w1959 -> [w1991]
              tunnel: [w1990] -> w1958
              tunnel: w1955 -> [w1989]
              tunnel: w1960 -> [w1996]
              tunnel: w1958 -> [w1995]
              tunnel: [w1996] -> w1980
              tunnel: [w1995] -> w1979
              tunnel: w1954 -> [w1994]
              tunnel: [w2001] -> w1978
              tunnel: [w2000] -> w1977
              tunnel: w1980 -> [w1999]
              tunnel: w1979 -> [w1998]
              tunnel: w1964 -> [w1997]
              tunnel: w1978 -> [w2004]
              tunnel: [w2004] -> w1976
              tunnel: w1977 -> [w2003]
              tunnel: [w2003] -> w1975
              tunnel: w1954 -> [w2002]
              tunnel: w1976 -> [w2008]
              tunnel: w1975 -> [w2007]
              frame #0 {
                n1094 = VISA Write(VISA resource name=w1985, write buffer=w1981, error in (no error)=w1983) -> (VISA resource name out=w1984:refnum<visa-resource-name>, error out=w1982:errorcluster)  [unwired: 1 out]
              }
              frame #1 {
                n1095 = Wait (ms)(milliseconds to wait=w1986) -> ()  [unwired: 1 out]
              }
              frame #2 {
                n1096 = VISA Write(VISA resource name=w1992, write buffer=w1989, error in (no error)=w1991) -> (VISA resource name out=w1993:refnum<visa-resource-name>, error out=w1990:errorcluster)  [unwired: 1 out]
              }
              frame #3 {
                n1097 = Wait (ms)(milliseconds to wait=w1994) -> ()  [unwired: 1 out]
              }
              frame #4 {
                n1098 = VISA Write(VISA resource name=w1999, write buffer=w1997, error in (no error)=w1998) -> (VISA resource name out=w2001:refnum<visa-resource-name>, error out=w2000:errorcluster)  [unwired: 1 out]
              }
              frame #5 {
                n1099 = Wait (ms)(milliseconds to wait=w2002) -> ()  [unwired: 1 out]
              }
              frame #6 {
                n1100 = Concatenate Strings("enter main ", "\r") -> (w2009:string)
                n1101 = VISA Write(VISA resource name=w2008, write buffer=w2009, error in (no error)=w2007) -> (VISA resource name out=w2006:refnum<visa-resource-name>, error out=w2005:errorcluster)  [unwired: 1 out]
                n1102 = VISA Close(VISA resource name=w2006, error in (no error)=w2005) -> ()  [unwired: 1 out]
              }
            }
            n1103 = Concatenate Strings("set units 4", "\r") -> (w1955:string)
            n1104 = Number To Decimal String(number="Normal \nVolume (ul)") -> (decimal integer string=w1966:string)  [unwired: 1 in]
            n1105 = Concatenate Strings("set volume", w1966, "\r") -> (w1964:string)
          }
          event "Normal \nRate (ul/hr)": Value Change {
            n1106 = event-data() -> ()  [unwired: 1 in, 5 out]
            n1107 = call-poly "VISA Configure Serial Port"("VISA resource name"=w2014) -> ("VISA resource name out"=w2022:refnum<visa-resource-name>, "error out"=w2021:errorcluster)  [unwired: 13 in]
            n1108 = local read "Write Wait"() -> (w2012:i32)
            n1109 = Concatenate Strings("enter pump1", "\r") -> (w2024:string)
            n1110 = flat-sequence {
              tunnel: w2021 -> [w2041]
              tunnel: w2022 -> [w2043]
              tunnel: [w2042] -> w2037
              tunnel: [w2040] -> w2036
              tunnel: w2024 -> [w2039]
              tunnel: w2037 -> [w2046]
              tunnel: [w2046] -> w2035
              tunnel: w2036 -> [w2045]
              tunnel: [w2045] -> w2034
              tunnel: w2012 -> [w2044]
              tunnel: w2035 -> [w2050]
              tunnel: [w2051] -> w2033
              tunnel: w2034 -> [w2049]
              tunnel: [w2048] -> w2032
              tunnel: w2015 -> [w2047]
              tunnel: w2033 -> [w2054]
              tunnel: w2032 -> [w2053]
              tunnel: [w2054] -> w2031
              tunnel: [w2053] -> w2030
              tunnel: w2012 -> [w2052]
              tunnel: [w2059] -> w2029
              tunnel: [w2058] -> w2028
              tunnel: w2031 -> [w2057]
              tunnel: w2030 -> [w2056]
              tunnel: w2018 -> [w2055]
              tunnel: w2029 -> [w2062]
              tunnel: [w2062] -> w2027
              tunnel: w2028 -> [w2061]
              tunnel: [w2061] -> w2026
              tunnel: w2012 -> [w2060]
              tunnel: w2027 -> [w2066]
              tunnel: w2026 -> [w2065]
              frame #0 {
                n1111 = VISA Write(VISA resource name=w2043, write buffer=w2039, error in (no error)=w2041) -> (VISA resource name out=w2042:refnum<visa-resource-name>, error out=w2040:errorcluster)  [unwired: 1 out]
              }
              frame #1 {
                n1112 = Wait (ms)(milliseconds to wait=w2044) -> ()  [unwired: 1 out]
              }
              frame #2 {
                n1113 = VISA Write(VISA resource name=w2050, write buffer=w2047, error in (no error)=w2049) -> (VISA resource name out=w2051:refnum<visa-resource-name>, error out=w2048:errorcluster)  [unwired: 1 out]
              }
              frame #3 {
                n1114 = Wait (ms)(milliseconds to wait=w2052) -> ()  [unwired: 1 out]
              }
              frame #4 {
                n1115 = VISA Write(VISA resource name=w2057, write buffer=w2055, error in (no error)=w2056) -> (VISA resource name out=w2059:refnum<visa-resource-name>, error out=w2058:errorcluster)  [unwired: 1 out]
              }
              frame #5 {
                n1116 = Wait (ms)(milliseconds to wait=w2060) -> ()  [unwired: 1 out]
              }
              frame #6 {
                n1117 = Concatenate Strings("enter main ", "\r") -> (w2067:string)
                n1118 = VISA Write(VISA resource name=w2066, write buffer=w2067, error in (no error)=w2065) -> (VISA resource name out=w2064:refnum<visa-resource-name>, error out=w2063:errorcluster)  [unwired: 1 out]
                n1119 = VISA Close(VISA resource name=w2064, error in (no error)=w2063) -> ()  [unwired: 1 out]
              }
            }
            n1120 = Concatenate Strings("set units 4", "\r") -> (w2015:string)
            n1121 = Number To Decimal String(number="Normal \nRate (ul/hr)") -> (decimal integer string=w2013:string)  [unwired: 1 in]
            n1122 = Concatenate Strings("set rate", w2013, "\r") -> (w2018:string)
          }
          event "Normal \nRate (ul/hr)  2": Value Change {
            n1123 = event-data() -> ()  [unwired: 1 in, 5 out]
            n1124 = call-poly "VISA Configure Serial Port"("VISA resource name"=w2072) -> ("VISA resource name out"=w2080:refnum<visa-resource-name>, "error out"=w2079:errorcluster)  [unwired: 13 in]
            n1125 = local read "Write Wait"() -> (w2070:i32)
            n1126 = Concatenate Strings("enter pump2", "\r") -> (w2082:string)
            n1127 = flat-sequence {
              tunnel: w2079 -> [w2099]
              tunnel: w2080 -> [w2101]
              tunnel: [w2100] -> w2095
              tunnel: [w2098] -> w2094
              tunnel: w2082 -> [w2097]
              tunnel: w2095 -> [w2104]
              tunnel: [w2104] -> w2093
              tunnel: w2094 -> [w2103]
              tunnel: [w2103] -> w2092
              tunnel: w2070 -> [w2102]
              tunnel: w2093 -> [w2108]
              tunnel: [w2109] -> w2091
              tunnel: w2092 -> [w2107]
              tunnel: [w2106] -> w2090
              tunnel: w2073 -> [w2105]
              tunnel: w2091 -> [w2112]
              tunnel: w2090 -> [w2111]
              tunnel: [w2112] -> w2089
              tunnel: [w2111] -> w2088
              tunnel: w2070 -> [w2110]
              tunnel: [w2117] -> w2087
              tunnel: [w2116] -> w2086
              tunnel: w2089 -> [w2115]
              tunnel: w2088 -> [w2114]
              tunnel: w2076 -> [w2113]
              tunnel: w2087 -> [w2120]
              tunnel: [w2120] -> w2085
              tunnel: w2086 -> [w2119]
              tunnel: [w2119] -> w2084
              tunnel: w2070 -> [w2118]
              tunnel: w2085 -> [w2124]
              tunnel: w2084 -> [w2123]
              frame #0 {
                n1128 = VISA Write(VISA resource name=w2101, write buffer=w2097, error in (no error)=w2099) -> (VISA resource name out=w2100:refnum<visa-resource-name>, error out=w2098:errorcluster)  [unwired: 1 out]
              }
              frame #1 {
                n1129 = Wait (ms)(milliseconds to wait=w2102) -> ()  [unwired: 1 out]
              }
              frame #2 {
                n1130 = VISA Write(VISA resource name=w2108, write buffer=w2105, error in (no error)=w2107) -> (VISA resource name out=w2109:refnum<visa-resource-name>, error out=w2106:errorcluster)  [unwired: 1 out]
              }
              frame #3 {
                n1131 = Wait (ms)(milliseconds to wait=w2110) -> ()  [unwired: 1 out]
              }
              frame #4 {
                n1132 = VISA Write(VISA resource name=w2115, write buffer=w2113, error in (no error)=w2114) -> (VISA resource name out=w2117:refnum<visa-resource-name>, error out=w2116:errorcluster)  [unwired: 1 out]
              }
              frame #5 {
                n1133 = Wait (ms)(milliseconds to wait=w2118) -> ()  [unwired: 1 out]
              }
              frame #6 {
                n1134 = Concatenate Strings("enter main ", "\r") -> (w2125:string)
                n1135 = VISA Write(VISA resource name=w2124, write buffer=w2125, error in (no error)=w2123) -> (VISA resource name out=w2122:refnum<visa-resource-name>, error out=w2121:errorcluster)  [unwired: 1 out]
                n1136 = VISA Close(VISA resource name=w2122, error in (no error)=w2121) -> ()  [unwired: 1 out]
              }
            }
            n1137 = Concatenate Strings("set units 4", "\r") -> (w2073:string)
            n1138 = Number To Decimal String(number="Normal \nRate (ul/hr)  2") -> (decimal integer string=w2071:string)  [unwired: 1 in]
            n1139 = Concatenate Strings("set rate", w2071, "\r") -> (w2076:string)
          }
          event "Normal \nVolume (ul) 2": Value Change {
            n1140 = event-data() -> ()  [unwired: 1 in, 5 out]
            n1141 = call-poly "VISA Configure Serial Port"("VISA resource name"=w2131) -> ("VISA resource name out"=w2135:refnum<visa-resource-name>, "error out"=w2136:errorcluster)  [unwired: 13 in]
            n1142 = local read "Write Wait"() -> (w2128:i32)
            n1143 = Concatenate Strings("enter pump2", "\r") -> (w2133:string)
            n1144 = flat-sequence {
              tunnel: w2136 -> [w2157]
              tunnel: w2135 -> [w2159]
              tunnel: [w2158] -> w2154
              tunnel: [w2156] -> w2153
              tunnel: w2133 -> [w2155]
              tunnel: w2154 -> [w2162]
              tunnel: [w2162] -> w2152
              tunnel: w2153 -> [w2161]
              tunnel: [w2161] -> w2151
              tunnel: w2128 -> [w2160]
              tunnel: w2152 -> [w2166]
              tunnel: [w2167] -> w2150
              tunnel: w2151 -> [w2165]
              tunnel: [w2164] -> w2149
              tunnel: w2142 -> [w2163]
              tunnel: w2150 -> [w2170]
              tunnel: w2149 -> [w2169]
              tunnel: [w2170] -> w2148
              tunnel: [w2169] -> w2147
              tunnel: w2128 -> [w2168]
              tunnel: [w2175] -> w2146
              tunnel: [w2174] -> w2145
              tunnel: w2148 -> [w2173]
              tunnel: w2147 -> [w2172]
              tunnel: w2139 -> [w2171]
              tunnel: w2146 -> [w2178]
              tunnel: [w2178] -> w2144
              tunnel: w2145 -> [w2177]
              tunnel: [w2177] -> w2143
              tunnel: w2128 -> [w2176]
              tunnel: w2144 -> [w2182]
              tunnel: w2143 -> [w2181]
              frame #0 {
                n1145 = VISA Write(VISA resource name=w2159, write buffer=w2155, error in (no error)=w2157) -> (VISA resource name out=w2158:refnum<visa-resource-name>, error out=w2156:errorcluster)  [unwired: 1 out]
              }
              frame #1 {
                n1146 = Wait (ms)(milliseconds to wait=w2160) -> ()  [unwired: 1 out]
              }
              frame #2 {
                n1147 = VISA Write(VISA resource name=w2166, write buffer=w2163, error in (no error)=w2165) -> (VISA resource name out=w2167:refnum<visa-resource-name>, error out=w2164:errorcluster)  [unwired: 1 out]
              }
              frame #3 {
                n1148 = Wait (ms)(milliseconds to wait=w2168) -> ()  [unwired: 1 out]
              }
              frame #4 {
                n1149 = VISA Write(VISA resource name=w2173, write buffer=w2171, error in (no error)=w2172) -> (VISA resource name out=w2175:refnum<visa-resource-name>, error out=w2174:errorcluster)  [unwired: 1 out]
              }
              frame #5 {
                n1150 = Wait (ms)(milliseconds to wait=w2176) -> ()  [unwired: 1 out]
              }
              frame #6 {
                n1151 = Concatenate Strings("enter main ", "\r") -> (w2183:string)
                n1152 = VISA Write(VISA resource name=w2182, write buffer=w2183, error in (no error)=w2181) -> (VISA resource name out=w2180:refnum<visa-resource-name>, error out=w2179:errorcluster)  [unwired: 1 out]
                n1153 = VISA Close(VISA resource name=w2180, error in (no error)=w2179) -> ()  [unwired: 1 out]
              }
            }
            n1154 = Concatenate Strings("set units 4", "\r") -> (w2142:string)
            n1155 = Number To Decimal String(number="Normal \nVolume (ul) 2") -> (decimal integer string=w2129:string)  [unwired: 1 in]
            n1156 = Concatenate Strings("set volume", w2129, "\r") -> (w2139:string)
          }
        }
        n1157 = node-c288() -> ()  [unwired: 1 in, 1 out]
      }
      n1158 = node-c288(w1515) -> ()  [unwired: 1 out]
    }
    frame Enabled {
      n1159 = node-c288(2 ("Processor")) -> (w2195:T12)  [unwired: 3 in]
      n1160 = timed-loop "Pump Control" {
        timing: w2195 -> [_]
        timing-out: [_] -> w2194
        tunnel: refnum<visa-resource-name> "COM5" ("VISA resource name") -> [w2197]
        stop <- w2196 stop-if-true
        n1161 = node-c288() -> ()  [unwired: 1 in, 1 out]
        n1162 = event shown="[2] \"Inject Sample\": Value Change" {
          selector: _ -> [_ _ _ _ _]
          dyn-events: _ -> [_ _ _ _ _]
          timeout: _ -> [_ _ _ _ _]
          tunnel: w2197 -> [w2203 _ w2277 w2304 w2309]
          tunnel: [_ w2275 _ _ _] -> w2196
          event "Flush Sample": Value Change {
            n1163 = event-data() -> ()  [unwired: 1 in, 5 out]
            n1164 = local read "Write Wait"() -> (w2217:i32)
            n1165 = flat-sequence {
              tunnel: [w2241] -> w2237
              tunnel: [w2240] -> w2236
              tunnel: "CLD" -> [w2239]
              tunnel: w2203 -> [w2238]
              tunnel: w2237 -> [w2244]
              tunnel: [w2244] -> w2235
              tunnel: w2236 -> [w2243]
              tunnel: [w2243] -> w2234
              tunnel: w2217 -> [w2242]
              tunnel: [w2249] -> w2233
              tunnel: [w2246] -> w2232
              tunnel: w2235 -> [w2248]
              tunnel: w2234 -> [w2247]
              tunnel: "MODVOL" -> [w2245]
              tunnel: w2233 -> [w2252]
              tunnel: [w2252] -> w2231
              tunnel: [w2251] -> w2230
              tunnel: w2232 -> [w2251]
              tunnel: w2217 -> [w2250]
              tunnel: w2231 -> [w2257]
              tunnel: [w2256] -> w2229
              tunnel: w2219 -> [w2255]
              tunnel: w2230 -> [w2254]
              tunnel: [w2253] -> w2228
              tunnel: w2229 -> [w2260]
              tunnel: [w2260] -> w2227
              tunnel: [w2259] -> w2226
              tunnel: w2228 -> [w2259]
              tunnel: w2217 -> [w2258]
              tunnel: w2227 -> [w2265]
              tunnel: [w2264] -> w2225
              tunnel: w2221 -> [w2263]
              tunnel: w2226 -> [w2262]
              tunnel: [w2261] -> w2224
              tunnel: [w2268] -> w2222
              tunnel: w2225 -> [w2268]
              tunnel: [w2267] -> w2223
              tunnel: w2224 -> [w2267]
              tunnel: w2217 -> [w2266]
              tunnel: w2223 -> [w2273]
              tunnel: w2222 -> [w2274]
              tunnel: [w2272] -> w2212
              tunnel: "RUN " -> [w2271]
              frame #0 {
                n1166 = call "Write to pump 2.vi"("String to write"=w2239, "VISA resource name"=w2238) -> ("error out"=w2240:errorcluster, "VISA resource name out"=w2241:refnum<visa-resource-name>)  [unwired: 8 in]
              }
              frame #1 {
                n1167 = Wait (ms)(milliseconds to wait=w2242) -> ()  [unwired: 1 out]
              }
              frame #2 {
                n1168 = call "Write to pump 2.vi"("error in (no error)"=w2247, "String to write"=w2245, "VISA resource name"=w2248) -> ("error out"=w2246:errorcluster, "VISA resource name out"=w2249:refnum<visa-resource-name>)  [unwired: 7 in]
              }
              frame #3 {
                n1169 = Wait (ms)(milliseconds to wait=w2250) -> ()  [unwired: 1 out]
              }
              frame #4 {
                n1170 = call "Write to pump 2.vi"("error in (no error)"=w2254, "String to write"=w2255, "VISA resource name"=w2257) -> ("error out"=w2253:errorcluster, "VISA resource name out"=w2256:refnum<visa-resource-name>)  [unwired: 7 in]
              }
              frame #5 {
                n1171 = Wait (ms)(milliseconds to wait=w2258) -> ()  [unwired: 1 out]
              }
              frame #6 {
                n1172 = call "Write to pump 2.vi"("error in (no error)"=w2262, "String to write"=w2263, "VISA resource name"=w2265) -> ("error out"=w2261:errorcluster, "VISA resource name out"=w2264:refnum<visa-resource-name>)  [unwired: 7 in]
              }
              frame #7 {
                n1173 = Wait (ms)(milliseconds to wait=w2266) -> ()  [unwired: 1 out]
              }
              frame #8 {
                w2270 = TRUE ("Inject Pump 3")
                n1174 = Tick Count (ms)() -> (millisecond timer value=→"Flush Sample Start Time":u32)
                n1175 = call "Write to pump 2.vi"("error in (no error)"=w2273, "String to write"=w2271, "VISA resource name"=w2274) -> ("error out"=w2272:errorcluster)  [unwired: 7 in, 1 out]
                n1176 = local write "Inject Sample"(w2270) -> ()
                "Flushing Sample" <- w2270
              }
            }
            n1177 = Number To Fractional String(number="Flush \nRate (ul/min)  3") -> (F-format string=w2205:string)  [unwired: 3 in]
            n1178 = String Subset(string=w2205, length (rest)=6 ("length (rest)")) -> (substring=w2204:string)  [unwired: 1 in]
            n1179 = Concatenate Strings("RAT", w2204, "UM") -> (w2219:string)
            n1180 = Divide(x="Flush\nVolume (ul)  3", y=1000.0) -> (x/y=w2210:dbl)
            n1181 = Number To Fractional String(number=w2210) -> (F-format string=w2209:string)  [unwired: 3 in]
            n1182 = Divide(x="Flush\nVolume (ul)  3", y="Flush \nRate (ul/min)  3") -> (x/y=w2200:dbl)
            n1183 = Multiply(x=w2200, y=60.0) -> (x*y=→"Sample flush time (s)":dbl)
            n1184 = String Subset(string=w2209, length (rest)=6 ("length (rest)")) -> (substring=w2208:string)  [unwired: 1 in]
            n1185 = Concatenate Strings("TGT", w2208) -> (w2221:string)
            "error out" <- w2212
          }
          event "Stop": Value Change {
            n1186 = event-data() -> ()  [unwired: 1 in, 5 out]
            n1187 = local read "Stop"() -> (w2275:bool)
          }
          event "Inject Sample": Value Change {
            n1188 = event-data() -> ()  [unwired: 1 in, 5 out]
            n1189 = case shown="True" "Inject Sample" {
              tunnel: w2277 -> [w2279 w2280]
              frame False {
                n1190 = call "Write to pump 2.vi"("String to write"="STP", "VISA resource name"=w2279) -> ()  [unwired: 8 in, 2 out]
              }
              frame True {
                n1191 = local read "Normal \nRate (ul/hr)  3"() -> (w2281:dbl)
                n1192 = Number To Fractional String(number=w2281) -> (F-format string=w2284:string)  [unwired: 3 in]
                n1193 = String Subset(string=w2284, length (rest)=6 ("length (rest)")) -> (substring=w2282:string)  [unwired: 1 in]
                n1194 = flat-sequence {
                  tunnel: "RUN " -> [w2296]
                  tunnel: [w2298] -> _
                  tunnel: [w2297] -> _
                  tunnel: w2280 -> [w2295]
                  frame #0 {
                    n1195 = call "Write to pump 2.vi"("String to write"=w2296, "VISA resource name"=w2295) -> ("error out"=w2297:errorcluster, "VISA resource name out"=w2298:refnum<visa-resource-name>)  [unwired: 8 in]
                  }
                }
                n1196 = Concatenate Strings("RAT", w2282, "UH" ("string")) -> ()  [unwired: 1 out]
                n1197 = local read "Normal \nVolume (ul) 3"() -> (w2290:dbl)
                n1198 = Divide(x=w2290, y=1000.0) -> (x/y=w2285:dbl)
                n1199 = Number To Fractional String(number=w2285) -> (F-format string=w2288:string)  [unwired: 3 in]
                n1200 = String Subset(string=w2288, length (rest)=6 ("length (rest)")) -> (substring=w2286:string)  [unwired: 1 in]
                n1201 = Concatenate Strings("TGT", w2286) -> ()  [unwired: 1 out]
              }
            }
          }
          event "Normal \nRate (ul/hr)  3": Value Change {
            n1202 = event-data() -> ()  [unwired: 1 in, 5 out]
            n1203 = Number To Fractional String(number="Normal \nRate (ul/hr)  3") -> (F-format string=w2302:string)  [unwired: 3 in]
            n1204 = String Subset(string=w2302, length (rest)=6 ("length (rest)")) -> (substring=w2300:string)  [unwired: 1 in]
            n1205 = Concatenate Strings("RAT", w2300, "UH") -> (w2303:string)
            n1206 = call "Write to pump 2.vi"("String to write"=w2303, "VISA resource name"=w2304) -> ()  [unwired: 8 in, 2 out]
          }
          event "Clear Volume": Value Change {
            n1207 = event-data() -> ()  [unwired: 1 in, 5 out]
            n1208 = Divide(x="Normal \nVolume (ul) 3", y=1000.0) -> (x/y=w2322:dbl)
            n1209 = Number To Fractional String(number=w2322) -> (F-format string=w2325:string)  [unwired: 3 in]
            n1210 = String Subset(string=w2325, length (rest)=6 ("length (rest)")) -> (substring=w2323:string)  [unwired: 1 in]
            n1211 = flat-sequence {
              tunnel: [w2332] -> w2320
              tunnel: [w2331] -> w2319
              tunnel: w2309 -> [w2330]
              tunnel: w2308 -> [w2329]
              tunnel: [w2334] -> w2317
              tunnel: [w2333] -> w2318
              tunnel: w2314 -> [w2335]
              tunnel: w2320 -> [w2334]
              tunnel: w2319 -> [w2333]
              tunnel: w2318 -> [w2339]
              tunnel: w2317 -> [w2340]
              tunnel: [w2338] -> _
              tunnel: [w2337] -> _
              tunnel: w2307 -> [w2336]
              frame #0 {
                n1212 = call "Write to pump 2.vi"("String to write"=w2329, "VISA resource name"=w2330) -> ("error out"=w2331:errorcluster, "VISA resource name out"=w2332:refnum<visa-resource-name>)  [unwired: 8 in]
              }
              frame #1 {
                n1213 = Wait (ms)(milliseconds to wait=w2335) -> ()  [unwired: 1 out]
              }
              frame #2 {
                n1214 = call "Write to pump 2.vi"("error in (no error)"=w2339, "String to write"=w2336, "VISA resource name"=w2340) -> ("error out"=w2337:errorcluster, "VISA resource name out"=w2338:refnum<visa-resource-name>)  [unwired: 7 in]
              }
            }
            n1215 = local read "Write Wait"() -> (w2314:i32)
            n1216 = Concatenate Strings("TGT", w2323) -> (w2308:string)
            n1217 = local read "Normal \nRate (ul/hr)  3"() -> (w2310:dbl)
            n1218 = local write "Clear Volume"(FALSE ("Clear Volume")) -> ()
            n1219 = Number To Fractional String(number=w2310) -> (F-format string=w2313:string)  [unwired: 3 in]
            n1220 = String Subset(string=w2313, length (rest)=6 ("length (rest)")) -> (substring=w2311:string)  [unwired: 1 in]
            n1221 = Concatenate Strings("RAT", w2311, "UH" ("string")) -> (w2307:string)
          }
        }
        n1222 = node-c288() -> ()  [unwired: 1 in, 1 out]
      }
      n1223 = node-c288(w2194) -> ()  [unwired: 1 out]
    }
  }
  n1224 = node-c288() -> (w84:T12)  [unwired: 4 in]
  n1225 = timed-loop {
    timing: w84 -> [_]
    timing-out: [_] -> w83
    stop <- w2347 stop-if-true
    n1226 = node-c288() -> ()  [unwired: 1 in, 1 out]
    n1227 = event shown="[1] \"Stop\": Value Change" {
      selector: _ -> [_ _]
      dyn-events: _ -> [_ _]
      timeout: _ -> [_ _]
      tunnel: [_ "Stop"] -> w2347
      event Timeout {
        n1228 = event-data() -> ()  [unwired: 1 in, 2 out]
      }
      event "Stop": Value Change {
        n1229 = event-data() -> ()  [unwired: 1 in, 4 out]
        n1230 = local write "Force Feedback"(FALSE ("Force Feedback")) -> ()
      }
    }
    n1231 = node-c288() -> ()  [unwired: 1 in, 1 out]
  }
  n1232 = case shown="True" w73 {
    tunnel: w78 -> [_ w2354]
    tunnel: w77 -> [_ w2353]
    tunnel: w76 -> [_ w2352]
    frame False {
    }
    frame True {
      w2356 = T15 3 items=["no dialog", "OK message", "continue or stop message", "OK message + warnings", "continue/stop + warnings"] ("type of dialog (OK msg:1)")
      w2355 = T15 3 items=["no dialog", "OK message", "continue or stop message", "OK message + warnings", "continue/stop + warnings"] ("type of dialog (OK msg:1)")
      n1233 = call <vilib>:"DAQmx Clear Task.vi"("task in"=w2354, "error in"=w2352) -> ("error out"=w2357:errorcluster)  [unwired: 13 in]
      n1234 = call <vilib>:"DAQmx Clear Task.vi"("task in"=w2353) -> ("error out"=w2358:errorcluster)  [unwired: 14 in]
      n1235 = call <vilib>:"Simple Error Handler.vi"("type of dialog (OK msg:1)"=w2356, "error in (no error)"=w2357) -> ()  [unwired: 3 in, 5 out]
      n1236 = call <vilib>:"Simple Error Handler.vi"("type of dialog (OK msg:1)"=w2355, "error in (no error)"=w2358) -> ()  [unwired: 3 in, 5 out]
    }
  }
  n1237 = case shown="\"Force Feedback\", Default" "?" {
    frame "Force Feedback", Default {
    }
    frame "Raster scan" {
    }
  }
  n1238 = node-c288(w83) -> ()  [unwired: 1 out]
  n1239 = node-c288(w86) -> ()  [unwired: 1 out]
  n1240 = local write "Pause Mouse/Mirror Connection"(FALSE ("Pause Mouse/Mirror Connection")) -> ()
  n1241 = local write "Stop"(FALSE ("Stop all")) -> ()
  "CoordinatesMousePressed" <- T4 {"Horizontal"=0, "Vertical"=0} ("Coords when pressed")
  "Deflection" <- T4 {"Horizontal"=0, "Vertical"=0} ("Coords when pressed")
